vi "CAEN_HVChannel.ProcCases.vi"(0 "i ref in":refnum<vi>, 1 "selector":string, 2 "Data":T1, 3 "call cluster":T2={"Object"="", "Selector"="", "CallType"=enum."synchronous", "Async Object"="", "Async Selector"="", "Data Descriptor"="", "Data"=[], "Error #"=0, "Expire"=0}, 5 "error in (no error)":errorcluster) -> (14 "i ref out":refnum<vi>, 17 "answer cluster":T2={"Object"="", "Selector"="", "CallType"=enum."synchronous", "Async Object"="", "Async Selector"="", "Data Descriptor"="", "Data"=[], "Error #"=0, "Expire"=0}, 19 "error out":errorcluster)   [LabVIEW 2014, in "CAEN_HVChannel.lvlib"]
doc: "This method is called by a process from within the default case in the event loop. The methods of a class that are linked to events will be called from THIS method. Add your code here."
uses:
  CAEN_HVChannel.lvlib
  CS_Core/CSSystem/CoreDefs/CoreDefs.call_type.ctl
  CS_Core/BaseProcess/BaseProcess.descriptor string definition.ctl
  CS_Core/CSSystem/CoreDefs/CoreDefs.rawDataType.ctl
  CS_Core/CSApplicationBaseClasses/PSChannelBase/PSChannelBase.directionType.ctl
  CS_Core/CSApplicationBaseClasses/PSChannelBase/PSChannelBase.serviceType.ctl
  CS_Core/CSSystem/CoreDefs/CoreDefs.error_type.ctl
  CS_Core/CSSystem/CoreDefs/CoreDefs.error_severity.ctl
  CSlibraries/UtilityLib/UtilityLib.valueStatus.ctl
  CS_Core/CSSystem/CoreLib/CoreLib.byte array 2 double.vi
  CS_Core/CSSystem/CoreLib/CoreLib.string 2 byte array.vi
  CS_Core/CSSystem/CoreLib/CoreLib.double 2 byte array.vi
  CS_Core/CSSystem/CoreLib/CoreLib.short 2 byte array.vi
  CS_Core/CSSystem/CoreLib/CoreLib.byte array 2 short.vi
  CS_Core/CSSystem/CoreLib/CoreLib.byte array 2 int.vi
  CS_Core/CSSystem/CoreLib/CoreLib.byte array 2 string.vi
  CS_Core/CSSystem/CoreLib/CoreLib.lvlib
  CS_Core/BaseProcess/BaseProcess.lvlib
  CS_Core/CSApplicationBaseClasses/PSChannelBase/PSChannelBase.lvlib
  CS_Core/CAEObj/CAEObj.lvlib
  CS_Core/CSApplicationBaseClasses/DeviceBase/DeviceBase.lvlib
  CAEN_HVSystem/CAEN_HVSystem.lvlib
  CSlibraries/UtilityLib/UtilityLib.lvlib
  CSlibraries-extern/DimLVEvent/LVDimInterface/LVDimInterface.lvlib
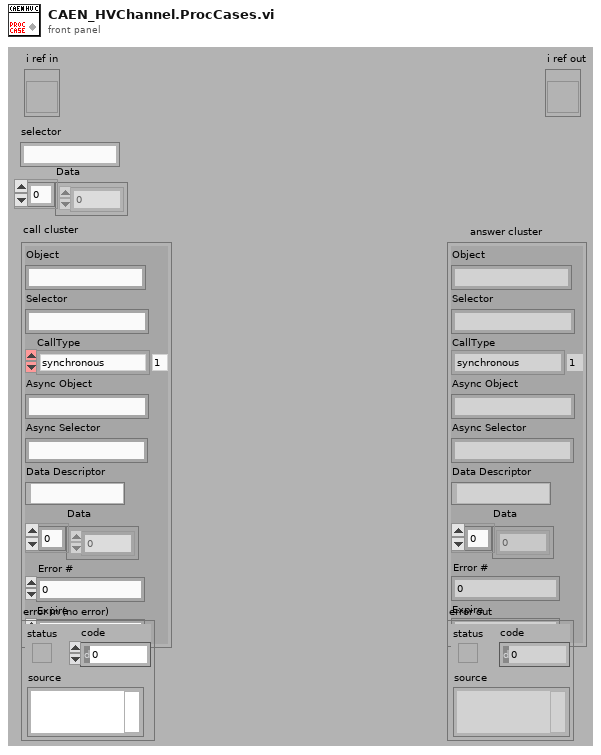
[diagram p1: front panel]
types:
  T1 = typedef "CoreDefs.rawDataType.ctl" = i8[]
  T2 = typedef "CoreDefs.call_type.ctl" = cluster{"Object":string, "Selector":string, "CallType":enum16{"simple", "synchronous", "asynchronous"}, "Async Object":string, "Async Selector":string, "Data Descriptor":T3, "Data":T1, "Error #":i32, "Expire":u32}
  T3 = typedef "BaseProcess.lvlib/BaseProcess.descriptor string definition.ctl" = string
  T4 = typedef "PSChannelBase.lvlib/PSChannelBase.serviceType.ctl" = enum16{"onOff", "voltage", "current", "tripCurrent", "rampUpSpeed", "rampDownSpeed", "status"}
  T5 = typedef "PSChannelBase.lvlib/PSChannelBase.directionType.ctl" = enum16{"unknown", "update actual value", "update nominal value", "update both"}
  T6 = typedef "CoreDefs.error_severity.ctl" = enum16{"undefined", "information", "warning", "error", "fatal"}
  T7 = typedef "CoreDefs.error_type.ctl" = enum16{"no error", "can't load process", "can't unload process", "process does not exist", "can't install process", "can't remove process", "unknown function", "time out", "can't execute function", "duplicate queue name", "super not found", "caller queue invalid", "can't ping process", "unknown error", "VISA Error", "VISA timeout", "GPIB timeout", "GPIB error", "communication error", "data type mismatch", "can't read data from OPC server", "can't write data to OPC server", "OET error", "function not implemented", "process already exists", "invalid Shared Variable name", "error writing Shared Variable", "error reading Shared Variable", "invalid client name", "corrupt database", "unknown class", "call not authorized", "parameter out of range", "OET timeout: can't get data to modify", "invalid queue name", "requested operation incompatible with current state", "event undefined", "event disabled", "state undefined", "caller is not a friend", "EventBuilder: bad eventID", "EventBuilder: no DAQ devices", "a thread must not stop itself", "UNUSED ELEMENT4", "DiscArchiver: eventData incomplete", "DiscArchiver: eventData does not belong to run", "DiscArchiver: can't open file", "DiscArchiver: can't write to file", "DiscArchiver: available disc space low", "can't acquire semaphore", "error reading data from database", "notifier object is not existing", "can't register process", "can't unregister process", "illegal event type", "object disabled", "object already exists", "can't change state", "Instrument not found", "no connection to remote node", "invalid reference", "N/A", "UNUSED ELEMENT 1", "element not found", "illegal TCP/IP connection detected", "object does not exist", "invalid access ID", "unknown CS system", "invalid privilige", "unsupported data type", "unsupported server type", "IO server already exists", "Shared Variable already exists"}
  T8 = typedef "UtilityLib.lvlib/UtilityLib.valueStatus.ctl" = enum16{"no info available", "stand by/off", "on", "warning", "alarm/malfunction", "not implemented", "user action required", "important information", "system default", "control default", "indicator default", "button default"}
  T9 = typedef "CAEN_HVChannel.lvlib/CAEN_HVChannel.i attribute.ctl" = cluster{"Channel Array":cluster{"Logical Name":string, "Address":string, "error in (no error)":errorcluster, "Name":cluster{"Name":string, "DIM Status":cluster{"no link":bool, "quality":i32, "Time Stamp":timestamp}}, "Status":cluster{"Status":i16, "DIM Status":cluster{"no link":bool, "quality":i32, "Time Stamp":timestamp}}, "V0Set":cluster{"V0Set#EU":cluster{"V0Set#EU":string, "DIM Status":cluster{"no link":bool, "quality":i32, "Time Stamp":timestamp}}, "V0Set":cluster{"V0Set":dbl, "DIM Status":cluster{"no link":bool, "quality":i32, "Time Stamp":timestamp}}, "V0Set#HighEU":cluster{"V0Set#HighEU":dbl, "DIM Status":cluster{"no link":bool, "quality":i32, "Time Stamp":timestamp}}, "V0Set#LowEU":cluster{"V0Set#LowEU":dbl, "DIM Status":cluster{"no link":bool, "quality":i32, "Time Stamp":timestamp}}, "V0Set#Multiplier":dbl}, "I0Set":cluster{"I0Set#EU":cluster{"I0Set#EU":string, "DIM Status":cluster{"no link":bool, "quality":i32, "Time Stamp":timestamp}}, "I0Set":cluster{"I0Set":dbl, "DIM Status":cluster{"no link":bool, "quality":i32, "Time Stamp":timestamp}}, "I0Set#HighEU":cluster{"I0Set#HighEU":dbl, "DIM Status":cluster{"no link":bool, "quality":i32, "Time Stamp":timestamp}}, "I0Set#LowEU":cluster{"I0Set#LowEU":dbl, "DIM Status":cluster{"no link":bool, "quality":i32, "Time Stamp":timestamp}}, "I0Set#Multiplier":dbl}, "V1Set":cluster{"V1Set#EU":cluster{"V1Set#EU":string, "DIM Status":cluster{"no link":bool, "quality":i32, "Time Stamp":timestamp}}, "V1Set":cluster{"V1Set":dbl, "DIM Status":cluster{"no link":bool, "quality":i32, "Time Stamp":timestamp}}, "V1Set#HighEU":cluster{"V1Set#HighEU":dbl, "DIM Status":cluster{"no link":bool, "quality":i32, "Time Stamp":timestamp}}, "V1Set#LowEU":cluster{"V1Set#LowEU":dbl, "DIM Status":cluster{"no link":bool, "quality":i32, "Time Stamp":timestamp}}, "V1Set#Multiplier":dbl}, "I1Set":cluster{"I1Set#EU":cluster{"I1Set#EU":string, "DIM Status":cluster{"no link":bool, "quality":i32, "Time Stamp":timestamp}}, "I1Set":cluster{"I1Set":dbl, "DIM Status":cluster{"no link":bool, "quality":i32, "Time Stamp":timestamp}}, "I1Set#HighEU":cluster{"I1Set#HighEU":dbl, "DIM Status":cluster{"no link":bool, "quality":i32, "Time Stamp":timestamp}}, "I1Set#LowEU":cluster{"I1Set#LowEU":dbl, "DIM Status":cluster{"no link":bool, "quality":i32, "Time Stamp":timestamp}}, "I1Set#Multiplier":dbl}, "RUp":cluster{"RUp#EU":cluster{"RUp#EU":string, "DIM Status":cluster{"no link":bool, "quality":i32, "Time Stamp":timestamp}}, "RUp":cluster{"RUp":dbl, "DIM Status":cluster{"no link":bool, "quality":i32, "Time Stamp":timestamp}}, "RUp#HighEU":cluster{"RUp#HighEU":dbl, "DIM Status":cluster{"no link":bool, "quality":i32, "Time Stamp":timestamp}}, "RUp#LowEU":cluster{"RUp#LowEU":dbl, "DIM Status":cluster{"no link":bool, "quality":i32, "Time Stamp":timestamp}}, "RUp#Multiplier":dbl}, "RDWn":cluster{"RDWn#EU":cluster{"RDWn#EU":string, "DIM Status":cluster{"no link":bool, "quality":i32, "Time Stamp":timestamp}}, "RDWn":cluster{"RDWn":dbl, "DIM Status":cluster{"no link":bool, "quality":i32, "Time Stamp":timestamp}}, "RDWn#HighEU":cluster{"RDWn#HighEU":dbl, "DIM Status":cluster{"no link":bool, "quality":i32, "Time Stamp":timestamp}}, "RDWn#LowEU":cluster{"RDWn#LowEU":dbl, "DIM Status":cluster{"no link":bool, "quality":i32, "Time Stamp":timestamp}}, "RDWn#Multiplier":dbl}, "Trip":cluster{"Trip#EU":cluster{"Trip#EU":string, "DIM Status":cluster{"no link":bool, "quality":i32, "Time Stamp":timestamp}}, "Trip":cluster{"Trip":dbl, "DIM Status":cluster{"no link":bool, "quality":i32, "Time Stamp":timestamp}}, "Trip#HighEU":cluster{"Trip#HighEU":dbl, "DIM Status":cluster{"no link":bool, "quality":i32, "Time Stamp":timestamp}}, "Trip#LowEU":cluster{"Trip#LowEU":dbl, "DIM Status":cluster{"no link":bool, "quality":i32, "Time Stamp":timestamp}}, "Trip#Multiplier":dbl}, "SVMax":cluster{"SVMax#EU":cluster{"SVMax#EU":string, "DIM Status":cluster{"no link":bool, "quality":i32, "Time Stamp":timestamp}}, "SVMax":cluster{"SVMax":dbl, "DIM Status":cluster{"no link":bool, "quality":i32, "Time Stamp":timestamp}}, "SVMax#HighEU":cluster{"SVMax#HighEU":dbl, "DIM Status":cluster{"no link":bool, "quality":i32, "Time Stamp":timestamp}}, "SVMax#LowEU":cluster{"SVMax#LowEU":dbl, "DIM Status":cluster{"no link":bool, "quality":i32, "Time Stamp":timestamp}}, "SVMax#Multiplier":dbl}, "VMon":cluster{"VMon#EU":cluster{"VMon#EU":string, "DIM Status":cluster{"no link":bool, "quality":i32, "Time Stamp":timestamp}}, "VMon":cluster{"VMon":dbl, "DIM Status":cluster{"no link":bool, "quality":i32, "Time Stamp":timestamp}}, "VMon#HighEU":cluster{"VMon#HighEU":dbl, "DIM Status":cluster{"no link":bool, "quality":i32, "Time Stamp":timestamp}}, "VMon#LowEU":cluster{"VMon#LowEU":dbl, "DIM Status":cluster{"no link":bool, "quality":i32, "Time Stamp":timestamp}}, "VMon#Multiplier":dbl}, "IMon":cluster{"IMon#EU":cluster{"IMon#EU":string, "DIM Status":cluster{"no link":bool, "quality":i32, "Time Stamp":timestamp}}, "IMon":cluster{"IMon":dbl, "DIM Status":cluster{"no link":bool, "quality":i32, "Time Stamp":timestamp}}, "IMon#HighEU":cluster{"IMon#HighEU":dbl, "DIM Status":cluster{"no link":bool, "quality":i32, "Time Stamp":timestamp}}, "IMon#LowEU":cluster{"IMon#LowEU":dbl, "DIM Status":cluster{"no link":bool, "quality":i32, "Time Stamp":timestamp}}, "IMon#Multiplier":dbl}, "TripInt":cluster{"TripInt#EU":cluster{"TripInt#EU":string, "DIM Status":cluster{"no link":bool, "quality":i32, "Time Stamp":timestamp}}, "TripInt":cluster{"TripInt":dbl, "DIM Status":cluster{"no link":bool, "quality":i32, "Time Stamp":timestamp}}, "TripInt#HighEU":cluster{"TripInt#HighEU":dbl, "DIM Status":cluster{"no link":bool, "quality":i32, "Time Stamp":timestamp}}, "TripInt#LowEU":cluster{"TripInt#LowEU":dbl, "DIM Status":cluster{"no link":bool, "quality":i32, "Time Stamp":timestamp}}, "TripInt#Multiplier":dbl}, "TripExt":cluster{"TripExt#EU":cluster{"TripExt#EU":string, "DIM Status":cluster{"no link":bool, "quality":i32, "Time Stamp":timestamp}}, "TripExt":cluster{"TripExt":dbl, "DIM Status":cluster{"no link":bool, "quality":i32, "Time Stamp":timestamp}}, "TripExt#HighEU":cluster{"TripExt#HighEU":dbl, "DIM Status":cluster{"no link":bool, "quality":i32, "Time Stamp":timestamp}}, "TripExt#LowEU":cluster{"TripExt#LowEU":dbl, "DIM Status":cluster{"no link":bool, "quality":i32, "Time Stamp":timestamp}}, "TripExt#Multiplier":dbl}, "Pw":cluster{"Pw":cluster{"Pw":bool, "DIM Status":cluster{"no link":bool, "quality":i32, "Time Stamp":timestamp}}, "Pw#CoClose":cluster{"Pw#CoClose":string, "DIM Status":cluster{"no link":bool, "quality":i32, "Time Stamp":timestamp}}, "Pw#CoOpen":cluster{"Pw#CoOpen":string, "DIM Status":cluster{"no link":bool, "quality":i32, "Time Stamp":timestamp}}}, "POn":cluster{"POn":cluster{"POn":bool, "DIM Status":cluster{"no link":bool, "quality":i32, "Time Stamp":timestamp}}, "POn#CoClose":cluster{"POn#CoClose":string, "DIM Status":cluster{"no link":bool, "quality":i32, "Time Stamp":timestamp}}, "POn#CoOpen":cluster{"POn#CoOpen":string, "DIM Status":cluster{"no link":bool, "quality":i32, "Time Stamp":timestamp}}}, "PDwn":cluster{"PDwn":cluster{"PDwn":bool, "DIM Status":cluster{"no link":bool, "quality":i32, "Time Stamp":timestamp}}, "PDwn#CoClose":cluster{"PDwn#CoClose":string, "DIM Status":cluster{"no link":bool, "quality":i32, "Time Stamp":timestamp}}, "PDwn#CoOpen":cluster{"PDwn#CoOpen":string, "DIM Status":cluster{"no link":bool, "quality":i32, "Time Stamp":timestamp}}}, "DIM Service IDs":cluster{"nomV1Set":i32, "nomI1Set":i32, "nomTrip":i32, "nomSVMax":i32, "nomPOn":i32, "nomPDwn":i32, "nomTripInt":i32, "nomTripExt":i32}}[], "VoltageInRangeBand":dbl}
  T10 = cluster{"Logical Name":string, "Address":string, "error in (no error)":errorcluster, "Name":cluster{"Name":string, "DIM Status":cluster{"no link":bool, "quality":i32, "Time Stamp":timestamp}}, "Status":cluster{"Status":i16, "DIM Status":cluster{"no link":bool, "quality":i32, "Time Stamp":timestamp}}, "V0Set":cluster{"V0Set#EU":cluster{"V0Set#EU":string, "DIM Status":cluster{"no link":bool, "quality":i32, "Time Stamp":timestamp}}, "V0Set":cluster{"V0Set":dbl, "DIM Status":cluster{"no link":bool, "quality":i32, "Time Stamp":timestamp}}, "V0Set#HighEU":cluster{"V0Set#HighEU":dbl, "DIM Status":cluster{"no link":bool, "quality":i32, "Time Stamp":timestamp}}, "V0Set#LowEU":cluster{"V0Set#LowEU":dbl, "DIM Status":cluster{"no link":bool, "quality":i32, "Time Stamp":timestamp}}, "V0Set#Multiplier":dbl}, "I0Set":cluster{"I0Set#EU":cluster{"I0Set#EU":string, "DIM Status":cluster{"no link":bool, "quality":i32, "Time Stamp":timestamp}}, "I0Set":cluster{"I0Set":dbl, "DIM Status":cluster{"no link":bool, "quality":i32, "Time Stamp":timestamp}}, "I0Set#HighEU":cluster{"I0Set#HighEU":dbl, "DIM Status":cluster{"no link":bool, "quality":i32, "Time Stamp":timestamp}}, "I0Set#LowEU":cluster{"I0Set#LowEU":dbl, "DIM Status":cluster{"no link":bool, "quality":i32, "Time Stamp":timestamp}}, "I0Set#Multiplier":dbl}, "V1Set":cluster{"V1Set#EU":cluster{"V1Set#EU":string, "DIM Status":cluster{"no link":bool, "quality":i32, "Time Stamp":timestamp}}, "V1Set":cluster{"V1Set":dbl, "DIM Status":cluster{"no link":bool, "quality":i32, "Time Stamp":timestamp}}, "V1Set#HighEU":cluster{"V1Set#HighEU":dbl, "DIM Status":cluster{"no link":bool, "quality":i32, "Time Stamp":timestamp}}, "V1Set#LowEU":cluster{"V1Set#LowEU":dbl, "DIM Status":cluster{"no link":bool, "quality":i32, "Time Stamp":timestamp}}, "V1Set#Multiplier":dbl}, "I1Set":cluster{"I1Set#EU":cluster{"I1Set#EU":string, "DIM Status":cluster{"no link":bool, "quality":i32, "Time Stamp":timestamp}}, "I1Set":cluster{"I1Set":dbl, "DIM Status":cluster{"no link":bool, "quality":i32, "Time Stamp":timestamp}}, "I1Set#HighEU":cluster{"I1Set#HighEU":dbl, "DIM Status":cluster{"no link":bool, "quality":i32, "Time Stamp":timestamp}}, "I1Set#LowEU":cluster{"I1Set#LowEU":dbl, "DIM Status":cluster{"no link":bool, "quality":i32, "Time Stamp":timestamp}}, "I1Set#Multiplier":dbl}, "RUp":cluster{"RUp#EU":cluster{"RUp#EU":string, "DIM Status":cluster{"no link":bool, "quality":i32, "Time Stamp":timestamp}}, "RUp":cluster{"RUp":dbl, "DIM Status":cluster{"no link":bool, "quality":i32, "Time Stamp":timestamp}}, "RUp#HighEU":cluster{"RUp#HighEU":dbl, "DIM Status":cluster{"no link":bool, "quality":i32, "Time Stamp":timestamp}}, "RUp#LowEU":cluster{"RUp#LowEU":dbl, "DIM Status":cluster{"no link":bool, "quality":i32, "Time Stamp":timestamp}}, "RUp#Multiplier":dbl}, "RDWn":cluster{"RDWn#EU":cluster{"RDWn#EU":string, "DIM Status":cluster{"no link":bool, "quality":i32, "Time Stamp":timestamp}}, "RDWn":cluster{"RDWn":dbl, "DIM Status":cluster{"no link":bool, "quality":i32, "Time Stamp":timestamp}}, "RDWn#HighEU":cluster{"RDWn#HighEU":dbl, "DIM Status":cluster{"no link":bool, "quality":i32, "Time Stamp":timestamp}}, "RDWn#LowEU":cluster{"RDWn#LowEU":dbl, "DIM Status":cluster{"no link":bool, "quality":i32, "Time Stamp":timestamp}}, "RDWn#Multiplier":dbl}, "Trip":cluster{"Trip#EU":cluster{"Trip#EU":string, "DIM Status":cluster{"no link":bool, "quality":i32, "Time Stamp":timestamp}}, "Trip":cluster{"Trip":dbl, "DIM Status":cluster{"no link":bool, "quality":i32, "Time Stamp":timestamp}}, "Trip#HighEU":cluster{"Trip#HighEU":dbl, "DIM Status":cluster{"no link":bool, "quality":i32, "Time Stamp":timestamp}}, "Trip#LowEU":cluster{"Trip#LowEU":dbl, "DIM Status":cluster{"no link":bool, "quality":i32, "Time Stamp":timestamp}}, "Trip#Multiplier":dbl}, "SVMax":cluster{"SVMax#EU":cluster{"SVMax#EU":string, "DIM Status":cluster{"no link":bool, "quality":i32, "Time Stamp":timestamp}}, "SVMax":cluster{"SVMax":dbl, "DIM Status":cluster{"no link":bool, "quality":i32, "Time Stamp":timestamp}}, "SVMax#HighEU":cluster{"SVMax#HighEU":dbl, "DIM Status":cluster{"no link":bool, "quality":i32, "Time Stamp":timestamp}}, "SVMax#LowEU":cluster{"SVMax#LowEU":dbl, "DIM Status":cluster{"no link":bool, "quality":i32, "Time Stamp":timestamp}}, "SVMax#Multiplier":dbl}, "VMon":cluster{"VMon#EU":cluster{"VMon#EU":string, "DIM Status":cluster{"no link":bool, "quality":i32, "Time Stamp":timestamp}}, "VMon":cluster{"VMon":dbl, "DIM Status":cluster{"no link":bool, "quality":i32, "Time Stamp":timestamp}}, "VMon#HighEU":cluster{"VMon#HighEU":dbl, "DIM Status":cluster{"no link":bool, "quality":i32, "Time Stamp":timestamp}}, "VMon#LowEU":cluster{"VMon#LowEU":dbl, "DIM Status":cluster{"no link":bool, "quality":i32, "Time Stamp":timestamp}}, "VMon#Multiplier":dbl}, "IMon":cluster{"IMon#EU":cluster{"IMon#EU":string, "DIM Status":cluster{"no link":bool, "quality":i32, "Time Stamp":timestamp}}, "IMon":cluster{"IMon":dbl, "DIM Status":cluster{"no link":bool, "quality":i32, "Time Stamp":timestamp}}, "IMon#HighEU":cluster{"IMon#HighEU":dbl, "DIM Status":cluster{"no link":bool, "quality":i32, "Time Stamp":timestamp}}, "IMon#LowEU":cluster{"IMon#LowEU":dbl, "DIM Status":cluster{"no link":bool, "quality":i32, "Time Stamp":timestamp}}, "IMon#Multiplier":dbl}, "TripInt":cluster{"TripInt#EU":cluster{"TripInt#EU":string, "DIM Status":cluster{"no link":bool, "quality":i32, "Time Stamp":timestamp}}, "TripInt":cluster{"TripInt":dbl, "DIM Status":cluster{"no link":bool, "quality":i32, "Time Stamp":timestamp}}, "TripInt#HighEU":cluster{"TripInt#HighEU":dbl, "DIM Status":cluster{"no link":bool, "quality":i32, "Time Stamp":timestamp}}, "TripInt#LowEU":cluster{"TripInt#LowEU":dbl, "DIM Status":cluster{"no link":bool, "quality":i32, "Time Stamp":timestamp}}, "TripInt#Multiplier":dbl}, "TripExt":cluster{"TripExt#EU":cluster{"TripExt#EU":string, "DIM Status":cluster{"no link":bool, "quality":i32, "Time Stamp":timestamp}}, "TripExt":cluster{"TripExt":dbl, "DIM Status":cluster{"no link":bool, "quality":i32, "Time Stamp":timestamp}}, "TripExt#HighEU":cluster{"TripExt#HighEU":dbl, "DIM Status":cluster{"no link":bool, "quality":i32, "Time Stamp":timestamp}}, "TripExt#LowEU":cluster{"TripExt#LowEU":dbl, "DIM Status":cluster{"no link":bool, "quality":i32, "Time Stamp":timestamp}}, "TripExt#Multiplier":dbl}, "Pw":cluster{"Pw":cluster{"Pw":bool, "DIM Status":cluster{"no link":bool, "quality":i32, "Time Stamp":timestamp}}, "Pw#CoClose":cluster{"Pw#CoClose":string, "DIM Status":cluster{"no link":bool, "quality":i32, "Time Stamp":timestamp}}, "Pw#CoOpen":cluster{"Pw#CoOpen":string, "DIM Status":cluster{"no link":bool, "quality":i32, "Time Stamp":timestamp}}}, "POn":cluster{"POn":cluster{"POn":bool, "DIM Status":cluster{"no link":bool, "quality":i32, "Time Stamp":timestamp}}, "POn#CoClose":cluster{"POn#CoClose":string, "DIM Status":cluster{"no link":bool, "quality":i32, "Time Stamp":timestamp}}, "POn#CoOpen":cluster{"POn#CoOpen":string, "DIM Status":cluster{"no link":bool, "quality":i32, "Time Stamp":timestamp}}}, "PDwn":cluster{"PDwn":cluster{"PDwn":bool, "DIM Status":cluster{"no link":bool, "quality":i32, "Time Stamp":timestamp}}, "PDwn#CoClose":cluster{"PDwn#CoClose":string, "DIM Status":cluster{"no link":bool, "quality":i32, "Time Stamp":timestamp}}, "PDwn#CoOpen":cluster{"PDwn#CoOpen":string, "DIM Status":cluster{"no link":bool, "quality":i32, "Time Stamp":timestamp}}}, "DIM Service IDs":cluster{"nomV1Set":i32, "nomI1Set":i32, "nomTrip":i32, "nomSVMax":i32, "nomPOn":i32, "nomPDwn":i32, "nomTripInt":i32, "nomTripExt":i32}}[]
  T11 = cluster{"Logical Name":string, "Address":string, "error in (no error)":errorcluster, "Name":cluster{"Name":string, "DIM Status":cluster{"no link":bool, "quality":i32, "Time Stamp":timestamp}}, "Status":cluster{"Status":i16, "DIM Status":cluster{"no link":bool, "quality":i32, "Time Stamp":timestamp}}, "V0Set":cluster{"V0Set#EU":cluster{"V0Set#EU":string, "DIM Status":cluster{"no link":bool, "quality":i32, "Time Stamp":timestamp}}, "V0Set":cluster{"V0Set":dbl, "DIM Status":cluster{"no link":bool, "quality":i32, "Time Stamp":timestamp}}, "V0Set#HighEU":cluster{"V0Set#HighEU":dbl, "DIM Status":cluster{"no link":bool, "quality":i32, "Time Stamp":timestamp}}, "V0Set#LowEU":cluster{"V0Set#LowEU":dbl, "DIM Status":cluster{"no link":bool, "quality":i32, "Time Stamp":timestamp}}, "V0Set#Multiplier":dbl}, "I0Set":cluster{"I0Set#EU":cluster{"I0Set#EU":string, "DIM Status":cluster{"no link":bool, "quality":i32, "Time Stamp":timestamp}}, "I0Set":cluster{"I0Set":dbl, "DIM Status":cluster{"no link":bool, "quality":i32, "Time Stamp":timestamp}}, "I0Set#HighEU":cluster{"I0Set#HighEU":dbl, "DIM Status":cluster{"no link":bool, "quality":i32, "Time Stamp":timestamp}}, "I0Set#LowEU":cluster{"I0Set#LowEU":dbl, "DIM Status":cluster{"no link":bool, "quality":i32, "Time Stamp":timestamp}}, "I0Set#Multiplier":dbl}, "V1Set":cluster{"V1Set#EU":cluster{"V1Set#EU":string, "DIM Status":cluster{"no link":bool, "quality":i32, "Time Stamp":timestamp}}, "V1Set":cluster{"V1Set":dbl, "DIM Status":cluster{"no link":bool, "quality":i32, "Time Stamp":timestamp}}, "V1Set#HighEU":cluster{"V1Set#HighEU":dbl, "DIM Status":cluster{"no link":bool, "quality":i32, "Time Stamp":timestamp}}, "V1Set#LowEU":cluster{"V1Set#LowEU":dbl, "DIM Status":cluster{"no link":bool, "quality":i32, "Time Stamp":timestamp}}, "V1Set#Multiplier":dbl}, "I1Set":cluster{"I1Set#EU":cluster{"I1Set#EU":string, "DIM Status":cluster{"no link":bool, "quality":i32, "Time Stamp":timestamp}}, "I1Set":cluster{"I1Set":dbl, "DIM Status":cluster{"no link":bool, "quality":i32, "Time Stamp":timestamp}}, "I1Set#HighEU":cluster{"I1Set#HighEU":dbl, "DIM Status":cluster{"no link":bool, "quality":i32, "Time Stamp":timestamp}}, "I1Set#LowEU":cluster{"I1Set#LowEU":dbl, "DIM Status":cluster{"no link":bool, "quality":i32, "Time Stamp":timestamp}}, "I1Set#Multiplier":dbl}, "RUp":cluster{"RUp#EU":cluster{"RUp#EU":string, "DIM Status":cluster{"no link":bool, "quality":i32, "Time Stamp":timestamp}}, "RUp":cluster{"RUp":dbl, "DIM Status":cluster{"no link":bool, "quality":i32, "Time Stamp":timestamp}}, "RUp#HighEU":cluster{"RUp#HighEU":dbl, "DIM Status":cluster{"no link":bool, "quality":i32, "Time Stamp":timestamp}}, "RUp#LowEU":cluster{"RUp#LowEU":dbl, "DIM Status":cluster{"no link":bool, "quality":i32, "Time Stamp":timestamp}}, "RUp#Multiplier":dbl}, "RDWn":cluster{"RDWn#EU":cluster{"RDWn#EU":string, "DIM Status":cluster{"no link":bool, "quality":i32, "Time Stamp":timestamp}}, "RDWn":cluster{"RDWn":dbl, "DIM Status":cluster{"no link":bool, "quality":i32, "Time Stamp":timestamp}}, "RDWn#HighEU":cluster{"RDWn#HighEU":dbl, "DIM Status":cluster{"no link":bool, "quality":i32, "Time Stamp":timestamp}}, "RDWn#LowEU":cluster{"RDWn#LowEU":dbl, "DIM Status":cluster{"no link":bool, "quality":i32, "Time Stamp":timestamp}}, "RDWn#Multiplier":dbl}, "Trip":cluster{"Trip#EU":cluster{"Trip#EU":string, "DIM Status":cluster{"no link":bool, "quality":i32, "Time Stamp":timestamp}}, "Trip":cluster{"Trip":dbl, "DIM Status":cluster{"no link":bool, "quality":i32, "Time Stamp":timestamp}}, "Trip#HighEU":cluster{"Trip#HighEU":dbl, "DIM Status":cluster{"no link":bool, "quality":i32, "Time Stamp":timestamp}}, "Trip#LowEU":cluster{"Trip#LowEU":dbl, "DIM Status":cluster{"no link":bool, "quality":i32, "Time Stamp":timestamp}}, "Trip#Multiplier":dbl}, "SVMax":cluster{"SVMax#EU":cluster{"SVMax#EU":string, "DIM Status":cluster{"no link":bool, "quality":i32, "Time Stamp":timestamp}}, "SVMax":cluster{"SVMax":dbl, "DIM Status":cluster{"no link":bool, "quality":i32, "Time Stamp":timestamp}}, "SVMax#HighEU":cluster{"SVMax#HighEU":dbl, "DIM Status":cluster{"no link":bool, "quality":i32, "Time Stamp":timestamp}}, "SVMax#LowEU":cluster{"SVMax#LowEU":dbl, "DIM Status":cluster{"no link":bool, "quality":i32, "Time Stamp":timestamp}}, "SVMax#Multiplier":dbl}, "VMon":cluster{"VMon#EU":cluster{"VMon#EU":string, "DIM Status":cluster{"no link":bool, "quality":i32, "Time Stamp":timestamp}}, "VMon":cluster{"VMon":dbl, "DIM Status":cluster{"no link":bool, "quality":i32, "Time Stamp":timestamp}}, "VMon#HighEU":cluster{"VMon#HighEU":dbl, "DIM Status":cluster{"no link":bool, "quality":i32, "Time Stamp":timestamp}}, "VMon#LowEU":cluster{"VMon#LowEU":dbl, "DIM Status":cluster{"no link":bool, "quality":i32, "Time Stamp":timestamp}}, "VMon#Multiplier":dbl}, "IMon":cluster{"IMon#EU":cluster{"IMon#EU":string, "DIM Status":cluster{"no link":bool, "quality":i32, "Time Stamp":timestamp}}, "IMon":cluster{"IMon":dbl, "DIM Status":cluster{"no link":bool, "quality":i32, "Time Stamp":timestamp}}, "IMon#HighEU":cluster{"IMon#HighEU":dbl, "DIM Status":cluster{"no link":bool, "quality":i32, "Time Stamp":timestamp}}, "IMon#LowEU":cluster{"IMon#LowEU":dbl, "DIM Status":cluster{"no link":bool, "quality":i32, "Time Stamp":timestamp}}, "IMon#Multiplier":dbl}, "TripInt":cluster{"TripInt#EU":cluster{"TripInt#EU":string, "DIM Status":cluster{"no link":bool, "quality":i32, "Time Stamp":timestamp}}, "TripInt":cluster{"TripInt":dbl, "DIM Status":cluster{"no link":bool, "quality":i32, "Time Stamp":timestamp}}, "TripInt#HighEU":cluster{"TripInt#HighEU":dbl, "DIM Status":cluster{"no link":bool, "quality":i32, "Time Stamp":timestamp}}, "TripInt#LowEU":cluster{"TripInt#LowEU":dbl, "DIM Status":cluster{"no link":bool, "quality":i32, "Time Stamp":timestamp}}, "TripInt#Multiplier":dbl}, "TripExt":cluster{"TripExt#EU":cluster{"TripExt#EU":string, "DIM Status":cluster{"no link":bool, "quality":i32, "Time Stamp":timestamp}}, "TripExt":cluster{"TripExt":dbl, "DIM Status":cluster{"no link":bool, "quality":i32, "Time Stamp":timestamp}}, "TripExt#HighEU":cluster{"TripExt#HighEU":dbl, "DIM Status":cluster{"no link":bool, "quality":i32, "Time Stamp":timestamp}}, "TripExt#LowEU":cluster{"TripExt#LowEU":dbl, "DIM Status":cluster{"no link":bool, "quality":i32, "Time Stamp":timestamp}}, "TripExt#Multiplier":dbl}, "Pw":cluster{"Pw":cluster{"Pw":bool, "DIM Status":cluster{"no link":bool, "quality":i32, "Time Stamp":timestamp}}, "Pw#CoClose":cluster{"Pw#CoClose":string, "DIM Status":cluster{"no link":bool, "quality":i32, "Time Stamp":timestamp}}, "Pw#CoOpen":cluster{"Pw#CoOpen":string, "DIM Status":cluster{"no link":bool, "quality":i32, "Time Stamp":timestamp}}}, "POn":cluster{"POn":cluster{"POn":bool, "DIM Status":cluster{"no link":bool, "quality":i32, "Time Stamp":timestamp}}, "POn#CoClose":cluster{"POn#CoClose":string, "DIM Status":cluster{"no link":bool, "quality":i32, "Time Stamp":timestamp}}, "POn#CoOpen":cluster{"POn#CoOpen":string, "DIM Status":cluster{"no link":bool, "quality":i32, "Time Stamp":timestamp}}}, "PDwn":cluster{"PDwn":cluster{"PDwn":bool, "DIM Status":cluster{"no link":bool, "quality":i32, "Time Stamp":timestamp}}, "PDwn#CoClose":cluster{"PDwn#CoClose":string, "DIM Status":cluster{"no link":bool, "quality":i32, "Time Stamp":timestamp}}, "PDwn#CoOpen":cluster{"PDwn#CoOpen":string, "DIM Status":cluster{"no link":bool, "quality":i32, "Time Stamp":timestamp}}}, "DIM Service IDs":cluster{"nomV1Set":i32, "nomI1Set":i32, "nomTrip":i32, "nomSVMax":i32, "nomPOn":i32, "nomPDwn":i32, "nomTripInt":i32, "nomTripExt":i32}}
  T12 = typedef "BaseProcess.lvlib/BaseProcess.i attribute.ctl" = cluster{"EventStatus":string, "EventError":i32, "PresetEvtWatchD":i32, "PresetPdcWatchD":i32, "EventTimeout":i32, "PeriodicInterval":i32, "Interface":string[], "Address":string[], "Special":string[], "PeriodicError":i32, "PeriodicStatus":string, "SuperProc":string, "Descriptors":T13[], "CaseRef":refnum<vi>, "PdcRef":refnum<vi>, "Thread Ref":refnum<vi>, "eventErrorID":i32, "eventStatusID":i32, "periodicErrorID":i32, "periodicStatusID":i32, "pdcCtrID":i32}
  T13 = typedef "BaseProcess.lvlib/BaseProcess.descriptor definition.ctl" = cluster{"selector":string, "descriptor":T3}
  T14 = typedef "PSChannelBase.lvlib/PSChannelBase.i attribute.ctl" = cluster{"defaultChannelIndex":i32, "nofChannels":i32, "defaultChannelIndexID":i32, "nofChannelsID":i32, "actValues":T15, "nomValues":T15, "logicalName":string[], "physicalName":string[], "logicalNameID":i32, "physicalNameID":i32}
  T15 = typedef "PSChannelBase.lvlib/PSChannelBase.parameters.ctl" = cluster{"onOff":bool[], "voltage":dbl[], "current":dbl[], "tripCurrent":dbl[], "rampUpSpeed":dbl[], "rampDownSpeed":dbl[], "status":i32[], "serviceIDs":cluster{"onOfflID":i32, "voltageID":i32, "currentID":i32, "tripCurrentID":i32, "rampUpSpeedID":i32, "rampDownSpeedID":i32, "statusID":i32}}
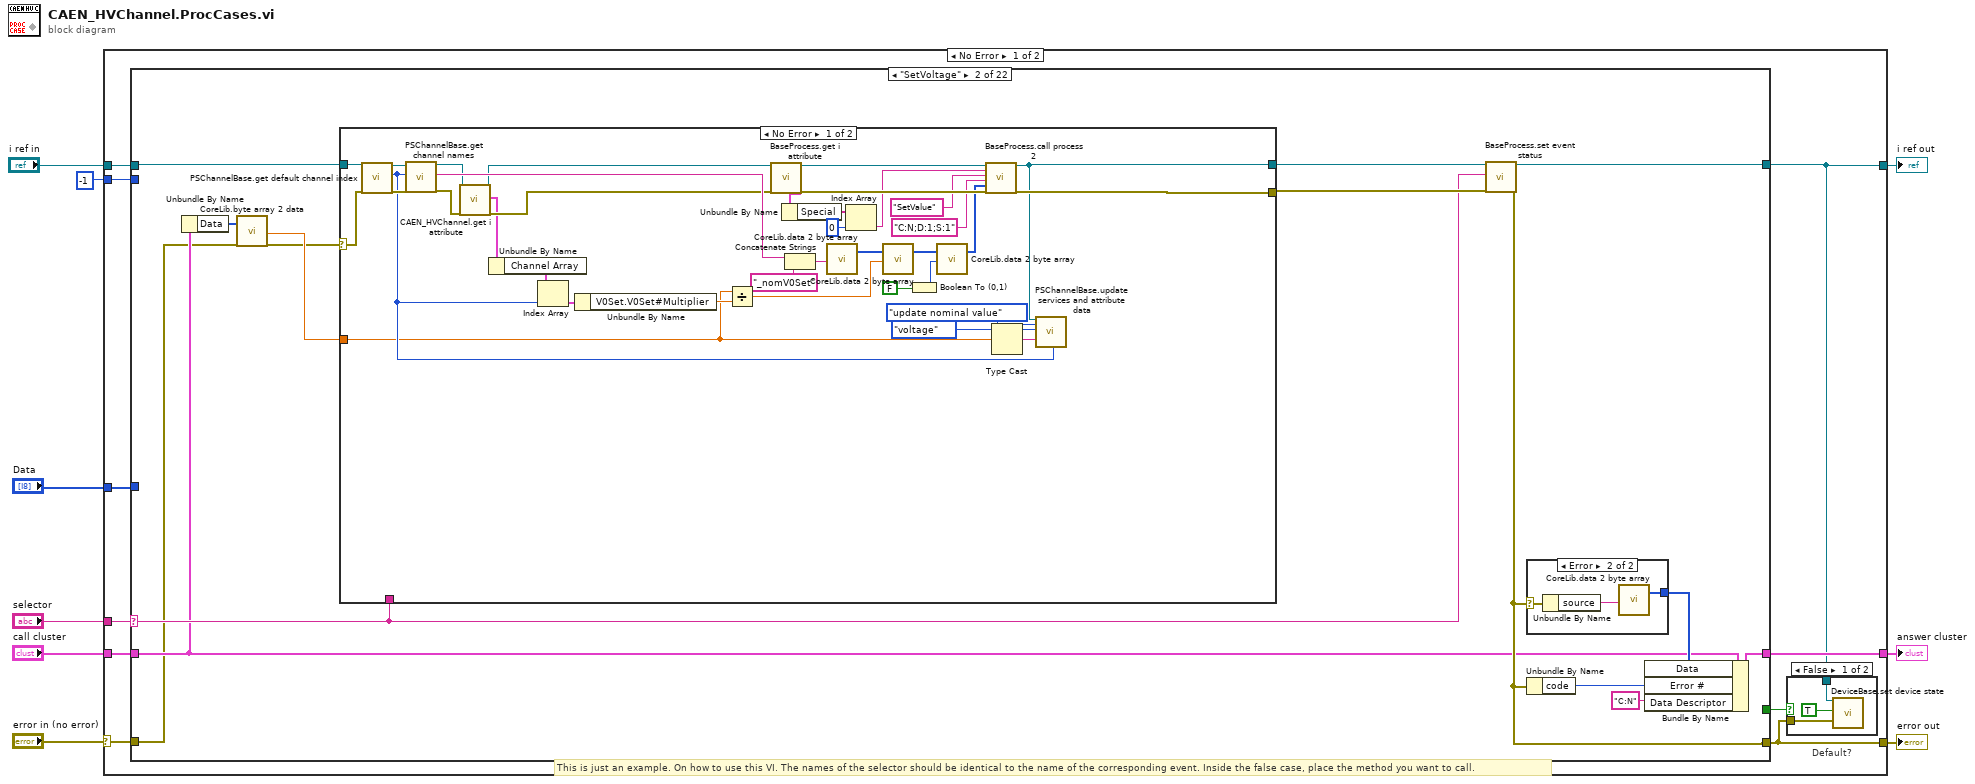
[diagram p0: block diagram]
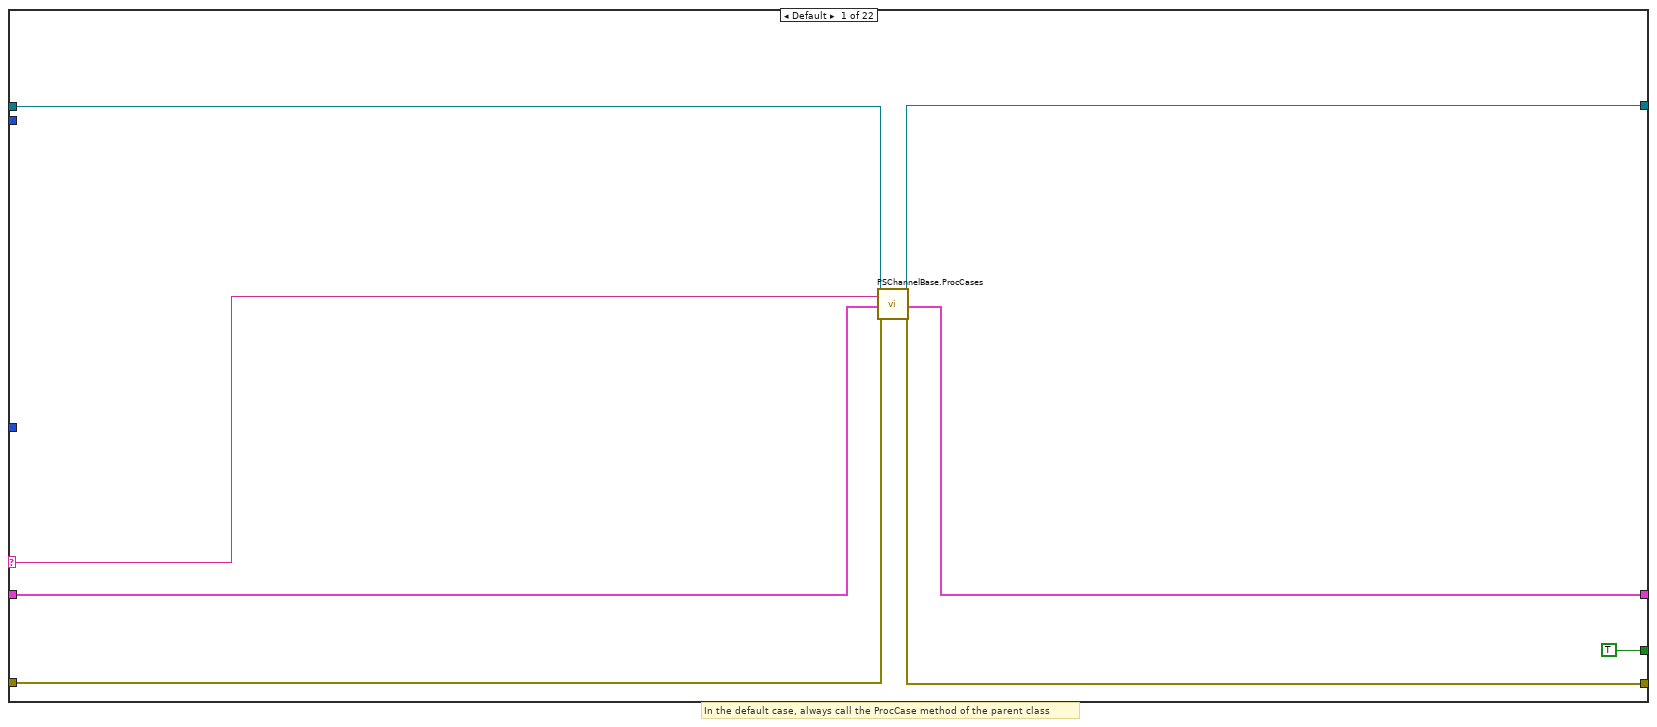
[diagram p3: hidden frame]
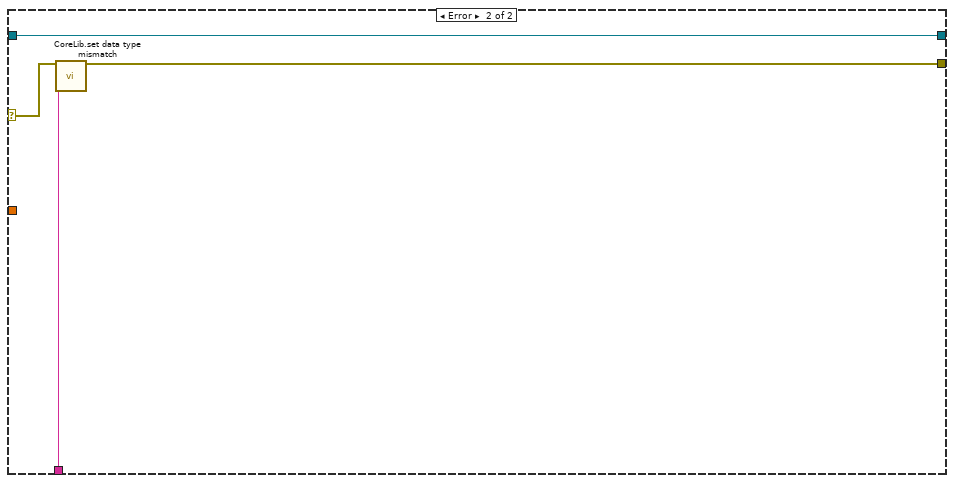
[diagram p5: hidden frame]
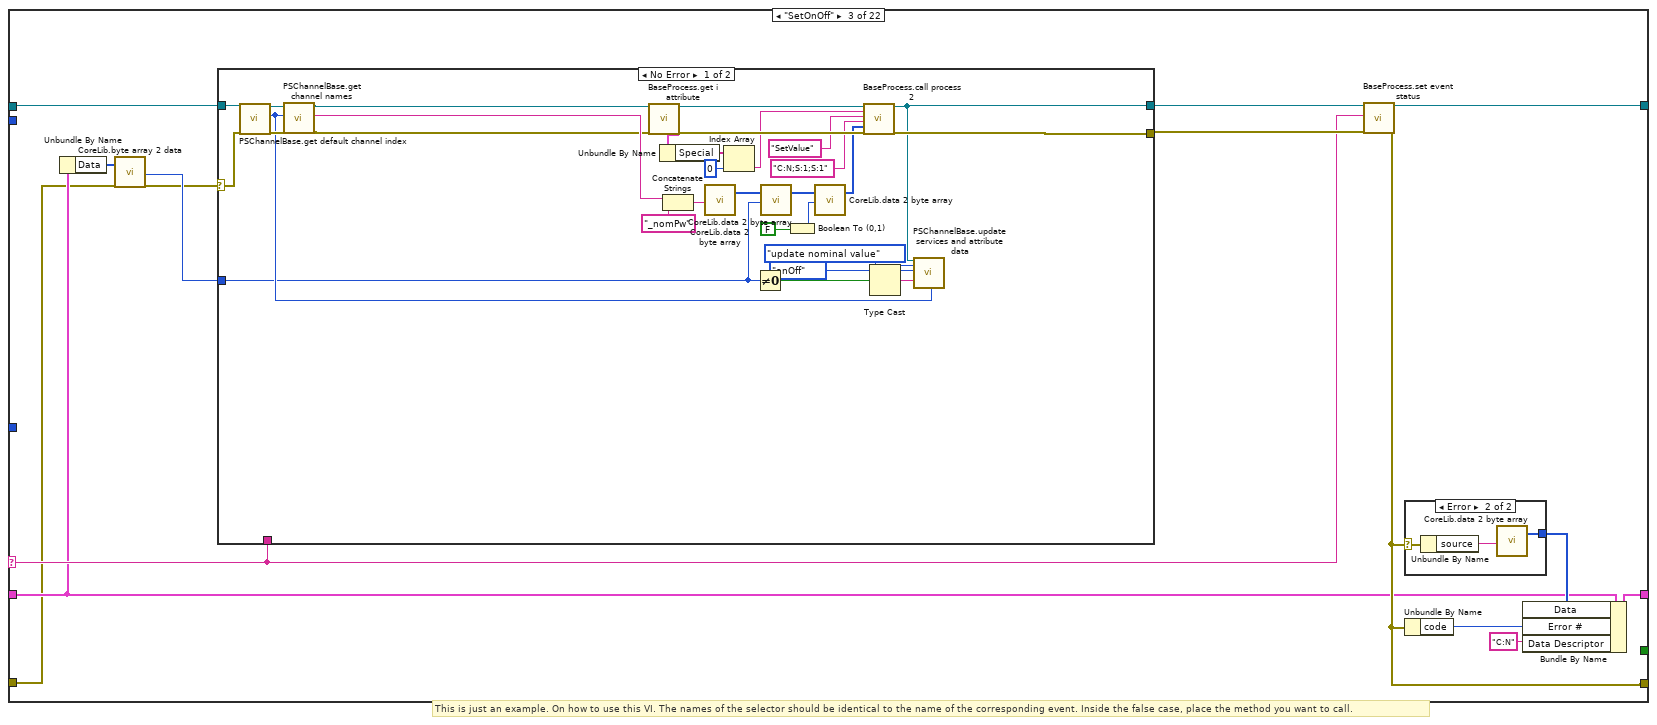
[diagram p6: hidden frame]
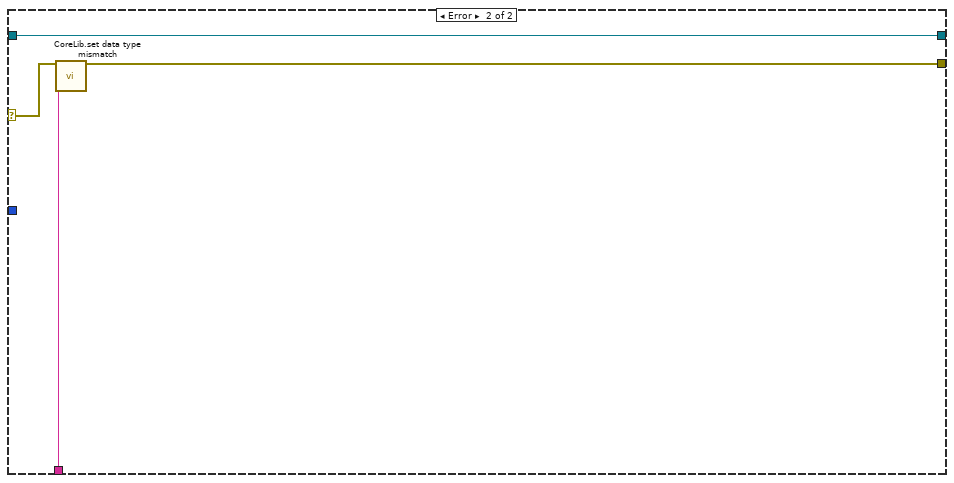
[diagram p8: hidden frame]
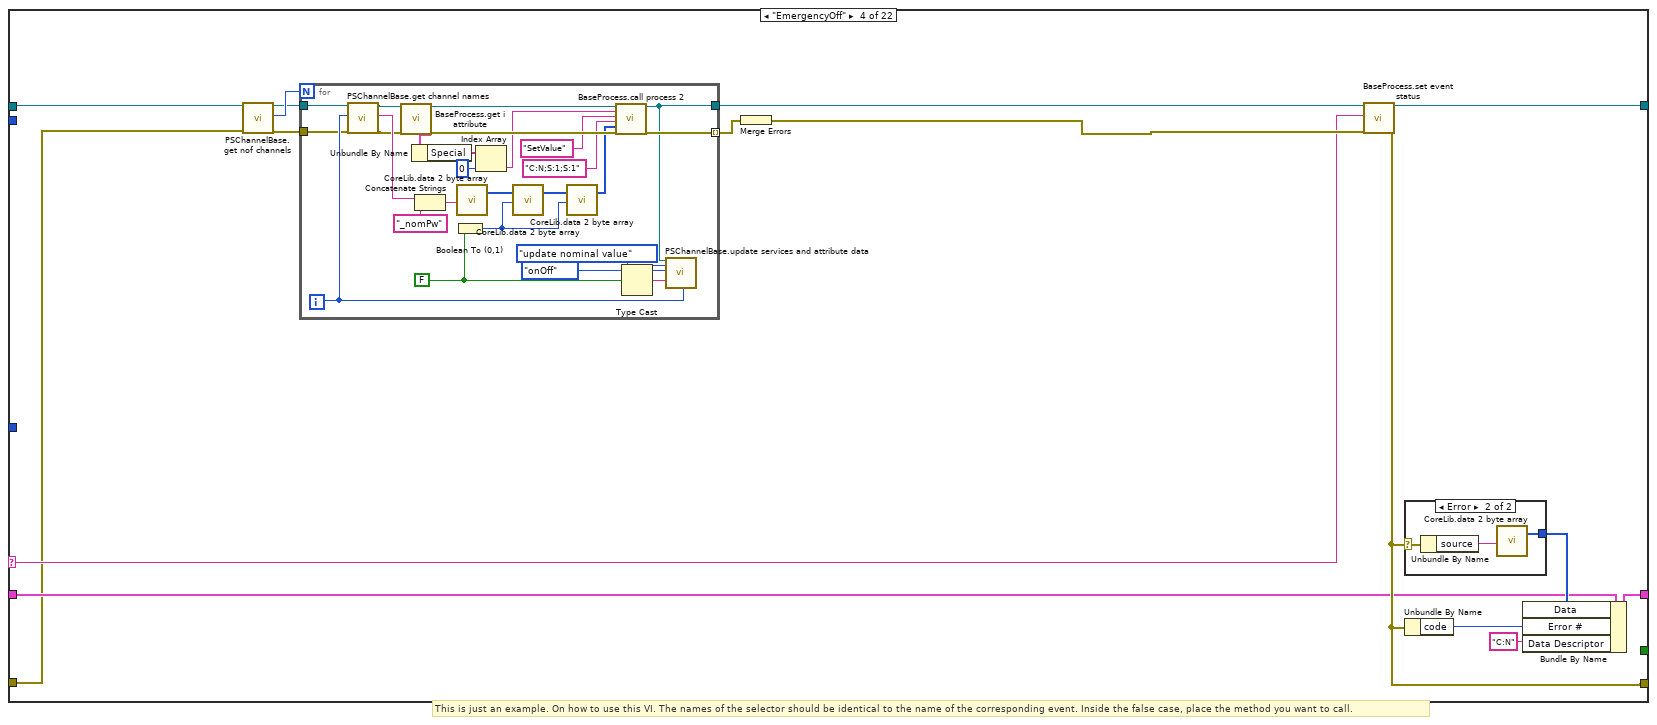
[diagram p9: hidden frame]
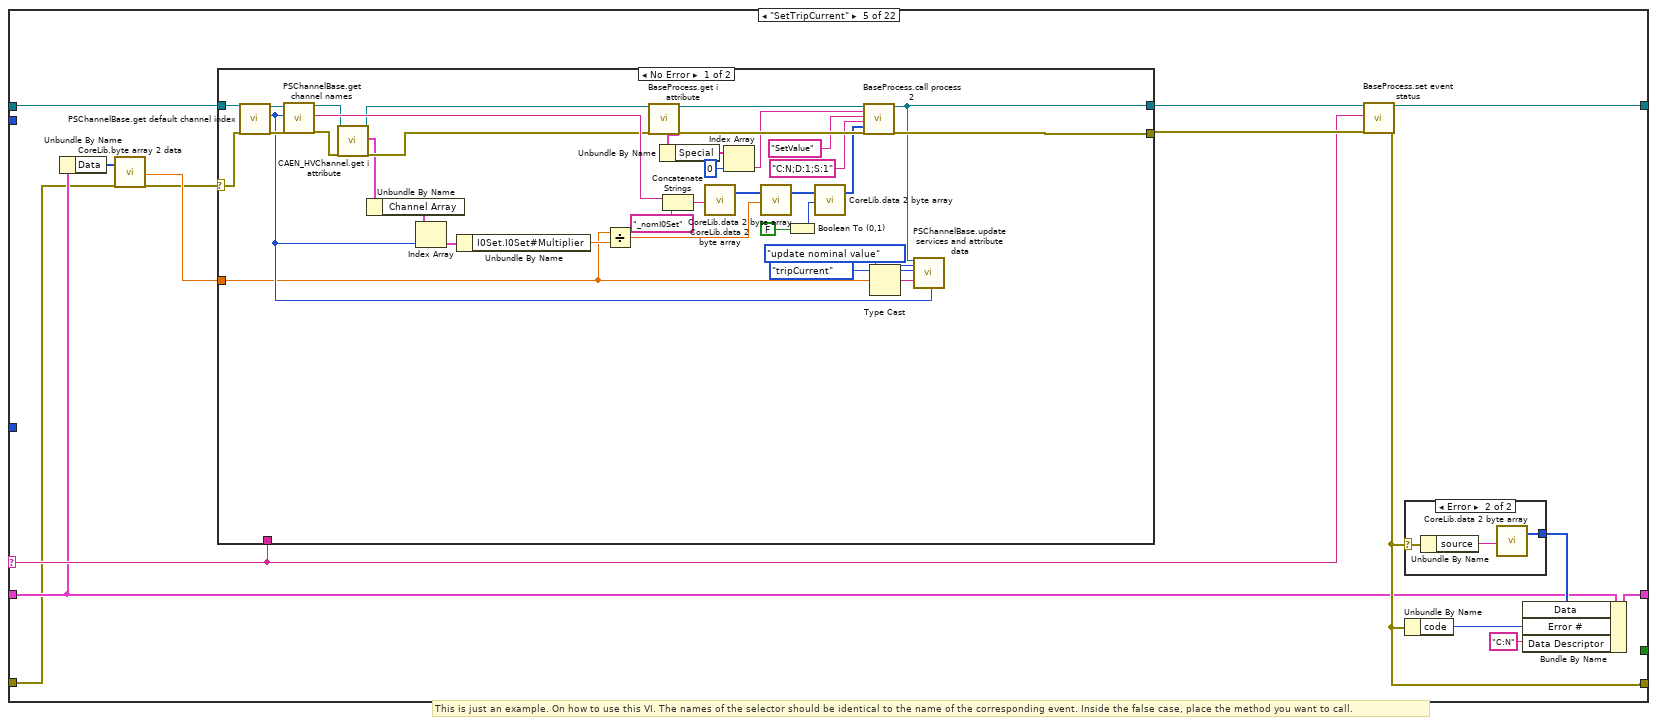
[diagram p11: hidden frame]
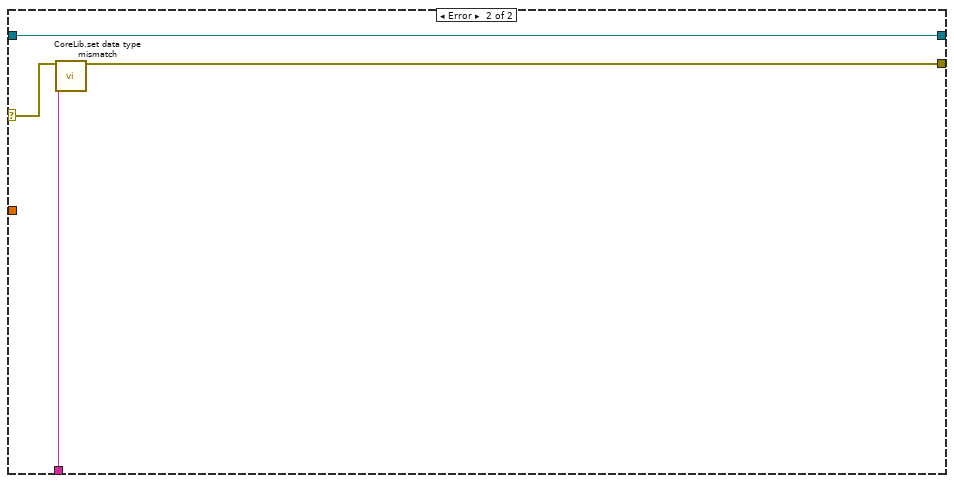
[diagram p13: hidden frame]
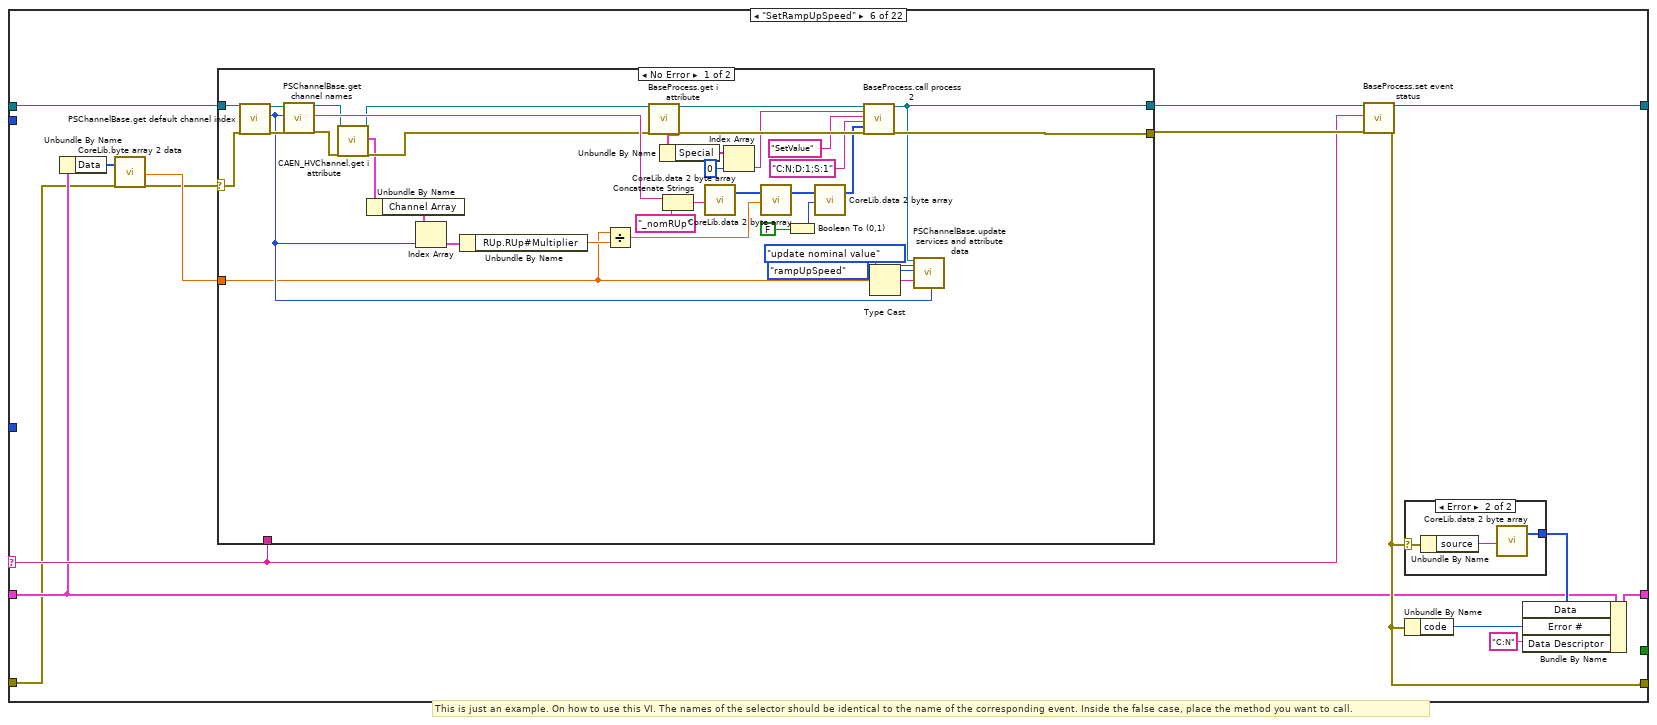
[diagram p14: hidden frame]
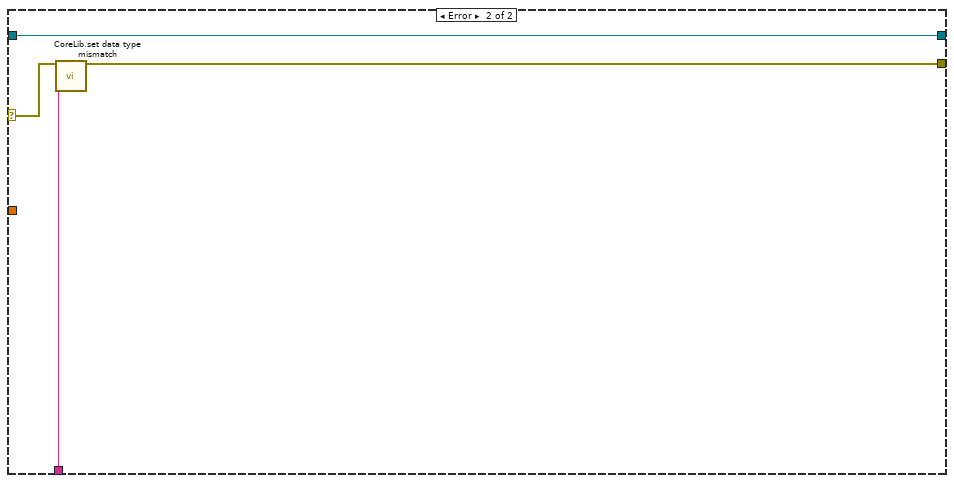
[diagram p16: hidden frame]
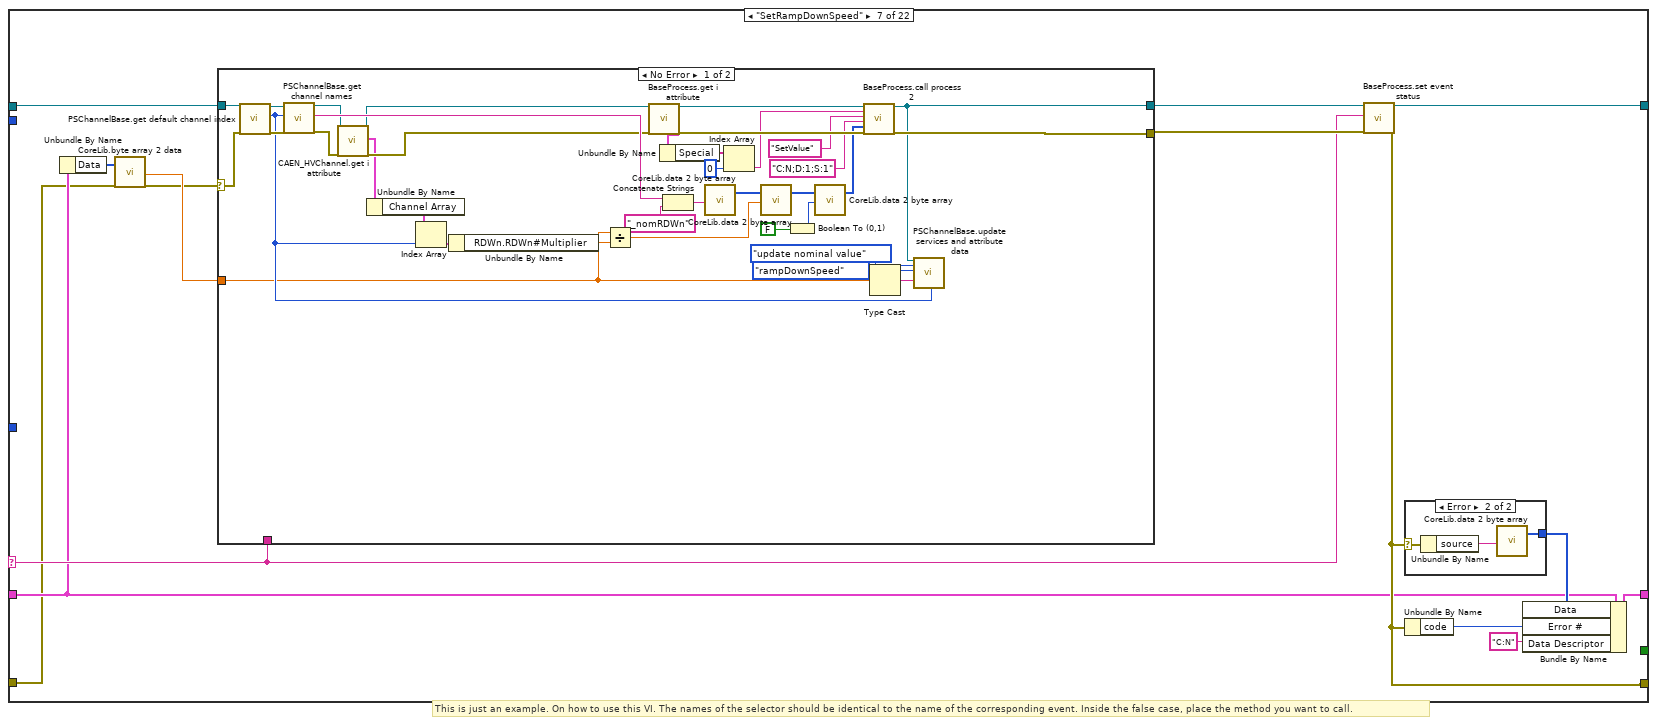
[diagram p17: hidden frame]
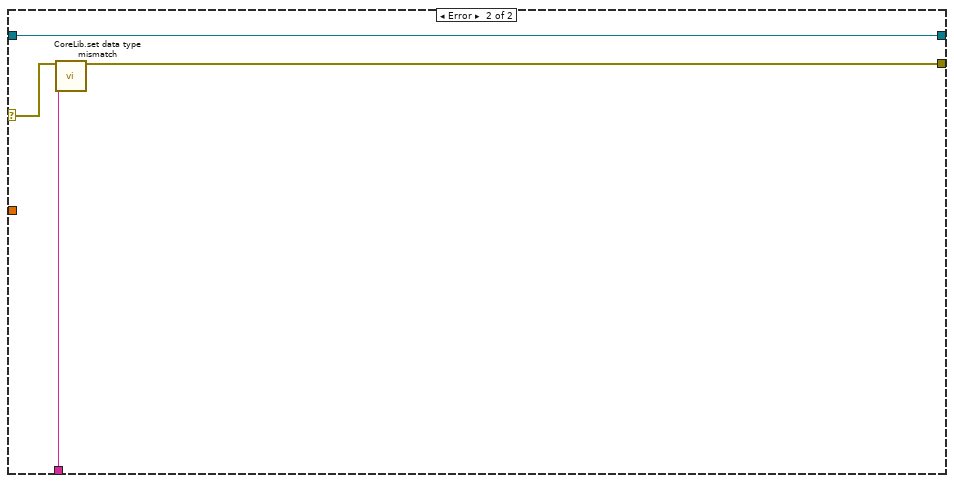
[diagram p19: hidden frame]
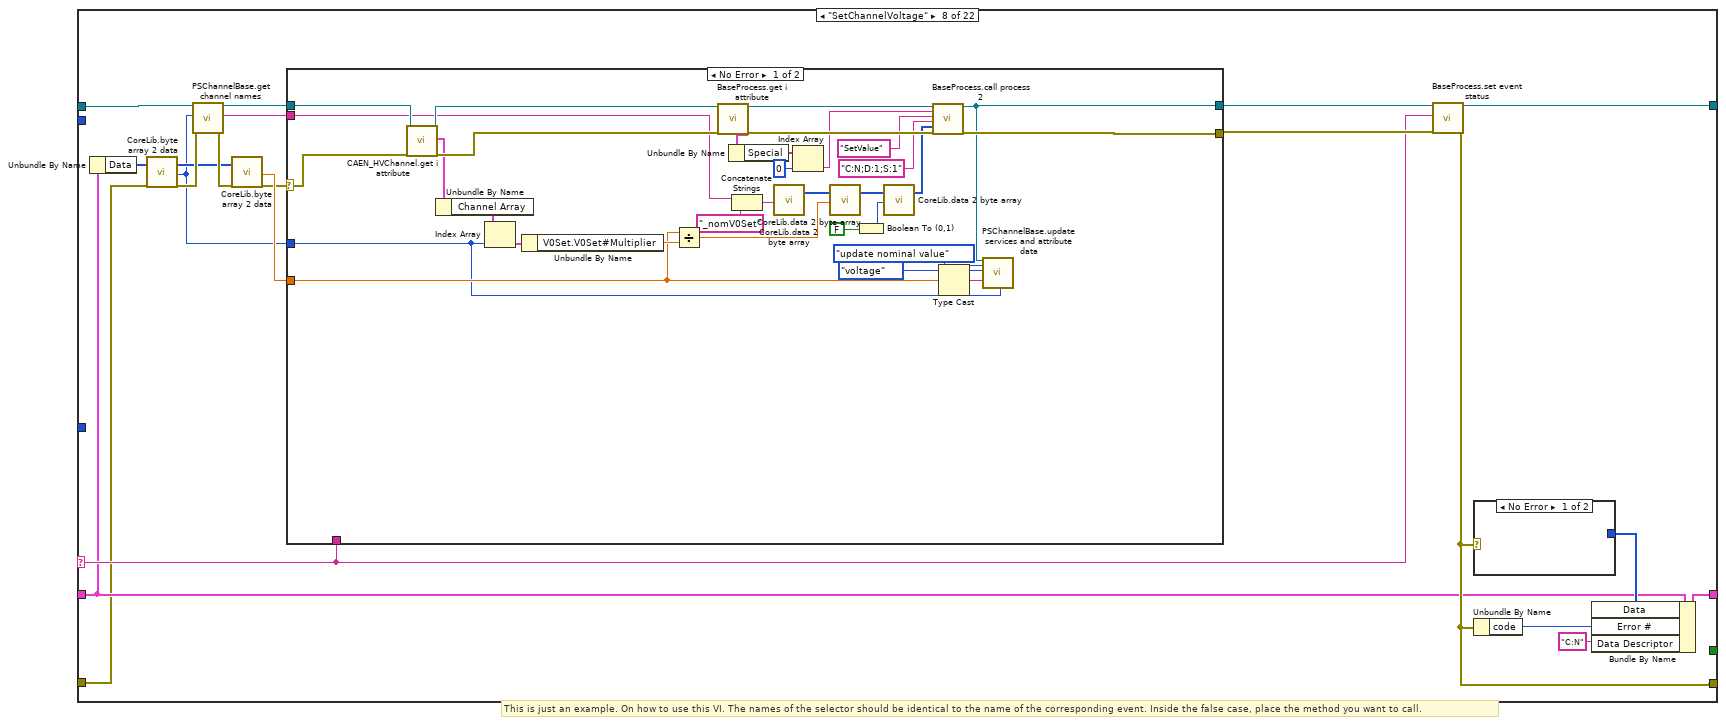
[diagram p20: hidden frame]
diagram:
  n1 = case shown="No Error" "error in (no error)" {
    selector: "error in (no error)" -> [w14 w2795]
    tunnel: "selector" -> [w19 _]
    tunnel: [w18 w2796] -> w8
    tunnel: "Data" -> [w17 _]
    tunnel: "call cluster" -> [w16 w2796]
    tunnel: "i ref in" -> [w15 w2797]
    tunnel: [w11 w2797] -> w4
    tunnel: [w12 w2795] -> w3
    tunnel: -1 ("ms timeout (10000)") -> [w10 _]
    frame No Error {
      n2 = case shown="\"SetVoltage\"" w19 {
        selector: w19 -> [w25 w39 w97 w150 w194 w252 w310 w374 w434 w493 w552 w611 w670 w729 w788 w845 w902 w956 w1016 w1076 w1129 w1161]
        tunnel: w17 -> [_ _ _ _ _ _ _ _ _ _ _ _ _ _ _ _ _ _ _ _ _ w1158]
        tunnel: w15 -> [w24 w32 w90 w146 w187 w245 w303 w363 w423 w482 w541 w600 w659 w718 w777 w834 w891 w945 w1005 w1065 w1138 w1149]
        tunnel: [w30 w38 w96 w149 w193 w251 w309 w373 w433 w492 w551 w610 w669 w728 w787 w844 w901 w955 w1015 w1075 w1128 w1160] -> w11
        tunnel: w16 -> [w26 w35 w93 w147 w190 w248 w306 w371 w431 w490 w549 w608 w667 w726 w785 w842 w899 w953 w1013 w1073 w1135 w1167]
        tunnel: [w27 w44 w102 w155 w199 w257 w315 w379 w439 w498 w557 w616 w675 w734 w793 w850 w907 w961 w1021 w1081 w1134 w1166] -> w18
        tunnel: w14 -> [w29 w31 w89 w145 w186 w244 w302 w367 w427 w486 w545 w604 w663 w722 w781 w838 w895 w949 w1009 w1069 w1137 w1151]
        tunnel: [w28 w40 w98 w151 w195 w253 w311 w375 w435 w494 w553 w612 w671 w730 w789 w846 w903 w957 w1017 w1077 w1130 w1162] -> w12
        tunnel: [TRUE _ _ _ _ _ _ _ _ _ _ _ _ _ _ _ _ _ _ _ _ _] -> w13
        tunnel: w10 -> [_ _ _ _ _ _ _ _ _ _ _ _ _ _ _ _ _ _ _ _ _ w1156]
        frame Default {
          # "In the default case, always call the ProcCase method of the parent class"
          n3 = call "PSChannelBase.ProcCases.vi"("i ref in"=w24, "selector"=w25, "call cluster"=w26, "error in (no error)"=w29) -> ("i ref out"=w30:refnum<vi>, "answer cluster"=w27:T2, "error out"=w28:errorcluster)  [unwired: 13 in]
        }
        frame "SetVoltage" {
          # "This is just an example. On how to use this VI. The names of the selector should be identical to the name of the corresponding event. Inside the false case, place the method you want to call."
          n4 = Unbundle By Name(w35) -> ("Data"=w36:T1)
          n5 = call-poly "CoreLib.byte array 2 data.vi"("byteArray"=w36, "error in (no error)"=w31) -> ("d64"=w34:dbl, "error out"=w33:errorcluster)  [unwired: 15 in, 1 out]
          n6 = case shown="No Error" w33 {
            selector: w33 -> [w61 w85]
            tunnel: [w65 w88] -> w42
            tunnel: w32 -> [w63 w88]
            tunnel: [w66 w87] -> w41
            tunnel: w39 -> [_ w86]
            tunnel: w34 -> [w50 _]
            frame No Error {
              n7 = call "PSChannelBase.get default channel index.vi"("i ref in"=w63, "error in (no error)"=w61) -> ("i ref out"=w64:refnum<vi>, "defaultChannelIndex"=w53:i32, "error out"=w62:errorcluster)  [unwired: 15 in]
              n8 = call "PSChannelBase.get channel names.vi"("i ref in"=w64, "channelIndex"=w53, "error in (no error)"=w62) -> ("i ref out"=w56:refnum<vi>, "physcialName"=w60:string, "error out"=w59:errorcluster)  [unwired: 13 in, 1 out]
              n9 = call "CAEN_HVChannel.get i attribute.vi"("i ref in"=w56, "error in (no error)"=w59) -> ("i ref out"=w55:refnum<vi>, "i attribute"=w57:T9, "error out"=w58:errorcluster)  [unwired: 15 in]
              n10 = Unbundle By Name(w57) -> ("Channel Array"=w54:T10)
              n11 = Index Array(array=w54, index=w53) -> (element=w52:T11)
              n12 = Unbundle By Name(w52) -> ("V0Set.V0Set#Multiplier"=w51:dbl)
              n13 = Divide(x=w50, y=w51) -> (x/y=w49:dbl)
              n14 = call "BaseProcess.get i attribute.vi"("i ref in"=w55, "error in (no error)"=w58) -> ("i ref out"=w77:refnum<vi>, "i attribute"=w80:T12, "error out"=w81:errorcluster)  [unwired: 15 in]
              n15 = Unbundle By Name(w80) -> ("Special"=w79:string[])
              n16 = Concatenate Strings(w60, "_nomV0Set" ("string")) -> (w68:string)
              n17 = call-poly "CoreLib.data 2 byte array.vi"("string"=w68) -> ("byteArray out"=w73:T1)  [unwired: 18 in]
              n18 = Index Array(array=w79, index=0) -> (element=w76:string)
              n19 = call-poly "CoreLib.data 2 byte array.vi"("byteArray"=w73, "f64"=w49) -> ("byteArray out"=w72:T1)  [unwired: 17 in]
              n20 = Boolean To (0,1)(Boolean=FALSE) -> (0, 1=w70:i16)
              n21 = call-poly "CoreLib.data 2 byte array.vi"("byteArray"=w72, "i16"=w70) -> ("byteArray out"=w69:T1)  [unwired: 17 in]
              n22 = call "BaseProcess.call process 2.vi"("i ref in"=w77, "Object"=w76, "Selector"="SetValue", "Data Descriptor"="C:N;D:1;S:1", "Data"=w69, "error in (no error)"=w81) -> ("i ref out"=w65:refnum<vi>, "error out"=w66:errorcluster)  [unwired: 12 in]
              n23 = Type Cast(x=w50) -> (*(type *) &x=w84:string)  [unwired: 1 in]
              n24 = call "PSChannelBase.update services and attribute data.vi"("i ref in"=w65, "direction"=PSChannelBase.directionType."update nominal value", "service"=PSChannelBase.serviceType."voltage", "value"=w84, "channelNumber"=w53) -> ()  [unwired: 12 in, 3 out]
            }
            frame Error {
              n25 = call "CoreLib.set data type mismatch.vi"("error in (no error)"=w85, "error source"=w86) -> ("error out"=w87:errorcluster)  [unwired: 17 in]
            }
          }
          n26 = call "BaseProcess.set event status.vi"("i ref in"=w42, "EventStatus"=w39, "error in (no error)"=w41) -> ("i ref out"=w38:refnum<vi>, "error out"=w40:errorcluster)  [unwired: 14 in, 1 out]
          n27 = case shown="Error" w40 {
            selector: w40 -> [_ w48]
            tunnel: [_ w47] -> w43
            frame No Error {
            }
            frame Error {
              n28 = Unbundle By Name(w48) -> ("source"=w46:string)
              n29 = call-poly "CoreLib.data 2 byte array.vi"("string"=w46) -> ("byteArray out"=w47:T1)  [unwired: 18 in]
            }
          }
          n30 = Unbundle By Name(w40) -> ("code"=w45:i32)
          n31 = Bundle By Name(cluster=w35, "Data"=w43, "Error #"=w45, "Data Descriptor"="C:N") -> (w44:T2)
        }
        frame "SetOnOff" {
          # "This is just an example. On how to use this VI. The names of the selector should be identical to the name of the corresponding event. Inside the false case, place the method you want to call."
          n32 = Unbundle By Name(w93) -> ("Data"=w94:T1)
          n33 = call-poly "CoreLib.byte array 2 data.vi"("byteArray"=w94, "error in (no error)"=w89) -> ("i16"=w92:i16, "error out"=w91:errorcluster)  [unwired: 15 in, 1 out]
          n34 = case shown="No Error" w91 {
            selector: w91 -> [w113 w137]
            tunnel: [w117 w140] -> w100
            tunnel: w90 -> [w115 w140]
            tunnel: [w118 w139] -> w99
            tunnel: w97 -> [_ w138]
            tunnel: w92 -> [w108 _]
            frame No Error {
              n35 = call "PSChannelBase.get default channel index.vi"("i ref in"=w115, "error in (no error)"=w113) -> ("i ref out"=w116:refnum<vi>, "defaultChannelIndex"=w111:i32, "error out"=w114:errorcluster)  [unwired: 15 in]
              n36 = call "PSChannelBase.get channel names.vi"("i ref in"=w116, "channelIndex"=w111, "error in (no error)"=w114) -> ("i ref out"=w110:refnum<vi>, "physcialName"=w112:string, "error out"=w109:errorcluster)  [unwired: 13 in, 1 out]
              n37 = call "BaseProcess.get i attribute.vi"("i ref in"=w110, "error in (no error)"=w109) -> ("i ref out"=w129:refnum<vi>, "i attribute"=w132:T12, "error out"=w133:errorcluster)  [unwired: 15 in]
              n38 = Unbundle By Name(w132) -> ("Special"=w131:string[])
              n39 = Concatenate Strings(w112, "_nomPw" ("string")) -> (w120:string)
              n40 = call-poly "CoreLib.data 2 byte array.vi"("string"=w120) -> ("byteArray out"=w125:T1)  [unwired: 18 in]
              n41 = Index Array(array=w131, index=0) -> (element=w128:string)
              n42 = Not Equal To 0?(x=w108) -> (x != 0?=w107:bool)
              n43 = call-poly "CoreLib.data 2 byte array.vi"("byteArray"=w125, "i16"=w108) -> ("byteArray out"=w124:T1)  [unwired: 17 in]
              n44 = Boolean To (0,1)(Boolean=FALSE) -> (0, 1=w122:i16)
              n45 = call-poly "CoreLib.data 2 byte array.vi"("byteArray"=w124, "i16"=w122) -> ("byteArray out"=w121:T1)  [unwired: 17 in]
              n46 = call "BaseProcess.call process 2.vi"("i ref in"=w129, "Object"=w128, "Selector"="SetValue", "Data Descriptor"="C:N;S:1;S:1", "Data"=w121, "error in (no error)"=w133) -> ("i ref out"=w117:refnum<vi>, "error out"=w118:errorcluster)  [unwired: 12 in]
              n47 = Type Cast(x=w107) -> (*(type *) &x=w136:string)  [unwired: 1 in]
              n48 = call "PSChannelBase.update services and attribute data.vi"("i ref in"=w117, "direction"=PSChannelBase.directionType."update nominal value", "service"=PSChannelBase.serviceType."onOff", "value"=w136, "channelNumber"=w111) -> ()  [unwired: 12 in, 3 out]
            }
            frame Error {
              n49 = call "CoreLib.set data type mismatch.vi"("error in (no error)"=w137, "error source"=w138) -> ("error out"=w139:errorcluster)  [unwired: 17 in]
            }
          }
          n50 = call "BaseProcess.set event status.vi"("i ref in"=w100, "EventStatus"=w97, "error in (no error)"=w99) -> ("i ref out"=w96:refnum<vi>, "error out"=w98:errorcluster)  [unwired: 14 in, 1 out]
          n51 = case shown="Error" w98 {
            selector: w98 -> [_ w106]
            tunnel: [_ w105] -> w101
            frame No Error {
            }
            frame Error {
              n52 = Unbundle By Name(w106) -> ("source"=w104:string)
              n53 = call-poly "CoreLib.data 2 byte array.vi"("string"=w104) -> ("byteArray out"=w105:T1)  [unwired: 18 in]
            }
          }
          n54 = Unbundle By Name(w98) -> ("code"=w103:i32)
          n55 = Bundle By Name(cluster=w93, "Data"=w101, "Error #"=w103, "Data Descriptor"="C:N") -> (w102:T2)
        }
        frame "EmergencyOff" {
          # "This is just an example. On how to use this VI. The names of the selector should be identical to the name of the corresponding event. Inside the false case, place the method you want to call."
          n56 = call "PSChannelBase.get nof channels.vi"("i ref in"=w146, "error in (no error)"=w145) -> ("i ref out"=w143:refnum<vi>, "NofChannels"=w144:i32, "error out"=w142:errorcluster)  [unwired: 15 in]
          n57 = for {
            N: w144 -> [_]
            tunnel: [w166] -> w141 mode=indexing
            tunnel: [w165] -> w153
            tunnel: w143 -> [w160]
            tunnel: w142 -> [w159]
            i -> [w161]
            w158 = FALSE
            n58 = call "PSChannelBase.get channel names.vi"("i ref in"=w160, "channelIndex"=w161, "error in (no error)"=w159) -> ("i ref out"=w163:refnum<vi>, "physcialName"=w164:string, "error out"=w162:errorcluster)  [unwired: 13 in, 1 out]
            n59 = call "BaseProcess.get i attribute.vi"("i ref in"=w163, "error in (no error)"=w162) -> ("i ref out"=w175:refnum<vi>, "i attribute"=w178:T12, "error out"=w179:errorcluster)  [unwired: 15 in]
            n60 = Unbundle By Name(w178) -> ("Special"=w177:string[])
            n61 = Concatenate Strings(w164, "_nomPw" ("string")) -> (w168:string)
            n62 = Boolean To (0,1)(Boolean=w158) -> (0, 1=w157:i16)
            n63 = call-poly "CoreLib.data 2 byte array.vi"("string"=w168) -> ("byteArray out"=w171:T1)  [unwired: 18 in]
            n64 = Index Array(array=w177, index=0) -> (element=w174:string)
            n65 = call-poly "CoreLib.data 2 byte array.vi"("byteArray"=w171, "i16"=w157) -> ("byteArray out"=w170:T1)  [unwired: 17 in]
            n66 = call-poly "CoreLib.data 2 byte array.vi"("byteArray"=w170, "i16"=w157) -> ("byteArray out"=w169:T1)  [unwired: 17 in]
            n67 = call "BaseProcess.call process 2.vi"("i ref in"=w175, "Object"=w174, "Selector"="SetValue", "Data Descriptor"="C:N;S:1;S:1", "Data"=w169, "error in (no error)"=w179) -> ("i ref out"=w165:refnum<vi>, "error out"=w166:errorcluster)  [unwired: 12 in]
            n68 = Type Cast(x=w158) -> (*(type *) &x=w182:string)  [unwired: 1 in]
            n69 = call "PSChannelBase.update services and attribute data.vi"("i ref in"=w165, "direction"=PSChannelBase.directionType."update nominal value", "service"=PSChannelBase.serviceType."onOff", "value"=w182, "channelNumber"=w161) -> ()  [unwired: 12 in, 3 out]
          }
          n70 = Merge Errors(w141) -> (w152:errorcluster)
          n71 = call "BaseProcess.set event status.vi"("i ref in"=w153, "EventStatus"=w150, "error in (no error)"=w152) -> ("i ref out"=w149:refnum<vi>, "error out"=w151:errorcluster)  [unwired: 14 in, 1 out]
          n72 = case shown="Error" w151 {
            selector: w151 -> [_ w185]
            tunnel: [_ w184] -> w154
            frame No Error {
            }
            frame Error {
              n73 = Unbundle By Name(w185) -> ("source"=w183:string)
              n74 = call-poly "CoreLib.data 2 byte array.vi"("string"=w183) -> ("byteArray out"=w184:T1)  [unwired: 18 in]
            }
          }
          n75 = Unbundle By Name(w151) -> ("code"=w156:i32)
          n76 = Bundle By Name(cluster=w147, "Data"=w154, "Error #"=w156, "Data Descriptor"="C:N") -> (w155:T2)
        }
        frame "SetTripCurrent" {
          # "This is just an example. On how to use this VI. The names of the selector should be identical to the name of the corresponding event. Inside the false case, place the method you want to call."
          n77 = Unbundle By Name(w190) -> ("Data"=w191:T1)
          n78 = call-poly "CoreLib.byte array 2 data.vi"("byteArray"=w191, "error in (no error)"=w186) -> ("d64"=w189:dbl, "error out"=w188:errorcluster)  [unwired: 15 in, 1 out]
          n79 = case shown="No Error" w188 {
            selector: w188 -> [w216 w240]
            tunnel: [w220 w243] -> w197
            tunnel: w187 -> [w218 w243]
            tunnel: [w221 w242] -> w196
            tunnel: w194 -> [_ w241]
            tunnel: w189 -> [w205 _]
            frame No Error {
              n80 = call "PSChannelBase.get default channel index.vi"("i ref in"=w218, "error in (no error)"=w216) -> ("i ref out"=w219:refnum<vi>, "defaultChannelIndex"=w208:i32, "error out"=w217:errorcluster)  [unwired: 15 in]
              n81 = call "PSChannelBase.get channel names.vi"("i ref in"=w219, "channelIndex"=w208, "error in (no error)"=w217) -> ("i ref out"=w211:refnum<vi>, "physcialName"=w215:string, "error out"=w214:errorcluster)  [unwired: 13 in, 1 out]
              n82 = call "CAEN_HVChannel.get i attribute.vi"("i ref in"=w211, "error in (no error)"=w214) -> ("i ref out"=w210:refnum<vi>, "i attribute"=w212:T9, "error out"=w213:errorcluster)  [unwired: 15 in]
              n83 = Unbundle By Name(w212) -> ("Channel Array"=w209:T10)
              n84 = Index Array(array=w209, index=w208) -> (element=w207:T11)
              n85 = Unbundle By Name(w207) -> ("I0Set.I0Set#Multiplier"=w206:dbl)
              n86 = Divide(x=w205, y=w206) -> (x/y=w204:dbl)
              n87 = call "BaseProcess.get i attribute.vi"("i ref in"=w210, "error in (no error)"=w213) -> ("i ref out"=w232:refnum<vi>, "i attribute"=w235:T12, "error out"=w236:errorcluster)  [unwired: 15 in]
              n88 = Unbundle By Name(w235) -> ("Special"=w234:string[])
              n89 = Concatenate Strings(w215, "_nomI0Set" ("string")) -> (w223:string)
              n90 = call-poly "CoreLib.data 2 byte array.vi"("string"=w223) -> ("byteArray out"=w228:T1)  [unwired: 18 in]
              n91 = Index Array(array=w234, index=0) -> (element=w231:string)
              n92 = call-poly "CoreLib.data 2 byte array.vi"("byteArray"=w228, "f64"=w204) -> ("byteArray out"=w227:T1)  [unwired: 17 in]
              n93 = Boolean To (0,1)(Boolean=FALSE) -> (0, 1=w225:i16)
              n94 = call-poly "CoreLib.data 2 byte array.vi"("byteArray"=w227, "i16"=w225) -> ("byteArray out"=w224:T1)  [unwired: 17 in]
              n95 = call "BaseProcess.call process 2.vi"("i ref in"=w232, "Object"=w231, "Selector"="SetValue", "Data Descriptor"="C:N;D:1;S:1", "Data"=w224, "error in (no error)"=w236) -> ("i ref out"=w220:refnum<vi>, "error out"=w221:errorcluster)  [unwired: 12 in]
              n96 = Type Cast(x=w205) -> (*(type *) &x=w239:string)  [unwired: 1 in]
              n97 = call "PSChannelBase.update services and attribute data.vi"("i ref in"=w220, "direction"=PSChannelBase.directionType."update nominal value", "service"=PSChannelBase.serviceType."tripCurrent", "value"=w239, "channelNumber"=w208) -> ()  [unwired: 12 in, 3 out]
            }
            frame Error {
              n98 = call "CoreLib.set data type mismatch.vi"("error in (no error)"=w240, "error source"=w241) -> ("error out"=w242:errorcluster)  [unwired: 17 in]
            }
          }
          n99 = call "BaseProcess.set event status.vi"("i ref in"=w197, "EventStatus"=w194, "error in (no error)"=w196) -> ("i ref out"=w193:refnum<vi>, "error out"=w195:errorcluster)  [unwired: 14 in, 1 out]
          n100 = case shown="Error" w195 {
            selector: w195 -> [_ w203]
            tunnel: [_ w202] -> w198
            frame No Error {
            }
            frame Error {
              n101 = Unbundle By Name(w203) -> ("source"=w201:string)
              n102 = call-poly "CoreLib.data 2 byte array.vi"("string"=w201) -> ("byteArray out"=w202:T1)  [unwired: 18 in]
            }
          }
          n103 = Unbundle By Name(w195) -> ("code"=w200:i32)
          n104 = Bundle By Name(cluster=w190, "Data"=w198, "Error #"=w200, "Data Descriptor"="C:N") -> (w199:T2)
        }
        frame "SetRampUpSpeed" {
          # "This is just an example. On how to use this VI. The names of the selector should be identical to the name of the corresponding event. Inside the false case, place the method you want to call."
          n105 = Unbundle By Name(w248) -> ("Data"=w249:T1)
          n106 = call-poly "CoreLib.byte array 2 data.vi"("byteArray"=w249, "error in (no error)"=w244) -> ("d64"=w247:dbl, "error out"=w246:errorcluster)  [unwired: 15 in, 1 out]
          n107 = case shown="No Error" w246 {
            selector: w246 -> [w274 w298]
            tunnel: [w278 w301] -> w255
            tunnel: w245 -> [w276 w301]
            tunnel: [w279 w300] -> w254
            tunnel: w252 -> [_ w299]
            tunnel: w247 -> [w263 _]
            frame No Error {
              n108 = call "PSChannelBase.get default channel index.vi"("i ref in"=w276, "error in (no error)"=w274) -> ("i ref out"=w277:refnum<vi>, "defaultChannelIndex"=w266:i32, "error out"=w275:errorcluster)  [unwired: 15 in]
              n109 = call "PSChannelBase.get channel names.vi"("i ref in"=w277, "channelIndex"=w266, "error in (no error)"=w275) -> ("i ref out"=w269:refnum<vi>, "physcialName"=w273:string, "error out"=w272:errorcluster)  [unwired: 13 in, 1 out]
              n110 = call "CAEN_HVChannel.get i attribute.vi"("i ref in"=w269, "error in (no error)"=w272) -> ("i ref out"=w268:refnum<vi>, "i attribute"=w270:T9, "error out"=w271:errorcluster)  [unwired: 15 in]
              n111 = Unbundle By Name(w270) -> ("Channel Array"=w267:T10)
              n112 = Index Array(array=w267, index=w266) -> (element=w265:T11)
              n113 = Unbundle By Name(w265) -> ("RUp.RUp#Multiplier"=w264:dbl)
              n114 = Divide(x=w263, y=w264) -> (x/y=w262:dbl)
              n115 = call "BaseProcess.get i attribute.vi"("i ref in"=w268, "error in (no error)"=w271) -> ("i ref out"=w290:refnum<vi>, "i attribute"=w293:T12, "error out"=w294:errorcluster)  [unwired: 15 in]
              n116 = Unbundle By Name(w293) -> ("Special"=w292:string[])
              n117 = Concatenate Strings(w273, "_nomRUp" ("string")) -> (w281:string)
              n118 = call-poly "CoreLib.data 2 byte array.vi"("string"=w281) -> ("byteArray out"=w286:T1)  [unwired: 18 in]
              n119 = Index Array(array=w292, index=0) -> (element=w289:string)
              n120 = call-poly "CoreLib.data 2 byte array.vi"("byteArray"=w286, "f64"=w262) -> ("byteArray out"=w285:T1)  [unwired: 17 in]
              n121 = Boolean To (0,1)(Boolean=FALSE) -> (0, 1=w283:i16)
              n122 = call-poly "CoreLib.data 2 byte array.vi"("byteArray"=w285, "i16"=w283) -> ("byteArray out"=w282:T1)  [unwired: 17 in]
              n123 = call "BaseProcess.call process 2.vi"("i ref in"=w290, "Object"=w289, "Selector"="SetValue", "Data Descriptor"="C:N;D:1;S:1", "Data"=w282, "error in (no error)"=w294) -> ("i ref out"=w278:refnum<vi>, "error out"=w279:errorcluster)  [unwired: 12 in]
              n124 = Type Cast(x=w263) -> (*(type *) &x=w297:string)  [unwired: 1 in]
              n125 = call "PSChannelBase.update services and attribute data.vi"("i ref in"=w278, "direction"=PSChannelBase.directionType."update nominal value", "service"=PSChannelBase.serviceType."rampUpSpeed", "value"=w297, "channelNumber"=w266) -> ()  [unwired: 12 in, 3 out]
            }
            frame Error {
              n126 = call "CoreLib.set data type mismatch.vi"("error in (no error)"=w298, "error source"=w299) -> ("error out"=w300:errorcluster)  [unwired: 17 in]
            }
          }
          n127 = call "BaseProcess.set event status.vi"("i ref in"=w255, "EventStatus"=w252, "error in (no error)"=w254) -> ("i ref out"=w251:refnum<vi>, "error out"=w253:errorcluster)  [unwired: 14 in, 1 out]
          n128 = case shown="Error" w253 {
            selector: w253 -> [_ w261]
            tunnel: [_ w260] -> w256
            frame No Error {
            }
            frame Error {
              n129 = Unbundle By Name(w261) -> ("source"=w259:string)
              n130 = call-poly "CoreLib.data 2 byte array.vi"("string"=w259) -> ("byteArray out"=w260:T1)  [unwired: 18 in]
            }
          }
          n131 = Unbundle By Name(w253) -> ("code"=w258:i32)
          n132 = Bundle By Name(cluster=w248, "Data"=w256, "Error #"=w258, "Data Descriptor"="C:N") -> (w257:T2)
        }
        frame "SetRampDownSpeed" {
          # "This is just an example. On how to use this VI. The names of the selector should be identical to the name of the corresponding event. Inside the false case, place the method you want to call."
          n133 = Unbundle By Name(w306) -> ("Data"=w307:T1)
          n134 = call-poly "CoreLib.byte array 2 data.vi"("byteArray"=w307, "error in (no error)"=w302) -> ("d64"=w305:dbl, "error out"=w304:errorcluster)  [unwired: 15 in, 1 out]
          n135 = case shown="No Error" w304 {
            selector: w304 -> [w332 w356]
            tunnel: [w336 w359] -> w313
            tunnel: w303 -> [w334 w359]
            tunnel: [w337 w358] -> w312
            tunnel: w310 -> [_ w357]
            tunnel: w305 -> [w321 _]
            frame No Error {
              n136 = call "PSChannelBase.get default channel index.vi"("i ref in"=w334, "error in (no error)"=w332) -> ("i ref out"=w335:refnum<vi>, "defaultChannelIndex"=w324:i32, "error out"=w333:errorcluster)  [unwired: 15 in]
              n137 = call "PSChannelBase.get channel names.vi"("i ref in"=w335, "channelIndex"=w324, "error in (no error)"=w333) -> ("i ref out"=w327:refnum<vi>, "physcialName"=w331:string, "error out"=w330:errorcluster)  [unwired: 13 in, 1 out]
              n138 = call "CAEN_HVChannel.get i attribute.vi"("i ref in"=w327, "error in (no error)"=w330) -> ("i ref out"=w326:refnum<vi>, "i attribute"=w328:T9, "error out"=w329:errorcluster)  [unwired: 15 in]
              n139 = Unbundle By Name(w328) -> ("Channel Array"=w325:T10)
              n140 = Index Array(array=w325, index=w324) -> (element=w323:T11)
              n141 = Unbundle By Name(w323) -> ("RDWn.RDWn#Multiplier"=w322:dbl)
              n142 = Divide(x=w321, y=w322) -> (x/y=w320:dbl)
              n143 = call "BaseProcess.get i attribute.vi"("i ref in"=w326, "error in (no error)"=w329) -> ("i ref out"=w348:refnum<vi>, "i attribute"=w351:T12, "error out"=w352:errorcluster)  [unwired: 15 in]
              n144 = Unbundle By Name(w351) -> ("Special"=w350:string[])
              n145 = Concatenate Strings(w331, "_nomRDWn" ("string")) -> (w339:string)
              n146 = call-poly "CoreLib.data 2 byte array.vi"("string"=w339) -> ("byteArray out"=w344:T1)  [unwired: 18 in]
              n147 = Index Array(array=w350, index=0) -> (element=w347:string)
              n148 = call-poly "CoreLib.data 2 byte array.vi"("byteArray"=w344, "f64"=w320) -> ("byteArray out"=w343:T1)  [unwired: 17 in]
              n149 = Boolean To (0,1)(Boolean=FALSE) -> (0, 1=w341:i16)
              n150 = call-poly "CoreLib.data 2 byte array.vi"("byteArray"=w343, "i16"=w341) -> ("byteArray out"=w340:T1)  [unwired: 17 in]
              n151 = call "BaseProcess.call process 2.vi"("i ref in"=w348, "Object"=w347, "Selector"="SetValue", "Data Descriptor"="C:N;D:1;S:1", "Data"=w340, "error in (no error)"=w352) -> ("i ref out"=w336:refnum<vi>, "error out"=w337:errorcluster)  [unwired: 12 in]
              n152 = Type Cast(x=w321) -> (*(type *) &x=w355:string)  [unwired: 1 in]
              n153 = call "PSChannelBase.update services and attribute data.vi"("i ref in"=w336, "direction"=PSChannelBase.directionType."update nominal value", "service"=PSChannelBase.serviceType."rampDownSpeed", "value"=w355, "channelNumber"=w324) -> ()  [unwired: 12 in, 3 out]
            }
            frame Error {
              n154 = call "CoreLib.set data type mismatch.vi"("error in (no error)"=w356, "error source"=w357) -> ("error out"=w358:errorcluster)  [unwired: 17 in]
            }
          }
          n155 = call "BaseProcess.set event status.vi"("i ref in"=w313, "EventStatus"=w310, "error in (no error)"=w312) -> ("i ref out"=w309:refnum<vi>, "error out"=w311:errorcluster)  [unwired: 14 in, 1 out]
          n156 = case shown="Error" w311 {
            selector: w311 -> [_ w319]
            tunnel: [_ w318] -> w314
            frame No Error {
            }
            frame Error {
              n157 = Unbundle By Name(w319) -> ("source"=w317:string)
              n158 = call-poly "CoreLib.data 2 byte array.vi"("string"=w317) -> ("byteArray out"=w318:T1)  [unwired: 18 in]
            }
          }
          n159 = Unbundle By Name(w311) -> ("code"=w316:i32)
          n160 = Bundle By Name(cluster=w306, "Data"=w314, "Error #"=w316, "Data Descriptor"="C:N") -> (w315:T2)
        }
        frame "SetChannelVoltage" {
          # "This is just an example. On how to use this VI. The names of the selector should be identical to the name of the corresponding event. Inside the false case, place the method you want to call."
          n161 = Unbundle By Name(w371) -> ("Data"=w366:T1)
          n162 = call-poly "CoreLib.byte array 2 data.vi"("byteArray"=w366, "error in (no error)"=w367) -> ("byteArray out"=w364:T1, "i32"=w360:i32, "error out"=w368:errorcluster)  [unwired: 15 in]
          n163 = call "PSChannelBase.get channel names.vi"("i ref in"=w363, "channelIndex"=w360, "error in (no error)"=w368) -> ("i ref out"=w362:refnum<vi>, "physcialName"=w361:string, "error out"=w365:errorcluster)  [unwired: 13 in, 1 out]
          n164 = call-poly "CoreLib.byte array 2 data.vi"("byteArray"=w364, "error in (no error)"=w365) -> ("d64"=w370:dbl, "error out"=w369:errorcluster)  [unwired: 15 in, 1 out]
          n165 = case shown="No Error" w369 {
            selector: w369 -> [w385 w416]
            tunnel: [w396 w419] -> w377
            tunnel: w362 -> [w387 w419]
            tunnel: [w397 w418] -> w376
            tunnel: w374 -> [_ w417]
            tunnel: w370 -> [w390 _]
            tunnel: w361 -> [w386 _]
            tunnel: w360 -> [w384 _]
            frame No Error {
              n166 = call "CAEN_HVChannel.get i attribute.vi"("i ref in"=w387, "error in (no error)"=w385) -> ("i ref out"=w388:refnum<vi>, "i attribute"=w394:T9, "error out"=w395:errorcluster)  [unwired: 15 in]
              n167 = Unbundle By Name(w394) -> ("Channel Array"=w393:T10)
              n168 = Index Array(array=w393, index=w384) -> (element=w392:T11)
              n169 = Unbundle By Name(w392) -> ("V0Set.V0Set#Multiplier"=w391:dbl)
              n170 = Divide(x=w390, y=w391) -> (x/y=w389:dbl)
              n171 = call "BaseProcess.get i attribute.vi"("i ref in"=w388, "error in (no error)"=w395) -> ("i ref out"=w408:refnum<vi>, "i attribute"=w411:T12, "error out"=w412:errorcluster)  [unwired: 15 in]
              n172 = Unbundle By Name(w411) -> ("Special"=w410:string[])
              n173 = Concatenate Strings(w386, "_nomV0Set" ("string")) -> (w399:string)
              n174 = call-poly "CoreLib.data 2 byte array.vi"("string"=w399) -> ("byteArray out"=w404:T1)  [unwired: 18 in]
              n175 = Index Array(array=w410, index=0) -> (element=w407:string)
              n176 = call-poly "CoreLib.data 2 byte array.vi"("byteArray"=w404, "f64"=w389) -> ("byteArray out"=w403:T1)  [unwired: 17 in]
              n177 = Boolean To (0,1)(Boolean=FALSE) -> (0, 1=w401:i16)
              n178 = call-poly "CoreLib.data 2 byte array.vi"("byteArray"=w403, "i16"=w401) -> ("byteArray out"=w400:T1)  [unwired: 17 in]
              n179 = call "BaseProcess.call process 2.vi"("i ref in"=w408, "Object"=w407, "Selector"="SetValue", "Data Descriptor"="C:N;D:1;S:1", "Data"=w400, "error in (no error)"=w412) -> ("i ref out"=w396:refnum<vi>, "error out"=w397:errorcluster)  [unwired: 12 in]
              n180 = Type Cast(x=w390) -> (*(type *) &x=w415:string)  [unwired: 1 in]
              n181 = call "PSChannelBase.update services and attribute data.vi"("i ref in"=w396, "direction"=PSChannelBase.directionType."update nominal value", "service"=PSChannelBase.serviceType."voltage", "value"=w415, "channelNumber"=w384) -> ()  [unwired: 12 in, 3 out]
            }
            frame Error {
              n182 = call "CoreLib.set data type mismatch.vi"("error in (no error)"=w416, "error source"=w417) -> ("error out"=w418:errorcluster)  [unwired: 17 in]
            }
          }
          n183 = call "BaseProcess.set event status.vi"("i ref in"=w377, "EventStatus"=w374, "error in (no error)"=w376) -> ("i ref out"=w373:refnum<vi>, "error out"=w375:errorcluster)  [unwired: 14 in, 1 out]
          n184 = case shown="No Error" w375 {
            selector: w375 -> [_ w383]
            tunnel: [_ w382] -> w378
            frame No Error {
            }
            frame Error {
              n185 = Unbundle By Name(w383) -> ("source"=w381:string)
              n186 = call-poly "CoreLib.data 2 byte array.vi"("string"=w381) -> ("byteArray out"=w382:T1)  [unwired: 18 in]
            }
          }
          n187 = Unbundle By Name(w375) -> ("code"=w380:i32)
          n188 = Bundle By Name(cluster=w371, "Data"=w378, "Error #"=w380, "Data Descriptor"="C:N") -> (w379:T2)
        }
        frame "SetChannelV1Set" {
          # "This is just an example. On how to use this VI. The names of the selector should be identical to the name of the corresponding event. Inside the false case, place the method you want to call."
          n189 = Unbundle By Name(w431) -> ("Data"=w426:T1)
          n190 = call-poly "CoreLib.byte array 2 data.vi"("byteArray"=w426, "error in (no error)"=w427) -> ("byteArray out"=w424:T1, "i32"=w420:i32, "error out"=w428:errorcluster)  [unwired: 15 in]
          n191 = call "PSChannelBase.get channel names.vi"("i ref in"=w423, "channelIndex"=w420, "error in (no error)"=w428) -> ("i ref out"=w422:refnum<vi>, "physcialName"=w421:string, "error out"=w425:errorcluster)  [unwired: 13 in, 1 out]
          n192 = call-poly "CoreLib.byte array 2 data.vi"("byteArray"=w424, "error in (no error)"=w425) -> ("d64"=w430:dbl, "error out"=w429:errorcluster)  [unwired: 15 in, 1 out]
          n193 = case shown="No Error" w429 {
            selector: w429 -> [w448 w475]
            tunnel: [w458 w478] -> w437
            tunnel: w422 -> [w450 w478]
            tunnel: [w459 w477] -> w436
            tunnel: w434 -> [_ w476]
            tunnel: w430 -> [w444 _]
            tunnel: w421 -> [w449 _]
            tunnel: w420 -> [w447 _]
            frame No Error {
              n194 = call "CAEN_HVChannel.get i attribute.vi"("i ref in"=w450, "error in (no error)"=w448) -> ("i ref out"=w451:refnum<vi>, "i attribute"=w456:T9, "error out"=w457:errorcluster)  [unwired: 15 in]
              n195 = Unbundle By Name(w456) -> ("Channel Array"=w455:T10)
              n196 = Index Array(array=w455, index=w447) -> (element=w454:T11)
              n197 = Unbundle By Name(w454) -> ("V1Set.V1Set#Multiplier"=w453:dbl, "DIM Service IDs.nomV1Set"=w446:i32)
              n198 = Divide(x=w444, y=w453) -> (x/y=w452:dbl)
              n199 = call "BaseProcess.get i attribute.vi"("i ref in"=w451, "error in (no error)"=w457) -> ("i ref out"=w470:refnum<vi>, "i attribute"=w473:T12, "error out"=w474:errorcluster)  [unwired: 15 in]
              n200 = Unbundle By Name(w473) -> ("Special"=w472:string[])
              n201 = Concatenate Strings(w449, "_nomV1Set" ("string")) -> (w461:string)
              n202 = call-poly "CoreLib.data 2 byte array.vi"("string"=w461) -> ("byteArray out"=w466:T1)  [unwired: 18 in]
              n203 = Index Array(array=w472, index=0) -> (element=w469:string)
              n204 = call-poly "CoreLib.data 2 byte array.vi"("byteArray"=w466, "f64"=w452) -> ("byteArray out"=w465:T1)  [unwired: 17 in]
              n205 = Boolean To (0,1)(Boolean=FALSE) -> (0, 1=w463:i16)
              n206 = Type Cast(x=w444) -> (*(type *) &x=w445:string)  [unwired: 1 in]
              n207 = call-poly "CoreLib.data 2 byte array.vi"("byteArray"=w465, "i16"=w463) -> ("byteArray out"=w462:T1)  [unwired: 17 in]
              n208 = call "LVDimInterface.dis_update_service.vi"("my_serviceID"=w446, "data"=w445) -> ()  [unwired: 15 in, 3 out]
              n209 = call "BaseProcess.call process 2.vi"("i ref in"=w470, "Object"=w469, "Selector"="SetValue", "Data Descriptor"="C:N;D:1;S:1", "Data"=w462, "error in (no error)"=w474) -> ("i ref out"=w458:refnum<vi>, "error out"=w459:errorcluster)  [unwired: 12 in]
            }
            frame Error {
              n210 = call "CoreLib.set data type mismatch.vi"("error in (no error)"=w475, "error source"=w476) -> ("error out"=w477:errorcluster)  [unwired: 17 in]
            }
          }
          n211 = call "BaseProcess.set event status.vi"("i ref in"=w437, "EventStatus"=w434, "error in (no error)"=w436) -> ("i ref out"=w433:refnum<vi>, "error out"=w435:errorcluster)  [unwired: 14 in, 1 out]
          n212 = case shown="Error" w435 {
            selector: w435 -> [_ w443]
            tunnel: [_ w442] -> w438
            frame No Error {
            }
            frame Error {
              n213 = Unbundle By Name(w443) -> ("source"=w441:string)
              n214 = call-poly "CoreLib.data 2 byte array.vi"("string"=w441) -> ("byteArray out"=w442:T1)  [unwired: 18 in]
            }
          }
          n215 = Unbundle By Name(w435) -> ("code"=w440:i32)
          n216 = Bundle By Name(cluster=w431, "Data"=w438, "Error #"=w440, "Data Descriptor"="C:N") -> (w439:T2)
        }
        frame "SetChannelI1Set" {
          # "This is just an example. On how to use this VI. The names of the selector should be identical to the name of the corresponding event. Inside the false case, place the method you want to call."
          n217 = Unbundle By Name(w490) -> ("Data"=w485:T1)
          n218 = call-poly "CoreLib.byte array 2 data.vi"("byteArray"=w485, "error in (no error)"=w486) -> ("byteArray out"=w483:T1, "i32"=w479:i32, "error out"=w487:errorcluster)  [unwired: 15 in]
          n219 = call "PSChannelBase.get channel names.vi"("i ref in"=w482, "channelIndex"=w479, "error in (no error)"=w487) -> ("i ref out"=w481:refnum<vi>, "physcialName"=w480:string, "error out"=w484:errorcluster)  [unwired: 13 in, 1 out]
          n220 = call-poly "CoreLib.byte array 2 data.vi"("byteArray"=w483, "error in (no error)"=w484) -> ("d64"=w489:dbl, "error out"=w488:errorcluster)  [unwired: 15 in, 1 out]
          n221 = case shown="No Error" w488 {
            selector: w488 -> [w507 w534]
            tunnel: [w517 w537] -> w496
            tunnel: w481 -> [w509 w537]
            tunnel: [w518 w536] -> w495
            tunnel: w493 -> [_ w535]
            tunnel: w489 -> [w503 _]
            tunnel: w480 -> [w508 _]
            tunnel: w479 -> [w506 _]
            frame No Error {
              n222 = call "CAEN_HVChannel.get i attribute.vi"("i ref in"=w509, "error in (no error)"=w507) -> ("i ref out"=w510:refnum<vi>, "i attribute"=w515:T9, "error out"=w516:errorcluster)  [unwired: 15 in]
              n223 = Unbundle By Name(w515) -> ("Channel Array"=w514:T10)
              n224 = Index Array(array=w514, index=w506) -> (element=w513:T11)
              n225 = Unbundle By Name(w513) -> ("I1Set.I1Set#Multiplier"=w512:dbl, "DIM Service IDs.nomI1Set"=w505:i32)
              n226 = Divide(x=w503, y=w512) -> (x/y=w511:dbl)
              n227 = call "BaseProcess.get i attribute.vi"("i ref in"=w510, "error in (no error)"=w516) -> ("i ref out"=w529:refnum<vi>, "i attribute"=w532:T12, "error out"=w533:errorcluster)  [unwired: 15 in]
              n228 = Unbundle By Name(w532) -> ("Special"=w531:string[])
              n229 = Concatenate Strings(w508, "_nomI1Set" ("string")) -> (w520:string)
              n230 = call-poly "CoreLib.data 2 byte array.vi"("string"=w520) -> ("byteArray out"=w525:T1)  [unwired: 18 in]
              n231 = Index Array(array=w531, index=0) -> (element=w528:string)
              n232 = call-poly "CoreLib.data 2 byte array.vi"("byteArray"=w525, "f64"=w511) -> ("byteArray out"=w524:T1)  [unwired: 17 in]
              n233 = Boolean To (0,1)(Boolean=FALSE) -> (0, 1=w522:i16)
              n234 = Type Cast(x=w503) -> (*(type *) &x=w504:string)  [unwired: 1 in]
              n235 = call-poly "CoreLib.data 2 byte array.vi"("byteArray"=w524, "i16"=w522) -> ("byteArray out"=w521:T1)  [unwired: 17 in]
              n236 = call "LVDimInterface.dis_update_service.vi"("my_serviceID"=w505, "data"=w504) -> ()  [unwired: 15 in, 3 out]
              n237 = call "BaseProcess.call process 2.vi"("i ref in"=w529, "Object"=w528, "Selector"="SetValue", "Data Descriptor"="C:N;D:1;S:1", "Data"=w521, "error in (no error)"=w533) -> ("i ref out"=w517:refnum<vi>, "error out"=w518:errorcluster)  [unwired: 12 in]
            }
            frame Error {
              n238 = call "CoreLib.set data type mismatch.vi"("error in (no error)"=w534, "error source"=w535) -> ("error out"=w536:errorcluster)  [unwired: 17 in]
            }
          }
          n239 = call "BaseProcess.set event status.vi"("i ref in"=w496, "EventStatus"=w493, "error in (no error)"=w495) -> ("i ref out"=w492:refnum<vi>, "error out"=w494:errorcluster)  [unwired: 14 in, 1 out]
          n240 = case shown="Error" w494 {
            selector: w494 -> [_ w502]
            tunnel: [_ w501] -> w497
            frame No Error {
            }
            frame Error {
              n241 = Unbundle By Name(w502) -> ("source"=w500:string)
              n242 = call-poly "CoreLib.data 2 byte array.vi"("string"=w500) -> ("byteArray out"=w501:T1)  [unwired: 18 in]
            }
          }
          n243 = Unbundle By Name(w494) -> ("code"=w499:i32)
          n244 = Bundle By Name(cluster=w490, "Data"=w497, "Error #"=w499, "Data Descriptor"="C:N") -> (w498:T2)
        }
        frame "SetChannelTripTime" {
          # "This is just an example. On how to use this VI. The names of the selector should be identical to the name of the corresponding event. Inside the false case, place the method you want to call."
          n245 = Unbundle By Name(w549) -> ("Data"=w544:T1)
          n246 = call-poly "CoreLib.byte array 2 data.vi"("byteArray"=w544, "error in (no error)"=w545) -> ("byteArray out"=w542:T1, "i32"=w538:i32, "error out"=w546:errorcluster)  [unwired: 15 in]
          n247 = call "PSChannelBase.get channel names.vi"("i ref in"=w541, "channelIndex"=w538, "error in (no error)"=w546) -> ("i ref out"=w540:refnum<vi>, "physcialName"=w539:string, "error out"=w543:errorcluster)  [unwired: 13 in, 1 out]
          n248 = call-poly "CoreLib.byte array 2 data.vi"("byteArray"=w542, "error in (no error)"=w543) -> ("d64"=w548:dbl, "error out"=w547:errorcluster)  [unwired: 15 in, 1 out]
          n249 = case shown="No Error" w547 {
            selector: w547 -> [w566 w593]
            tunnel: [w576 w596] -> w555
            tunnel: w540 -> [w568 w596]
            tunnel: [w577 w595] -> w554
            tunnel: w552 -> [_ w594]
            tunnel: w548 -> [w562 _]
            tunnel: w539 -> [w567 _]
            tunnel: w538 -> [w565 _]
            frame No Error {
              n250 = call "CAEN_HVChannel.get i attribute.vi"("i ref in"=w568, "error in (no error)"=w566) -> ("i ref out"=w569:refnum<vi>, "i attribute"=w574:T9, "error out"=w575:errorcluster)  [unwired: 15 in]
              n251 = Unbundle By Name(w574) -> ("Channel Array"=w573:T10)
              n252 = Index Array(array=w573, index=w565) -> (element=w572:T11)
              n253 = Unbundle By Name(w572) -> ("Trip.Trip#Multiplier"=w571:dbl, "DIM Service IDs.nomTrip"=w564:i32)
              n254 = Divide(x=w562, y=w571) -> (x/y=w570:dbl)
              n255 = call "BaseProcess.get i attribute.vi"("i ref in"=w569, "error in (no error)"=w575) -> ("i ref out"=w588:refnum<vi>, "i attribute"=w591:T12, "error out"=w592:errorcluster)  [unwired: 15 in]
              n256 = Unbundle By Name(w591) -> ("Special"=w590:string[])
              n257 = Concatenate Strings(w567, "_nomTrip" ("string")) -> (w579:string)
              n258 = call-poly "CoreLib.data 2 byte array.vi"("string"=w579) -> ("byteArray out"=w584:T1)  [unwired: 18 in]
              n259 = Index Array(array=w590, index=0) -> (element=w587:string)
              n260 = call-poly "CoreLib.data 2 byte array.vi"("byteArray"=w584, "f64"=w570) -> ("byteArray out"=w583:T1)  [unwired: 17 in]
              n261 = Boolean To (0,1)(Boolean=FALSE) -> (0, 1=w581:i16)
              n262 = Type Cast(x=w562) -> (*(type *) &x=w563:string)  [unwired: 1 in]
              n263 = call-poly "CoreLib.data 2 byte array.vi"("byteArray"=w583, "i16"=w581) -> ("byteArray out"=w580:T1)  [unwired: 17 in]
              n264 = call "LVDimInterface.dis_update_service.vi"("my_serviceID"=w564, "data"=w563) -> ()  [unwired: 15 in, 3 out]
              n265 = call "BaseProcess.call process 2.vi"("i ref in"=w588, "Object"=w587, "Selector"="SetValue", "Data Descriptor"="C:N;D:1;S:1", "Data"=w580, "error in (no error)"=w592) -> ("i ref out"=w576:refnum<vi>, "error out"=w577:errorcluster)  [unwired: 12 in]
            }
            frame Error {
              n266 = call "CoreLib.set data type mismatch.vi"("error in (no error)"=w593, "error source"=w594) -> ("error out"=w595:errorcluster)  [unwired: 17 in]
            }
          }
          n267 = call "BaseProcess.set event status.vi"("i ref in"=w555, "EventStatus"=w552, "error in (no error)"=w554) -> ("i ref out"=w551:refnum<vi>, "error out"=w553:errorcluster)  [unwired: 14 in, 1 out]
          n268 = case shown="Error" w553 {
            selector: w553 -> [_ w561]
            tunnel: [_ w560] -> w556
            frame No Error {
            }
            frame Error {
              n269 = Unbundle By Name(w561) -> ("source"=w559:string)
              n270 = call-poly "CoreLib.data 2 byte array.vi"("string"=w559) -> ("byteArray out"=w560:T1)  [unwired: 18 in]
            }
          }
          n271 = Unbundle By Name(w553) -> ("code"=w558:i32)
          n272 = Bundle By Name(cluster=w549, "Data"=w556, "Error #"=w558, "Data Descriptor"="C:N") -> (w557:T2)
        }
        frame "SetChannelTripInt" {
          # "This is just an example. On how to use this VI. The names of the selector should be identical to the name of the corresponding event. Inside the false case, place the method you want to call."
          n273 = Unbundle By Name(w608) -> ("Data"=w603:T1)
          n274 = call-poly "CoreLib.byte array 2 data.vi"("byteArray"=w603, "error in (no error)"=w604) -> ("byteArray out"=w601:T1, "i32"=w597:i32, "error out"=w605:errorcluster)  [unwired: 15 in]
          n275 = call "PSChannelBase.get channel names.vi"("i ref in"=w600, "channelIndex"=w597, "error in (no error)"=w605) -> ("i ref out"=w599:refnum<vi>, "physcialName"=w598:string, "error out"=w602:errorcluster)  [unwired: 13 in, 1 out]
          n276 = call-poly "CoreLib.byte array 2 data.vi"("byteArray"=w601, "error in (no error)"=w602) -> ("d64"=w607:dbl, "error out"=w606:errorcluster)  [unwired: 15 in, 1 out]
          n277 = case shown="No Error" w606 {
            selector: w606 -> [w625 w652]
            tunnel: [w635 w655] -> w614
            tunnel: w599 -> [w627 w655]
            tunnel: [w636 w654] -> w613
            tunnel: w611 -> [_ w653]
            tunnel: w607 -> [w621 _]
            tunnel: w598 -> [w626 _]
            tunnel: w597 -> [w624 _]
            frame No Error {
              n278 = call "CAEN_HVChannel.get i attribute.vi"("i ref in"=w627, "error in (no error)"=w625) -> ("i ref out"=w628:refnum<vi>, "i attribute"=w633:T9, "error out"=w634:errorcluster)  [unwired: 15 in]
              n279 = Unbundle By Name(w633) -> ("Channel Array"=w632:T10)
              n280 = Index Array(array=w632, index=w624) -> (element=w631:T11)
              n281 = Unbundle By Name(w631) -> ("TripInt.TripInt#Multiplier"=w630:dbl, "DIM Service IDs.nomTripInt"=w623:i32)
              n282 = Divide(x=w621, y=w630) -> (x/y=w629:dbl)
              n283 = call "BaseProcess.get i attribute.vi"("i ref in"=w628, "error in (no error)"=w634) -> ("i ref out"=w647:refnum<vi>, "i attribute"=w650:T12, "error out"=w651:errorcluster)  [unwired: 15 in]
              n284 = Unbundle By Name(w650) -> ("Special"=w649:string[])
              n285 = Concatenate Strings(w626, "_nomTripInt" ("string")) -> (w638:string)
              n286 = call-poly "CoreLib.data 2 byte array.vi"("string"=w638) -> ("byteArray out"=w643:T1)  [unwired: 18 in]
              n287 = Index Array(array=w649, index=0) -> (element=w646:string)
              n288 = call-poly "CoreLib.data 2 byte array.vi"("byteArray"=w643, "f64"=w629) -> ("byteArray out"=w642:T1)  [unwired: 17 in]
              n289 = Boolean To (0,1)(Boolean=FALSE) -> (0, 1=w640:i16)
              n290 = Type Cast(x=w621) -> (*(type *) &x=w622:string)  [unwired: 1 in]
              n291 = call-poly "CoreLib.data 2 byte array.vi"("byteArray"=w642, "i16"=w640) -> ("byteArray out"=w639:T1)  [unwired: 17 in]
              n292 = call "LVDimInterface.dis_update_service.vi"("my_serviceID"=w623, "data"=w622) -> ()  [unwired: 15 in, 3 out]
              n293 = call "BaseProcess.call process 2.vi"("i ref in"=w647, "Object"=w646, "Selector"="SetValue", "Data Descriptor"="C:N;D:1;S:1", "Data"=w639, "error in (no error)"=w651) -> ("i ref out"=w635:refnum<vi>, "error out"=w636:errorcluster)  [unwired: 12 in]
            }
            frame Error {
              n294 = call "CoreLib.set data type mismatch.vi"("error in (no error)"=w652, "error source"=w653) -> ("error out"=w654:errorcluster)  [unwired: 17 in]
            }
          }
          n295 = call "BaseProcess.set event status.vi"("i ref in"=w614, "EventStatus"=w611, "error in (no error)"=w613) -> ("i ref out"=w610:refnum<vi>, "error out"=w612:errorcluster)  [unwired: 14 in, 1 out]
          n296 = case shown="Error" w612 {
            selector: w612 -> [_ w620]
            tunnel: [_ w619] -> w615
            frame No Error {
            }
            frame Error {
              n297 = Unbundle By Name(w620) -> ("source"=w618:string)
              n298 = call-poly "CoreLib.data 2 byte array.vi"("string"=w618) -> ("byteArray out"=w619:T1)  [unwired: 18 in]
            }
          }
          n299 = Unbundle By Name(w612) -> ("code"=w617:i32)
          n300 = Bundle By Name(cluster=w608, "Data"=w615, "Error #"=w617, "Data Descriptor"="C:N") -> (w616:T2)
        }
        frame "SetChannelTripExt" {
          # "This is just an example. On how to use this VI. The names of the selector should be identical to the name of the corresponding event. Inside the false case, place the method you want to call."
          n301 = Unbundle By Name(w667) -> ("Data"=w662:T1)
          n302 = call-poly "CoreLib.byte array 2 data.vi"("byteArray"=w662, "error in (no error)"=w663) -> ("byteArray out"=w660:T1, "i32"=w656:i32, "error out"=w664:errorcluster)  [unwired: 15 in]
          n303 = call "PSChannelBase.get channel names.vi"("i ref in"=w659, "channelIndex"=w656, "error in (no error)"=w664) -> ("i ref out"=w658:refnum<vi>, "physcialName"=w657:string, "error out"=w661:errorcluster)  [unwired: 13 in, 1 out]
          n304 = call-poly "CoreLib.byte array 2 data.vi"("byteArray"=w660, "error in (no error)"=w661) -> ("d64"=w666:dbl, "error out"=w665:errorcluster)  [unwired: 15 in, 1 out]
          n305 = case shown="No Error" w665 {
            selector: w665 -> [w684 w711]
            tunnel: [w694 w714] -> w673
            tunnel: w658 -> [w686 w714]
            tunnel: [w695 w713] -> w672
            tunnel: w670 -> [_ w712]
            tunnel: w666 -> [w680 _]
            tunnel: w657 -> [w685 _]
            tunnel: w656 -> [w683 _]
            frame No Error {
              n306 = call "CAEN_HVChannel.get i attribute.vi"("i ref in"=w686, "error in (no error)"=w684) -> ("i ref out"=w687:refnum<vi>, "i attribute"=w692:T9, "error out"=w693:errorcluster)  [unwired: 15 in]
              n307 = Unbundle By Name(w692) -> ("Channel Array"=w691:T10)
              n308 = Index Array(array=w691, index=w683) -> (element=w690:T11)
              n309 = Unbundle By Name(w690) -> ("TripExt.TripExt#Multiplier"=w689:dbl, "DIM Service IDs.nomTripExt"=w682:i32)
              n310 = Divide(x=w680, y=w689) -> (x/y=w688:dbl)
              n311 = call "BaseProcess.get i attribute.vi"("i ref in"=w687, "error in (no error)"=w693) -> ("i ref out"=w706:refnum<vi>, "i attribute"=w709:T12, "error out"=w710:errorcluster)  [unwired: 15 in]
              n312 = Unbundle By Name(w709) -> ("Special"=w708:string[])
              n313 = Concatenate Strings(w685, "_nomTripExt" ("string")) -> (w697:string)
              n314 = call-poly "CoreLib.data 2 byte array.vi"("string"=w697) -> ("byteArray out"=w702:T1)  [unwired: 18 in]
              n315 = Index Array(array=w708, index=0) -> (element=w705:string)
              n316 = call-poly "CoreLib.data 2 byte array.vi"("byteArray"=w702, "f64"=w688) -> ("byteArray out"=w701:T1)  [unwired: 17 in]
              n317 = Boolean To (0,1)(Boolean=FALSE) -> (0, 1=w699:i16)
              n318 = Type Cast(x=w680) -> (*(type *) &x=w681:string)  [unwired: 1 in]
              n319 = call-poly "CoreLib.data 2 byte array.vi"("byteArray"=w701, "i16"=w699) -> ("byteArray out"=w698:T1)  [unwired: 17 in]
              n320 = call "LVDimInterface.dis_update_service.vi"("my_serviceID"=w682, "data"=w681) -> ()  [unwired: 15 in, 3 out]
              n321 = call "BaseProcess.call process 2.vi"("i ref in"=w706, "Object"=w705, "Selector"="SetValue", "Data Descriptor"="C:N;D:1;S:1", "Data"=w698, "error in (no error)"=w710) -> ("i ref out"=w694:refnum<vi>, "error out"=w695:errorcluster)  [unwired: 12 in]
            }
            frame Error {
              n322 = call "CoreLib.set data type mismatch.vi"("error in (no error)"=w711, "error source"=w712) -> ("error out"=w713:errorcluster)  [unwired: 17 in]
            }
          }
          n323 = call "BaseProcess.set event status.vi"("i ref in"=w673, "EventStatus"=w670, "error in (no error)"=w672) -> ("i ref out"=w669:refnum<vi>, "error out"=w671:errorcluster)  [unwired: 14 in, 1 out]
          n324 = case shown="Error" w671 {
            selector: w671 -> [_ w679]
            tunnel: [_ w678] -> w674
            frame No Error {
            }
            frame Error {
              n325 = Unbundle By Name(w679) -> ("source"=w677:string)
              n326 = call-poly "CoreLib.data 2 byte array.vi"("string"=w677) -> ("byteArray out"=w678:T1)  [unwired: 18 in]
            }
          }
          n327 = Unbundle By Name(w671) -> ("code"=w676:i32)
          n328 = Bundle By Name(cluster=w667, "Data"=w674, "Error #"=w676, "Data Descriptor"="C:N") -> (w675:T2)
        }
        frame "SetChannelSVMax" {
          # "This is just an example. On how to use this VI. The names of the selector should be identical to the name of the corresponding event. Inside the false case, place the method you want to call."
          n329 = Unbundle By Name(w726) -> ("Data"=w721:T1)
          n330 = call-poly "CoreLib.byte array 2 data.vi"("byteArray"=w721, "error in (no error)"=w722) -> ("byteArray out"=w719:T1, "i32"=w715:i32, "error out"=w723:errorcluster)  [unwired: 15 in]
          n331 = call "PSChannelBase.get channel names.vi"("i ref in"=w718, "channelIndex"=w715, "error in (no error)"=w723) -> ("i ref out"=w717:refnum<vi>, "physcialName"=w716:string, "error out"=w720:errorcluster)  [unwired: 13 in, 1 out]
          n332 = call-poly "CoreLib.byte array 2 data.vi"("byteArray"=w719, "error in (no error)"=w720) -> ("d64"=w725:dbl, "error out"=w724:errorcluster)  [unwired: 15 in, 1 out]
          n333 = case shown="No Error" w724 {
            selector: w724 -> [w743 w770]
            tunnel: [w753 w773] -> w732
            tunnel: w717 -> [w745 w773]
            tunnel: [w754 w772] -> w731
            tunnel: w729 -> [_ w771]
            tunnel: w725 -> [w739 _]
            tunnel: w716 -> [w744 _]
            tunnel: w715 -> [w742 _]
            frame No Error {
              n334 = call "CAEN_HVChannel.get i attribute.vi"("i ref in"=w745, "error in (no error)"=w743) -> ("i ref out"=w746:refnum<vi>, "i attribute"=w751:T9, "error out"=w752:errorcluster)  [unwired: 15 in]
              n335 = Unbundle By Name(w751) -> ("Channel Array"=w750:T10)
              n336 = Index Array(array=w750, index=w742) -> (element=w749:T11)
              n337 = Unbundle By Name(w749) -> ("SVMax.SVMax#Multiplier"=w748:dbl, "DIM Service IDs.nomSVMax"=w741:i32)
              n338 = Divide(x=w739, y=w748) -> (x/y=w747:dbl)
              n339 = call "BaseProcess.get i attribute.vi"("i ref in"=w746, "error in (no error)"=w752) -> ("i ref out"=w765:refnum<vi>, "i attribute"=w768:T12, "error out"=w769:errorcluster)  [unwired: 15 in]
              n340 = Unbundle By Name(w768) -> ("Special"=w767:string[])
              n341 = Concatenate Strings(w744, "_nomSVMax" ("string")) -> (w756:string)
              n342 = call-poly "CoreLib.data 2 byte array.vi"("string"=w756) -> ("byteArray out"=w761:T1)  [unwired: 18 in]
              n343 = Index Array(array=w767, index=0) -> (element=w764:string)
              n344 = call-poly "CoreLib.data 2 byte array.vi"("byteArray"=w761, "f64"=w747) -> ("byteArray out"=w760:T1)  [unwired: 17 in]
              n345 = Boolean To (0,1)(Boolean=FALSE) -> (0, 1=w758:i16)
              n346 = Type Cast(x=w739) -> (*(type *) &x=w740:string)  [unwired: 1 in]
              n347 = call-poly "CoreLib.data 2 byte array.vi"("byteArray"=w760, "i16"=w758) -> ("byteArray out"=w757:T1)  [unwired: 17 in]
              n348 = call "LVDimInterface.dis_update_service.vi"("my_serviceID"=w741, "data"=w740) -> ()  [unwired: 15 in, 3 out]
              n349 = call "BaseProcess.call process 2.vi"("i ref in"=w765, "Object"=w764, "Selector"="SetValue", "Data Descriptor"="C:N;D:1;S:1", "Data"=w757, "error in (no error)"=w769) -> ("i ref out"=w753:refnum<vi>, "error out"=w754:errorcluster)  [unwired: 12 in]
            }
            frame Error {
              n350 = call "CoreLib.set data type mismatch.vi"("error in (no error)"=w770, "error source"=w771) -> ("error out"=w772:errorcluster)  [unwired: 17 in]
            }
          }
          n351 = call "BaseProcess.set event status.vi"("i ref in"=w732, "EventStatus"=w729, "error in (no error)"=w731) -> ("i ref out"=w728:refnum<vi>, "error out"=w730:errorcluster)  [unwired: 14 in, 1 out]
          n352 = case shown="Error" w730 {
            selector: w730 -> [_ w738]
            tunnel: [_ w737] -> w733
            frame No Error {
            }
            frame Error {
              n353 = Unbundle By Name(w738) -> ("source"=w736:string)
              n354 = call-poly "CoreLib.data 2 byte array.vi"("string"=w736) -> ("byteArray out"=w737:T1)  [unwired: 18 in]
            }
          }
          n355 = Unbundle By Name(w730) -> ("code"=w735:i32)
          n356 = Bundle By Name(cluster=w726, "Data"=w733, "Error #"=w735, "Data Descriptor"="C:N") -> (w734:T2)
        }
        frame "SetChannelPwrOnOption" {
          # "This is just an example. On how to use this VI. The names of the selector should be identical to the name of the corresponding event. Inside the false case, place the method you want to call."
          n357 = Unbundle By Name(w785) -> ("Data"=w780:T1)
          n358 = call-poly "CoreLib.byte array 2 data.vi"("byteArray"=w780, "error in (no error)"=w781) -> ("byteArray out"=w778:T1, "i32"=w774:i32, "error out"=w782:errorcluster)  [unwired: 15 in]
          n359 = call "PSChannelBase.get channel names.vi"("i ref in"=w777, "channelIndex"=w774, "error in (no error)"=w782) -> ("i ref out"=w776:refnum<vi>, "physcialName"=w775:string, "error out"=w779:errorcluster)  [unwired: 13 in, 1 out]
          n360 = call-poly "CoreLib.byte array 2 data.vi"("byteArray"=w778, "error in (no error)"=w779) -> ("i16"=w784:i16, "error out"=w783:errorcluster)  [unwired: 15 in, 1 out]
          n361 = case shown="No Error" w783 {
            selector: w783 -> [w802 w827]
            tunnel: [w810 w830] -> w791
            tunnel: w776 -> [w804 w830]
            tunnel: [w811 w829] -> w790
            tunnel: w788 -> [_ w828]
            tunnel: w784 -> [w798 _]
            tunnel: w775 -> [w803 _]
            tunnel: w774 -> [w801 _]
            frame No Error {
              n362 = call "CAEN_HVChannel.get i attribute.vi"("i ref in"=w804, "error in (no error)"=w802) -> ("i ref out"=w805:refnum<vi>, "i attribute"=w808:T9, "error out"=w809:errorcluster)  [unwired: 15 in]
              n363 = Unbundle By Name(w808) -> ("Channel Array"=w807:T10)
              n364 = Index Array(array=w807, index=w801) -> (element=w806:T11)
              n365 = Unbundle By Name(w806) -> ("DIM Service IDs.nomPDwn"=w800:i32)
              n366 = call "BaseProcess.get i attribute.vi"("i ref in"=w805, "error in (no error)"=w809) -> ("i ref out"=w822:refnum<vi>, "i attribute"=w825:T12, "error out"=w826:errorcluster)  [unwired: 15 in]
              n367 = Unbundle By Name(w825) -> ("Special"=w824:string[])
              n368 = Concatenate Strings(w803, "_nomPOn" ("string")) -> (w813:string)
              n369 = call-poly "CoreLib.data 2 byte array.vi"("string"=w813) -> ("byteArray out"=w818:T1)  [unwired: 18 in]
              n370 = Index Array(array=w824, index=0) -> (element=w821:string)
              n371 = call-poly "CoreLib.data 2 byte array.vi"("byteArray"=w818, "f64"=w798) -> ("byteArray out"=w817:T1)  [unwired: 17 in]
              n372 = Boolean To (0,1)(Boolean=FALSE) -> (0, 1=w815:i16)
              n373 = Type Cast(x=w798) -> (*(type *) &x=w799:string)  [unwired: 1 in]
              n374 = call-poly "CoreLib.data 2 byte array.vi"("byteArray"=w817, "i16"=w815) -> ("byteArray out"=w814:T1)  [unwired: 17 in]
              n375 = call "LVDimInterface.dis_update_service.vi"("my_serviceID"=w800, "data"=w799) -> ()  [unwired: 15 in, 3 out]
              n376 = call "BaseProcess.call process 2.vi"("i ref in"=w822, "Object"=w821, "Selector"="SetValue", "Data Descriptor"="C:N;S:1;S:1", "Data"=w814, "error in (no error)"=w826) -> ("i ref out"=w810:refnum<vi>, "error out"=w811:errorcluster)  [unwired: 12 in]
            }
            frame Error {
              n377 = call "CoreLib.set data type mismatch.vi"("error in (no error)"=w827, "error source"=w828) -> ("error out"=w829:errorcluster)  [unwired: 17 in]
            }
          }
          n378 = call "BaseProcess.set event status.vi"("i ref in"=w791, "EventStatus"=w788, "error in (no error)"=w790) -> ("i ref out"=w787:refnum<vi>, "error out"=w789:errorcluster)  [unwired: 14 in, 1 out]
          n379 = case shown="Error" w789 {
            selector: w789 -> [_ w797]
            tunnel: [_ w796] -> w792
            frame No Error {
            }
            frame Error {
              n380 = Unbundle By Name(w797) -> ("source"=w795:string)
              n381 = call-poly "CoreLib.data 2 byte array.vi"("string"=w795) -> ("byteArray out"=w796:T1)  [unwired: 18 in]
            }
          }
          n382 = Unbundle By Name(w789) -> ("code"=w794:i32)
          n383 = Bundle By Name(cluster=w785, "Data"=w792, "Error #"=w794, "Data Descriptor"="C:N") -> (w793:T2)
        }
        frame "SetChannelPwrDwnOption" {
          # "This is just an example. On how to use this VI. The names of the selector should be identical to the name of the corresponding event. Inside the false case, place the method you want to call."
          n384 = Unbundle By Name(w842) -> ("Data"=w837:T1)
          n385 = call-poly "CoreLib.byte array 2 data.vi"("byteArray"=w837, "error in (no error)"=w838) -> ("byteArray out"=w835:T1, "i32"=w831:i32, "error out"=w839:errorcluster)  [unwired: 15 in]
          n386 = call "PSChannelBase.get channel names.vi"("i ref in"=w834, "channelIndex"=w831, "error in (no error)"=w839) -> ("i ref out"=w833:refnum<vi>, "physcialName"=w832:string, "error out"=w836:errorcluster)  [unwired: 13 in, 1 out]
          n387 = call-poly "CoreLib.byte array 2 data.vi"("byteArray"=w835, "error in (no error)"=w836) -> ("i16"=w841:i16, "error out"=w840:errorcluster)  [unwired: 15 in, 1 out]
          n388 = case shown="No Error" w840 {
            selector: w840 -> [w859 w884]
            tunnel: [w867 w887] -> w848
            tunnel: w833 -> [w861 w887]
            tunnel: [w868 w886] -> w847
            tunnel: w845 -> [_ w885]
            tunnel: w841 -> [w855 _]
            tunnel: w832 -> [w860 _]
            tunnel: w831 -> [w858 _]
            frame No Error {
              n389 = call "CAEN_HVChannel.get i attribute.vi"("i ref in"=w861, "error in (no error)"=w859) -> ("i ref out"=w862:refnum<vi>, "i attribute"=w865:T9, "error out"=w866:errorcluster)  [unwired: 15 in]
              n390 = Unbundle By Name(w865) -> ("Channel Array"=w864:T10)
              n391 = Index Array(array=w864, index=w858) -> (element=w863:T11)
              n392 = Unbundle By Name(w863) -> ("DIM Service IDs.nomPDwn"=w857:i32)
              n393 = call "BaseProcess.get i attribute.vi"("i ref in"=w862, "error in (no error)"=w866) -> ("i ref out"=w879:refnum<vi>, "i attribute"=w882:T12, "error out"=w883:errorcluster)  [unwired: 15 in]
              n394 = Unbundle By Name(w882) -> ("Special"=w881:string[])
              n395 = Concatenate Strings(w860, "_nomPDwn" ("string")) -> (w870:string)
              n396 = call-poly "CoreLib.data 2 byte array.vi"("string"=w870) -> ("byteArray out"=w875:T1)  [unwired: 18 in]
              n397 = Index Array(array=w881, index=0) -> (element=w878:string)
              n398 = call-poly "CoreLib.data 2 byte array.vi"("byteArray"=w875, "f64"=w855) -> ("byteArray out"=w874:T1)  [unwired: 17 in]
              n399 = Boolean To (0,1)(Boolean=FALSE) -> (0, 1=w872:i16)
              n400 = Type Cast(x=w855) -> (*(type *) &x=w856:string)  [unwired: 1 in]
              n401 = call-poly "CoreLib.data 2 byte array.vi"("byteArray"=w874, "i16"=w872) -> ("byteArray out"=w871:T1)  [unwired: 17 in]
              n402 = call "LVDimInterface.dis_update_service.vi"("my_serviceID"=w857, "data"=w856) -> ()  [unwired: 15 in, 3 out]
              n403 = call "BaseProcess.call process 2.vi"("i ref in"=w879, "Object"=w878, "Selector"="SetValue", "Data Descriptor"="C:N;S:1;S:1", "Data"=w871, "error in (no error)"=w883) -> ("i ref out"=w867:refnum<vi>, "error out"=w868:errorcluster)  [unwired: 12 in]
            }
            frame Error {
              n404 = call "CoreLib.set data type mismatch.vi"("error in (no error)"=w884, "error source"=w885) -> ("error out"=w886:errorcluster)  [unwired: 17 in]
            }
          }
          n405 = call "BaseProcess.set event status.vi"("i ref in"=w848, "EventStatus"=w845, "error in (no error)"=w847) -> ("i ref out"=w844:refnum<vi>, "error out"=w846:errorcluster)  [unwired: 14 in, 1 out]
          n406 = case shown="Error" w846 {
            selector: w846 -> [_ w854]
            tunnel: [_ w853] -> w849
            frame No Error {
            }
            frame Error {
              n407 = Unbundle By Name(w854) -> ("source"=w852:string)
              n408 = call-poly "CoreLib.data 2 byte array.vi"("string"=w852) -> ("byteArray out"=w853:T1)  [unwired: 18 in]
            }
          }
          n409 = Unbundle By Name(w846) -> ("code"=w851:i32)
          n410 = Bundle By Name(cluster=w842, "Data"=w849, "Error #"=w851, "Data Descriptor"="C:N") -> (w850:T2)
        }
        frame "SetChannelOnOff" {
          # "This is just an example. On how to use this VI. The names of the selector should be identical to the name of the corresponding event. Inside the false case, place the method you want to call."
          n411 = Unbundle By Name(w899) -> ("Data"=w894:T1)
          n412 = call-poly "CoreLib.byte array 2 data.vi"("byteArray"=w894, "error in (no error)"=w895) -> ("byteArray out"=w892:T1, "i32"=w888:i32, "error out"=w896:errorcluster)  [unwired: 15 in]
          n413 = call "PSChannelBase.get channel names.vi"("i ref in"=w891, "channelIndex"=w888, "error in (no error)"=w896) -> ("i ref out"=w890:refnum<vi>, "physcialName"=w889:string, "error out"=w893:errorcluster)  [unwired: 13 in, 1 out]
          n414 = call-poly "CoreLib.byte array 2 data.vi"("byteArray"=w892, "error in (no error)"=w893) -> ("i16"=w898:i16, "error out"=w897:errorcluster)  [unwired: 15 in, 1 out]
          n415 = case shown="No Error" w897 {
            selector: w897 -> [w914 w938]
            tunnel: [w918 w941] -> w905
            tunnel: w890 -> [w915 w941]
            tunnel: [w919 w940] -> w904
            tunnel: w902 -> [_ w939]
            tunnel: w898 -> [w913 _]
            tunnel: w889 -> [w917 _]
            tunnel: w888 -> [w916 _]
            frame No Error {
              n416 = call "BaseProcess.get i attribute.vi"("i ref in"=w915, "error in (no error)"=w914) -> ("i ref out"=w930:refnum<vi>, "i attribute"=w933:T12, "error out"=w934:errorcluster)  [unwired: 15 in]
              n417 = Unbundle By Name(w933) -> ("Special"=w932:string[])
              n418 = Concatenate Strings(w917, "_nomPw" ("string")) -> (w921:string)
              n419 = call-poly "CoreLib.data 2 byte array.vi"("string"=w921) -> ("byteArray out"=w926:T1)  [unwired: 18 in]
              n420 = Index Array(array=w932, index=0) -> (element=w929:string)
              n421 = Not Equal To 0?(x=w913) -> (x != 0?=w912:bool)
              n422 = call-poly "CoreLib.data 2 byte array.vi"("byteArray"=w926, "i16"=w913) -> ("byteArray out"=w925:T1)  [unwired: 17 in]
              n423 = Boolean To (0,1)(Boolean=FALSE) -> (0, 1=w923:i16)
              n424 = call-poly "CoreLib.data 2 byte array.vi"("byteArray"=w925, "i16"=w923) -> ("byteArray out"=w922:T1)  [unwired: 17 in]
              n425 = call "BaseProcess.call process 2.vi"("i ref in"=w930, "Object"=w929, "Selector"="SetValue", "Data Descriptor"="C:N;S:1;S:1", "Data"=w922, "error in (no error)"=w934) -> ("i ref out"=w918:refnum<vi>, "error out"=w919:errorcluster)  [unwired: 12 in]
              n426 = Type Cast(x=w912) -> (*(type *) &x=w937:string)  [unwired: 1 in]
              n427 = call "PSChannelBase.update services and attribute data.vi"("i ref in"=w918, "direction"=PSChannelBase.directionType."update nominal value", "service"=PSChannelBase.serviceType."onOff", "value"=w937, "channelNumber"=w916) -> ()  [unwired: 12 in, 3 out]
            }
            frame Error {
              n428 = call "CoreLib.set data type mismatch.vi"("error in (no error)"=w938, "error source"=w939) -> ("error out"=w940:errorcluster)  [unwired: 17 in]
            }
          }
          n429 = call "BaseProcess.set event status.vi"("i ref in"=w905, "EventStatus"=w902, "error in (no error)"=w904) -> ("i ref out"=w901:refnum<vi>, "error out"=w903:errorcluster)  [unwired: 14 in, 1 out]
          n430 = case shown="No Error" w903 {
            selector: w903 -> [_ w911]
            tunnel: [_ w910] -> w906
            frame No Error {
            }
            frame Error {
              n431 = Unbundle By Name(w911) -> ("source"=w909:string)
              n432 = call-poly "CoreLib.data 2 byte array.vi"("string"=w909) -> ("byteArray out"=w910:T1)  [unwired: 18 in]
            }
          }
          n433 = Unbundle By Name(w903) -> ("code"=w908:i32)
          n434 = Bundle By Name(cluster=w899, "Data"=w906, "Error #"=w908, "Data Descriptor"="C:N") -> (w907:T2)
        }
        frame "SetChannelTripCurrent" {
          # "This is just an example. On how to use this VI. The names of the selector should be identical to the name of the corresponding event. Inside the false case, place the method you want to call."
          n435 = Unbundle By Name(w953) -> ("Data"=w948:T1)
          n436 = call-poly "CoreLib.byte array 2 data.vi"("byteArray"=w948, "error in (no error)"=w949) -> ("byteArray out"=w946:T1, "i32"=w942:i32, "error out"=w950:errorcluster)  [unwired: 15 in]
          n437 = call "PSChannelBase.get channel names.vi"("i ref in"=w945, "channelIndex"=w942, "error in (no error)"=w950) -> ("i ref out"=w944:refnum<vi>, "physcialName"=w943:string, "error out"=w947:errorcluster)  [unwired: 13 in, 1 out]
          n438 = call-poly "CoreLib.byte array 2 data.vi"("byteArray"=w946, "error in (no error)"=w947) -> ("d64"=w952:dbl, "error out"=w951:errorcluster)  [unwired: 15 in, 1 out]
          n439 = case shown="No Error" w951 {
            selector: w951 -> [w967 w998]
            tunnel: [w978 w1001] -> w959
            tunnel: w944 -> [w969 w1001]
            tunnel: [w979 w1000] -> w958
            tunnel: w956 -> [_ w999]
            tunnel: w952 -> [w972 _]
            tunnel: w943 -> [w968 _]
            tunnel: w942 -> [w966 _]
            frame No Error {
              n440 = call "CAEN_HVChannel.get i attribute.vi"("i ref in"=w969, "error in (no error)"=w967) -> ("i ref out"=w970:refnum<vi>, "i attribute"=w976:T9, "error out"=w977:errorcluster)  [unwired: 15 in]
              n441 = Unbundle By Name(w976) -> ("Channel Array"=w975:T10)
              n442 = Index Array(array=w975, index=w966) -> (element=w974:T11)
              n443 = Unbundle By Name(w974) -> ("I0Set.I0Set#Multiplier"=w973:dbl)
              n444 = Divide(x=w972, y=w973) -> (x/y=w971:dbl)
              n445 = call "BaseProcess.get i attribute.vi"("i ref in"=w970, "error in (no error)"=w977) -> ("i ref out"=w990:refnum<vi>, "i attribute"=w993:T12, "error out"=w994:errorcluster)  [unwired: 15 in]
              n446 = Unbundle By Name(w993) -> ("Special"=w992:string[])
              n447 = Concatenate Strings(w968, "_nomI0Set" ("string")) -> (w981:string)
              n448 = call-poly "CoreLib.data 2 byte array.vi"("string"=w981) -> ("byteArray out"=w986:T1)  [unwired: 18 in]
              n449 = Index Array(array=w992, index=0) -> (element=w989:string)
              n450 = call-poly "CoreLib.data 2 byte array.vi"("byteArray"=w986, "f64"=w971) -> ("byteArray out"=w985:T1)  [unwired: 17 in]
              n451 = Boolean To (0,1)(Boolean=FALSE) -> (0, 1=w983:i16)
              n452 = call-poly "CoreLib.data 2 byte array.vi"("byteArray"=w985, "i16"=w983) -> ("byteArray out"=w982:T1)  [unwired: 17 in]
              n453 = call "BaseProcess.call process 2.vi"("i ref in"=w990, "Object"=w989, "Selector"="SetValue", "Data Descriptor"="C:N;D:1;S:1", "Data"=w982, "error in (no error)"=w994) -> ("i ref out"=w978:refnum<vi>, "error out"=w979:errorcluster)  [unwired: 12 in]
              n454 = Type Cast(x=w972) -> (*(type *) &x=w997:string)  [unwired: 1 in]
              n455 = call "PSChannelBase.update services and attribute data.vi"("i ref in"=w978, "direction"=PSChannelBase.directionType."update nominal value", "service"=PSChannelBase.serviceType."tripCurrent", "value"=w997, "channelNumber"=w966) -> ()  [unwired: 12 in, 3 out]
            }
            frame Error {
              n456 = call "CoreLib.set data type mismatch.vi"("error in (no error)"=w998, "error source"=w999) -> ("error out"=w1000:errorcluster)  [unwired: 17 in]
            }
          }
          n457 = call "BaseProcess.set event status.vi"("i ref in"=w959, "EventStatus"=w956, "error in (no error)"=w958) -> ("i ref out"=w955:refnum<vi>, "error out"=w957:errorcluster)  [unwired: 14 in, 1 out]
          n458 = case shown="Error" w957 {
            selector: w957 -> [_ w965]
            tunnel: [_ w964] -> w960
            frame No Error {
            }
            frame Error {
              n459 = Unbundle By Name(w965) -> ("source"=w963:string)
              n460 = call-poly "CoreLib.data 2 byte array.vi"("string"=w963) -> ("byteArray out"=w964:T1)  [unwired: 18 in]
            }
          }
          n461 = Unbundle By Name(w957) -> ("code"=w962:i32)
          n462 = Bundle By Name(cluster=w953, "Data"=w960, "Error #"=w962, "Data Descriptor"="C:N") -> (w961:T2)
        }
        frame "SetChannelRampUpSpeed" {
          # "This is just an example. On how to use this VI. The names of the selector should be identical to the name of the corresponding event. Inside the false case, place the method you want to call."
          n463 = Unbundle By Name(w1013) -> ("Data"=w1008:T1)
          n464 = call-poly "CoreLib.byte array 2 data.vi"("byteArray"=w1008, "error in (no error)"=w1009) -> ("byteArray out"=w1006:T1, "i32"=w1002:i32, "error out"=w1010:errorcluster)  [unwired: 15 in]
          n465 = call "PSChannelBase.get channel names.vi"("i ref in"=w1005, "channelIndex"=w1002, "error in (no error)"=w1010) -> ("i ref out"=w1004:refnum<vi>, "physcialName"=w1003:string, "error out"=w1007:errorcluster)  [unwired: 13 in, 1 out]
          n466 = call-poly "CoreLib.byte array 2 data.vi"("byteArray"=w1006, "error in (no error)"=w1007) -> ("d64"=w1012:dbl, "error out"=w1011:errorcluster)  [unwired: 15 in, 1 out]
          n467 = case shown="No Error" w1011 {
            selector: w1011 -> [w1027 w1058]
            tunnel: [w1038 w1061] -> w1019
            tunnel: w1004 -> [w1029 w1061]
            tunnel: [w1039 w1060] -> w1018
            tunnel: w1016 -> [_ w1059]
            tunnel: w1012 -> [w1032 _]
            tunnel: w1003 -> [w1028 _]
            tunnel: w1002 -> [w1026 _]
            frame No Error {
              n468 = call "CAEN_HVChannel.get i attribute.vi"("i ref in"=w1029, "error in (no error)"=w1027) -> ("i ref out"=w1030:refnum<vi>, "i attribute"=w1036:T9, "error out"=w1037:errorcluster)  [unwired: 15 in]
              n469 = Unbundle By Name(w1036) -> ("Channel Array"=w1035:T10)
              n470 = Index Array(array=w1035, index=w1026) -> (element=w1034:T11)
              n471 = Unbundle By Name(w1034) -> ("RUp.RUp#Multiplier"=w1033:dbl)
              n472 = Divide(x=w1032, y=w1033) -> (x/y=w1031:dbl)
              n473 = call "BaseProcess.get i attribute.vi"("i ref in"=w1030, "error in (no error)"=w1037) -> ("i ref out"=w1050:refnum<vi>, "i attribute"=w1053:T12, "error out"=w1054:errorcluster)  [unwired: 15 in]
              n474 = Unbundle By Name(w1053) -> ("Special"=w1052:string[])
              n475 = Concatenate Strings(w1028, "_nomRUp" ("string")) -> (w1041:string)
              n476 = call-poly "CoreLib.data 2 byte array.vi"("string"=w1041) -> ("byteArray out"=w1046:T1)  [unwired: 18 in]
              n477 = Index Array(array=w1052, index=0) -> (element=w1049:string)
              n478 = call-poly "CoreLib.data 2 byte array.vi"("byteArray"=w1046, "f64"=w1031) -> ("byteArray out"=w1045:T1)  [unwired: 17 in]
              n479 = Boolean To (0,1)(Boolean=FALSE) -> (0, 1=w1043:i16)
              n480 = call-poly "CoreLib.data 2 byte array.vi"("byteArray"=w1045, "i16"=w1043) -> ("byteArray out"=w1042:T1)  [unwired: 17 in]
              n481 = call "BaseProcess.call process 2.vi"("i ref in"=w1050, "Object"=w1049, "Selector"="SetValue", "Data Descriptor"="C:N;D:1;S:1", "Data"=w1042, "error in (no error)"=w1054) -> ("i ref out"=w1038:refnum<vi>, "error out"=w1039:errorcluster)  [unwired: 12 in]
              n482 = Type Cast(x=w1032) -> (*(type *) &x=w1057:string)  [unwired: 1 in]
              n483 = call "PSChannelBase.update services and attribute data.vi"("i ref in"=w1038, "direction"=PSChannelBase.directionType."update nominal value", "service"=PSChannelBase.serviceType."rampUpSpeed", "value"=w1057, "channelNumber"=w1026) -> ()  [unwired: 12 in, 3 out]
            }
            frame Error {
              n484 = call "CoreLib.set data type mismatch.vi"("error in (no error)"=w1058, "error source"=w1059) -> ("error out"=w1060:errorcluster)  [unwired: 17 in]
            }
          }
          n485 = call "BaseProcess.set event status.vi"("i ref in"=w1019, "EventStatus"=w1016, "error in (no error)"=w1018) -> ("i ref out"=w1015:refnum<vi>, "error out"=w1017:errorcluster)  [unwired: 14 in, 1 out]
          n486 = case shown="Error" w1017 {
            selector: w1017 -> [_ w1025]
            tunnel: [_ w1024] -> w1020
            frame No Error {
            }
            frame Error {
              n487 = Unbundle By Name(w1025) -> ("source"=w1023:string)
              n488 = call-poly "CoreLib.data 2 byte array.vi"("string"=w1023) -> ("byteArray out"=w1024:T1)  [unwired: 18 in]
            }
          }
          n489 = Unbundle By Name(w1017) -> ("code"=w1022:i32)
          n490 = Bundle By Name(cluster=w1013, "Data"=w1020, "Error #"=w1022, "Data Descriptor"="C:N") -> (w1021:T2)
        }
        frame "SetChannelRampDownSpeed" {
          # "This is just an example. On how to use this VI. The names of the selector should be identical to the name of the corresponding event. Inside the false case, place the method you want to call."
          n491 = Unbundle By Name(w1073) -> ("Data"=w1068:T1)
          n492 = call-poly "CoreLib.byte array 2 data.vi"("byteArray"=w1068, "error in (no error)"=w1069) -> ("byteArray out"=w1066:T1, "i32"=w1062:i32, "error out"=w1070:errorcluster)  [unwired: 15 in]
          n493 = call "PSChannelBase.get channel names.vi"("i ref in"=w1065, "channelIndex"=w1062, "error in (no error)"=w1070) -> ("i ref out"=w1064:refnum<vi>, "physcialName"=w1063:string, "error out"=w1067:errorcluster)  [unwired: 13 in, 1 out]
          n494 = call-poly "CoreLib.byte array 2 data.vi"("byteArray"=w1066, "error in (no error)"=w1067) -> ("d64"=w1072:dbl, "error out"=w1071:errorcluster)  [unwired: 15 in, 1 out]
          n495 = case shown="No Error" w1071 {
            selector: w1071 -> [w1087 w1118]
            tunnel: [w1098 w1121] -> w1079
            tunnel: w1064 -> [w1089 w1121]
            tunnel: [w1099 w1120] -> w1078
            tunnel: w1076 -> [_ w1119]
            tunnel: w1072 -> [w1092 _]
            tunnel: w1063 -> [w1088 _]
            tunnel: w1062 -> [w1086 _]
            frame No Error {
              n496 = call "CAEN_HVChannel.get i attribute.vi"("i ref in"=w1089, "error in (no error)"=w1087) -> ("i ref out"=w1090:refnum<vi>, "i attribute"=w1096:T9, "error out"=w1097:errorcluster)  [unwired: 15 in]
              n497 = Unbundle By Name(w1096) -> ("Channel Array"=w1095:T10)
              n498 = Index Array(array=w1095, index=w1086) -> (element=w1094:T11)
              n499 = Unbundle By Name(w1094) -> ("RDWn.RDWn#Multiplier"=w1093:dbl)
              n500 = Divide(x=w1092, y=w1093) -> (x/y=w1091:dbl)
              n501 = call "BaseProcess.get i attribute.vi"("i ref in"=w1090, "error in (no error)"=w1097) -> ("i ref out"=w1110:refnum<vi>, "i attribute"=w1113:T12, "error out"=w1114:errorcluster)  [unwired: 15 in]
              n502 = Unbundle By Name(w1113) -> ("Special"=w1112:string[])
              n503 = Concatenate Strings(w1088, "_nomRDWn" ("string")) -> (w1101:string)
              n504 = call-poly "CoreLib.data 2 byte array.vi"("string"=w1101) -> ("byteArray out"=w1106:T1)  [unwired: 18 in]
              n505 = Index Array(array=w1112, index=0) -> (element=w1109:string)
              n506 = call-poly "CoreLib.data 2 byte array.vi"("byteArray"=w1106, "f64"=w1091) -> ("byteArray out"=w1105:T1)  [unwired: 17 in]
              n507 = Boolean To (0,1)(Boolean=FALSE) -> (0, 1=w1103:i16)
              n508 = call-poly "CoreLib.data 2 byte array.vi"("byteArray"=w1105, "i16"=w1103) -> ("byteArray out"=w1102:T1)  [unwired: 17 in]
              n509 = call "BaseProcess.call process 2.vi"("i ref in"=w1110, "Object"=w1109, "Selector"="SetValue", "Data Descriptor"="C:N;D:1;S:1", "Data"=w1102, "error in (no error)"=w1114) -> ("i ref out"=w1098:refnum<vi>, "error out"=w1099:errorcluster)  [unwired: 12 in]
              n510 = Type Cast(x=w1092) -> (*(type *) &x=w1117:string)  [unwired: 1 in]
              n511 = call "PSChannelBase.update services and attribute data.vi"("i ref in"=w1098, "direction"=PSChannelBase.directionType."update nominal value", "service"=PSChannelBase.serviceType."rampDownSpeed", "value"=w1117, "channelNumber"=w1086) -> ()  [unwired: 12 in, 3 out]
            }
            frame Error {
              n512 = call "CoreLib.set data type mismatch.vi"("error in (no error)"=w1118, "error source"=w1119) -> ("error out"=w1120:errorcluster)  [unwired: 17 in]
            }
          }
          n513 = call "BaseProcess.set event status.vi"("i ref in"=w1079, "EventStatus"=w1076, "error in (no error)"=w1078) -> ("i ref out"=w1075:refnum<vi>, "error out"=w1077:errorcluster)  [unwired: 14 in, 1 out]
          n514 = case shown="Error" w1077 {
            selector: w1077 -> [_ w1085]
            tunnel: [_ w1084] -> w1080
            frame No Error {
            }
            frame Error {
              n515 = Unbundle By Name(w1085) -> ("source"=w1083:string)
              n516 = call-poly "CoreLib.data 2 byte array.vi"("string"=w1083) -> ("byteArray out"=w1084:T1)  [unwired: 18 in]
            }
          }
          n517 = Unbundle By Name(w1077) -> ("code"=w1082:i32)
          n518 = Bundle By Name(cluster=w1073, "Data"=w1080, "Error #"=w1082, "Data Descriptor"="C:N") -> (w1081:T2)
        }
        frame "Configure" {
          # "This is just an example. On how to use this VI. The names of the selector should be identical to the name of the corresponding event. Inside the false case, place the method you want to call."
          n519 = Unbundle By Name(w1135) -> ("Data"=w1125:T1)
          n520 = call-poly "CoreLib.byte array 2 data.vi"("byteArray"=w1125) -> ("string"=w1126:string, "error out"=w1124:errorcluster)  [unwired: 16 in, 1 out]
          n521 = call "CoreLib.stringToStringArray.vi"("String"=w1126) -> ("Array"=w1123:string[])
          n522 = case shown="No Error" w1124 {
            tunnel: [w1140 w1147] -> w1132
            tunnel: w1138 -> [w1142 w1147]
            tunnel: w1137 -> [w1143 w1146]
            tunnel: [w1141 w1145] -> w1131
            tunnel: w1123 -> [w1139 _]
            tunnel: w1129 -> [_ w1144]
            frame No Error {
              n523 = call "DeviceBase.configure.vi"("i ref in"=w1142, "configureData"=w1139, "error in (no error)"=w1143) -> ("i ref out"=w1140:refnum<vi>, "error out"=w1141:errorcluster)  [unwired: 14 in, 1 out]
            }
            frame Error {
              n524 = call "CoreLib.set data type mismatch.vi"("error in (no error)"=w1146, "error source"=w1144) -> ("error out"=w1145:errorcluster)  [unwired: 17 in]
            }
          }
          n525 = call "BaseProcess.set event status.vi"("i ref in"=w1132, "EventStatus"=w1129, "error in (no error)"=w1131) -> ("i ref out"=w1128:refnum<vi>, "error out"=w1130:errorcluster)  [unwired: 14 in, 1 out]
          n526 = Unbundle By Name(w1130) -> ("source"=w1122:string)
          n527 = Unbundle By Name(w1130) -> ("code"=w1136:i32)
          n528 = call-poly "CoreLib.data 2 byte array.vi"("string"=w1122) -> ("byteArray out"=w1133:T1)  [unwired: 18 in]
          n529 = Bundle By Name(cluster=w1135, "Data"=w1133, "Error #"=w1136, "Data Descriptor"="C:N") -> (w1134:T2)
        }
        frame "DIMUpdate" {
          n530 = call "CAEObj.unfold trend data.vi"("i ref in"=w1149, "raw trend data"=w1158, "error in (no error)"=w1151) -> ("quality"=w1153:i32, "timeStamp"=w1155:dbl, "no link"=w1154:bool, "data"=w1148:i8[], "serviceName"=w1150:string, "error out"=w1152:errorcluster)  [unwired: 8 in, 3 out]
          n531 = case shown="No Error" w1152 {
            selector: w1152 -> [w1184 w2792]
            tunnel: [w1188 w2794] -> w1164
            tunnel: w1149 -> [w1182 w2794]
            tunnel: [w1189 w2793] -> w1163
            tunnel: w1156 -> [w1190 _]
            tunnel: w1155 -> [w1172 _]
            tunnel: w1154 -> [w1187 _]
            tunnel: w1153 -> [w1186 _]
            tunnel: w1148 -> [w1185 _]
            tunnel: w1150 -> [w1178 _]
            frame No Error {
              n532 = call "PSChannelBase.get i attribute.vi"("i ref in"=w1182, "error in (no error)"=w1184) -> ("i ref out"=w1181:refnum<vi>, "i attribute"=w1180:T14, "error out"=w1183:errorcluster)  [unwired: 15 in]
              n533 = Reverse String(1:w1178) -> (0:w1177:string)
              n534 = To Time Stamp(1:w1172) -> (0:w1171:timestamp)
              n535 = Unbundle By Name(w1180) -> ("physicalName"=w1179:string[])
              n536 = Match Pattern(string=w1177, regular expression="_") -> (before substring=w1174:string, after substring=w1175:string)  [unwired: 1 in, 2 out]
              n537 = Reverse String(1:w1175) -> (0:w1173:string)
              n538 = Reverse String(1:w1174) -> (0:w1169:string)
              n539 = Search 1D Array(1D array=w1179, element=w1173) -> (index of element=w1170:i32)  [unwired: 1 in]
              n540 = case "-1: Channel not found" shown="Default" w1170 {
                selector: w1170 -> [_ w1220]
                tunnel: w1181 -> [w1198 w1230]
                tunnel: w1190 -> [_ w1229]
                tunnel: [w1196 w1205] -> w1189
                tunnel: [w1198 w1206] -> w1188
                tunnel: w1187 -> [_ w1226]
                tunnel: w1186 -> [_ w1225]
                tunnel: w1185 -> [_ w1224]
                tunnel: w1183 -> [w1197 w1222]
                tunnel: w1171 -> [_ w1221]
                tunnel: w1169 -> [_ w1218]
                frame -1 {
                  n541 = call "CoreLib.my to LV error.vi"("ErrorTypes"=CoreDefs.error_type."element not found", "severityLevel"=CoreDefs.error_severity."warning") -> ("myErrorCluster"=w1193:errorcluster)  [unwired: 16 in, 1 out]
                  n542 = Bundle By Name(cluster=w1193, "source"="DIMUpdate") -> (w1192:errorcluster)
                  n543 = Select(t=w1197, s=w1197, f=w1192) -> (s? t:f=w1196:errorcluster)
                }
                frame Default {
                  n544 = call "CAEN_HVChannel.get data to modify.vi"("i ref in"=w1230, "ms timeout (10000)"=w1229, "error in (no error)"=w1222) -> ("i ref out"=w1228:refnum<vi>, "i attribute"=w1223:T9, "timed out"=w1219:bool, "error out"=w1227:errorcluster)  [unwired: 13 in]
                  n545 = case "timed out?" shown="False" w1219 {
                    tunnel: w1228 -> [w1252 w2791]
                    tunnel: w1227 -> [w1257 w2790]
                    tunnel: [w1276 w2790] -> w1216
                    tunnel: [w1275 w2791] -> w1217
                    tunnel: w1226 -> [w1274 _]
                    tunnel: w1225 -> [w1273 _]
                    tunnel: w1224 -> [w1272 _]
                    tunnel: w1223 -> [w1268 _]
                    tunnel: w1221 -> [w1265 _]
                    tunnel: w1220 -> [w1255 w2788]
                    tunnel: w1218 -> [w1264 _]
                    tunnel: [w1263 PSChannelBase.directionType."unknown" ("direction")] -> w1210
                    tunnel: [w1262 _] -> w1213
                    tunnel: [w1261 _] -> w1212
                    tunnel: [w1260 _] -> w1211
                    tunnel: [w1255 w2788] -> w1204
                    tunnel: [w1259 _] -> w1201
                    frame False {
                      n546 = Unbundle By Name(w1268) -> ("VoltageInRangeBand"=w1258:dbl, "Channel Array"=w1270:T10)
                      n547 = Index Array(array=w1270, index=w1255) -> (element=w1271:T11)
                      n548 = call "PSChannelBase.get channel status.vi"("i ref in"=w1252, "channelIndex"=w1255, "error in (no error)"=w1257) -> ("i ref out"=w1253:refnum<vi>, "status"=w1254:i32, "error out"=w1256:errorcluster)  [unwired: 14 in]
                      n549 = case "Attribute" shown="\"PDwn\"" w1264 {
                        tunnel: w1274 -> [w1286 w1315 w1346 w1367 w1388 w1409 w1440 w1461 w1490 w1523 w1562 w1583 w1604 w1622 w1642 w1660 w1678 w1698 w1716 w1734 w1754 w1772 w1794 w1827 w1866 w1887 w1912 w1945 w1984 w2005 w2026 w2047 w2078 w2099 w2128 w2181 w2202 w2233 w2254 w2275 w2296 w2327 w2348 w2369 w2390 w2421 w2442 w2463 w2484 w2515 w2536 w2557 w2578 w2609 w2630 w2660 w2710 w2749 w2770 _]
                        tunnel: w1273 -> [w1285 w1314 w1345 w1366 w1387 w1408 w1439 w1460 w1489 w1522 w1561 w1582 w1603 w1621 w1641 w1659 w1677 w1697 w1715 w1733 w1753 w1771 w1793 w1826 w1865 w1886 w1911 w1944 w1983 w2004 w2025 w2046 w2077 w2098 w2127 w2180 w2201 w2232 w2253 w2274 w2295 w2326 w2347 w2368 w2389 w2420 w2441 w2462 w2483 w2514 w2535 w2556 w2577 w2608 w2629 w2659 w2709 w2748 w2769 _]
                        tunnel: w1272 -> [w1284 w1313 w1344 w1365 w1386 w1407 w1438 w1459 w1488 w1521 w1560 w1581 w1602 w1620 w1640 w1658 w1676 w1696 w1714 w1732 w1752 w1770 w1792 w1825 w1864 w1885 w1910 w1943 w1982 w2003 w2024 w2045 w2076 w2097 w2126 w2179 w2200 w2231 w2252 w2273 w2294 w2325 w2346 w2367 w2388 w2419 w2440 w2461 w2482 w2513 w2534 w2555 w2576 w2607 w2628 w2658 w2708 w2747 w2768 _]
                        tunnel: w1271 -> [w1283 w1312 w1343 w1364 w1385 w1406 w1437 w1458 w1487 w1520 w1559 w1580 w1601 w1619 w1639 w1657 w1675 w1695 w1713 w1731 w1751 w1769 w1791 w1824 w1863 w1884 w1909 w1942 w1981 w2002 w2023 w2044 w2075 w2096 w2125 w2178 w2199 w2230 w2251 w2272 w2293 w2324 w2345 w2366 w2387 w2418 w2439 w2460 w2481 w2512 w2533 w2554 w2575 w2606 w2627 w2657 w2707 w2746 w2767 w2787]
                        tunnel: [w1282 w1311 w1342 w1363 w1384 w1405 w1436 w1457 w1486 w1519 w1558 w1579 w1600 w1618 w1638 w1656 w1674 w1694 w1712 w1730 w1750 w1768 w1790 w1823 w1862 w1883 w1908 w1941 w1980 w2001 w2022 w2043 w2074 w2095 w2124 w2177 w2198 w2229 w2250 w2271 w2292 w2323 w2344 w2365 w2386 w2417 w2438 w2459 w2480 w2511 w2532 w2553 w2574 w2605 w2626 w2656 w2706 w2745 w2766 w2787] -> w1269
                        tunnel: w1265 -> [w1281 w1310 w1341 w1362 w1383 w1404 w1435 w1456 w1485 w1518 w1557 w1578 w1599 w1617 w1637 w1655 w1673 w1693 w1711 w1729 w1749 w1767 w1789 w1822 w1861 w1882 w1907 w1940 w1979 w2000 w2021 w2042 w2073 w2094 w2123 w2176 w2197 w2228 w2249 w2270 w2291 w2322 w2343 w2364 w2385 w2416 w2437 w2458 w2479 w2510 w2531 w2552 w2573 w2604 w2625 w2655 w2705 w2744 w2765 _]
                        tunnel: [w1280 _ _ _ _ _ _ _ w1484 w1517 _ _ _ _ _ _ _ _ _ _ _ _ w1788 w1821 _ _ w1906 w1939 _ _ _ _ _ _ w2122 _ _ _ _ _ _ _ _ _ _ _ _ _ _ _ _ _ _ _ _ w2654 w2704 _ _ PSChannelBase.directionType."unknown" ("direction")] -> w1263
                        tunnel: [w1278 _ _ _ _ _ _ _ w1483 w1515 _ _ _ _ _ _ _ _ _ _ _ _ w1786 w1819 _ _ w1904 w1937 _ _ _ _ _ _ w2121 _ _ _ _ _ _ _ _ _ _ _ _ _ _ _ _ _ _ _ _ w2653 w2702 _ _ _] -> w1262
                        tunnel: [w1279 _ _ _ _ _ _ _ w1482 w1516 _ _ _ _ _ _ _ _ _ _ _ _ w1787 w1820 _ _ w1905 w1938 _ _ _ _ _ _ w2120 _ _ _ _ _ _ _ _ _ _ _ _ _ _ _ _ _ _ _ _ w2652 w2703 _ _ _] -> w1261
                        tunnel: [w1277 _ _ _ _ _ _ _ w1481 w1514 _ _ _ _ _ _ _ _ _ _ _ _ w1785 w1818 _ _ w1903 w1936 _ _ _ _ _ _ w2119 _ _ _ _ _ _ _ _ _ _ _ _ _ _ _ _ _ _ _ _ w2651 w2701 _ _ _] -> w1260
                        tunnel: [_ _ _ _ _ _ _ _ _ _ _ _ _ _ _ _ _ _ _ _ _ _ _ _ _ _ _ _ _ _ _ _ _ _ _ _ _ _ _ _ _ _ _ _ _ _ _ _ _ _ _ _ _ _ _ w2646 _ _ _ _] -> w1259
                        tunnel: w1253 -> [_ _ _ _ _ _ _ _ w1480 _ _ _ _ _ _ _ _ _ _ _ _ _ _ _ _ _ _ _ _ _ _ _ _ _ w2118 _ _ _ _ _ _ _ _ _ _ _ _ _ _ _ _ _ _ _ _ w2650 _ _ _ _]
                        tunnel: w1255 -> [_ _ _ _ _ _ _ _ w1479 _ _ _ _ _ _ _ _ _ _ _ _ _ _ _ _ _ _ _ _ _ _ _ _ _ w2117 _ _ _ _ _ _ _ _ _ _ _ _ _ _ _ _ _ _ _ _ w2649 _ _ _ _]
                        tunnel: w1258 -> [_ _ _ _ _ _ _ _ w1478 _ _ _ _ _ _ _ _ _ _ _ _ _ _ _ _ _ _ _ _ _ _ _ _ _ w2116 _ _ _ _ _ _ _ _ _ _ _ _ _ _ _ _ _ _ _ _ w2648 _ _ _ _]
                        tunnel: w1254 -> [_ _ _ _ _ _ _ _ w1477 _ _ _ _ _ _ _ _ _ _ _ _ _ _ _ _ _ _ _ _ _ _ _ _ _ w2115 _ _ _ _ _ _ _ _ _ _ _ _ _ _ _ _ _ _ _ _ w2647 _ _ _ _]
                        frame "I0Set" {
                          n550 = case "no link?" shown="False" w1286 {
                            selector: w1286 -> [w1294 w1305]
                            tunnel: [w1296 w1309] -> w1282
                            tunnel: w1284 -> [_ w1308]
                            tunnel: w1283 -> [w1288 w1304]
                            tunnel: w1285 -> [w1293 w1301]
                            tunnel: w1281 -> [w1295 w1306]
                            tunnel: [PSChannelBase.directionType."update actual value" ("direction") PSChannelBase.directionType."update actual value" ("direction")] -> w1280
                            tunnel: [PSChannelBase.serviceType."tripCurrent" ("service") PSChannelBase.serviceType."tripCurrent" ("service")] -> w1279
                            tunnel: [w1290 w1298] -> w1278
                            tunnel: [UtilityLib.valueStatus."no info available" ("quality") _] -> w1277
                            frame True {
                              n551 = Unbundle By Name(w1288) -> ("I0Set.I0Set.I0Set"=w1287:dbl)
                              n552 = Bundle By Name(cluster=w1288, "I0Set.I0Set.DIM Status.quality"=w1293, "I0Set.I0Set.DIM Status.Time Stamp"=w1295, "I0Set.I0Set.DIM Status.no link"=w1294) -> (w1296:T11)
                              n553 = Type Cast(x=w1287) -> (*(type *) &x=w1290:string)  [unwired: 1 in]
                            }
                            frame False {
                              n554 = Type Cast(type=0.0, x=w1308) -> (*(type *) &x=w1307:dbl)
                              n555 = Unbundle By Name(w1304) -> ("I0Set.I0Set#Multiplier"=w1302:dbl)
                              n556 = Multiply(x=w1302, y=w1307) -> (x*y=w1297:dbl)
                              n557 = Bundle By Name(cluster=w1304, "I0Set.I0Set.DIM Status.quality"=w1301, "I0Set.I0Set.DIM Status.Time Stamp"=w1306, "I0Set.I0Set.I0Set"=w1297, "I0Set.I0Set.DIM Status.no link"=w1305) -> (w1309:T11)
                              n558 = Type Cast(x=w1297) -> (*(type *) &x=w1298:string)  [unwired: 1 in]
                            }
                          }
                        }
                        frame "I0Set#EU" {
                          n559 = case "no link?" shown="False" w1315 {
                            selector: w1315 -> [w1316 w1336]
                            tunnel: [w1320 w1340] -> w1311
                            tunnel: w1313 -> [_ w1339]
                            tunnel: w1312 -> [w1319 w1335]
                            tunnel: w1314 -> [w1318 w1338]
                            tunnel: w1310 -> [w1317 w1337]
                            frame True {
                              n560 = Bundle By Name(cluster=w1319, "I0Set.I0Set#EU.DIM Status.quality"=w1318, "I0Set.I0Set#EU.DIM Status.Time Stamp"=w1317, "I0Set.I0Set#EU.DIM Status.no link"=w1316) -> (w1320:T11)
                            }
                            frame False {
                              n561 = Type Cast(x=w1339) -> (*(type *) &x=w1334:string)  [unwired: 1 in]
                              n562 = Unbundle By Name(w1335) -> ("I0Set.I0Set.I0Set"=w1328:dbl, "I0Set.I0Set#HighEU.I0Set#HighEU"=w1327:dbl, "I0Set.I0Set#LowEU.I0Set#LowEU"=w1326:dbl, "I0Set.I0Set#Multiplier"=w1325:dbl)
                              n563 = call "CAEN_HVSystem.EUString2UnitMultilier.vi"("EU String"=w1334) -> ("Multiplier"=w1324:dbl, "Unit"=w1333:string)  [unwired: 2 in, 1 out]
                              n564 = Build Array(w1328, w1327, w1326) -> (w1330:dbl[])
                              n565 = Divide(x=w1330, y=w1325) -> (x/y=w1329:dbl[])
                              n566 = Multiply(x=w1329, y=w1324) -> (x*y=w1331:dbl[])
                              n567 = Index Array(array=w1331, index #1=0 ("index")) -> (element #1=w1323:dbl, element #2=w1322:dbl, element #3=w1321:dbl)  [unwired: 2 in]
                              n568 = Bundle By Name(cluster=w1335, "I0Set.I0Set.I0Set"=w1323, "I0Set.I0Set#HighEU.I0Set#HighEU"=w1322, "I0Set.I0Set#LowEU.I0Set#LowEU"=w1321, "I0Set.I0Set#Multiplier"=w1324, "I0Set.I0Set#EU.DIM Status.quality"=w1338, "I0Set.I0Set#EU.DIM Status.Time Stamp"=w1337, "I0Set.I0Set#EU.I0Set#EU"=w1333, "I0Set.I0Set#EU.DIM Status.no link"=w1336) -> (w1340:T11)
                            }
                          }
                        }
                        frame "I0Set#HighEU" {
                          n569 = case "no link?" shown="False" w1346 {
                            selector: w1346 -> [w1347 w1356]
                            tunnel: [w1351 w1361] -> w1342
                            tunnel: w1344 -> [_ w1360]
                            tunnel: w1343 -> [w1350 w1355]
                            tunnel: w1345 -> [w1349 w1358]
                            tunnel: w1341 -> [w1348 w1357]
                            frame True {
                              n570 = Bundle By Name(cluster=w1350, "I0Set.I0Set#HighEU.DIM Status.quality"=w1349, "I0Set.I0Set#HighEU.DIM Status.Time Stamp"=w1348, "I0Set.I0Set#HighEU.DIM Status.no link"=w1347) -> (w1351:T11)
                            }
                            frame False {
                              n571 = Type Cast(type=0.0, x=w1360) -> (*(type *) &x=w1359:dbl)
                              n572 = Unbundle By Name(w1355) -> ("I0Set.I0Set#Multiplier"=w1352:dbl)
                              n573 = Multiply(x=w1352, y=w1359) -> (x*y=w1353:dbl)
                              n574 = Bundle By Name(cluster=w1355, "I0Set.I0Set#HighEU.DIM Status.quality"=w1358, "I0Set.I0Set#HighEU.DIM Status.Time Stamp"=w1357, "I0Set.I0Set#HighEU.I0Set#HighEU"=w1353, "I0Set.I0Set#HighEU.DIM Status.no link"=w1356) -> (w1361:T11)
                            }
                          }
                        }
                        frame "I0Set#LowEU" {
                          n575 = case "no link?" shown="False" w1367 {
                            selector: w1367 -> [w1368 w1377]
                            tunnel: [w1372 w1382] -> w1363
                            tunnel: w1365 -> [_ w1381]
                            tunnel: w1364 -> [w1371 w1376]
                            tunnel: w1366 -> [w1370 w1379]
                            tunnel: w1362 -> [w1369 w1378]
                            frame True {
                              n576 = Bundle By Name(cluster=w1371, "I0Set.I0Set#LowEU.DIM Status.quality"=w1370, "I0Set.I0Set#LowEU.DIM Status.Time Stamp"=w1369, "I0Set.I0Set#LowEU.DIM Status.no link"=w1368) -> (w1372:T11)
                            }
                            frame False {
                              n577 = Type Cast(type=0.0, x=w1381) -> (*(type *) &x=w1380:dbl)
                              n578 = Unbundle By Name(w1376) -> ("I0Set.I0Set#Multiplier"=w1373:dbl)
                              n579 = Multiply(x=w1373, y=w1380) -> (x*y=w1374:dbl)
                              n580 = Bundle By Name(cluster=w1376, "I0Set.I0Set#LowEU.DIM Status.quality"=w1379, "I0Set.I0Set#LowEU.DIM Status.Time Stamp"=w1378, "I0Set.I0Set#LowEU.I0Set#LowEU"=w1374, "I0Set.I0Set#LowEU.DIM Status.no link"=w1377) -> (w1382:T11)
                            }
                          }
                        }
                        frame "I1Set" {
                          n581 = case "no link?" shown="False" w1388 {
                            selector: w1388 -> [w1391 w1399]
                            tunnel: [w1393 w1403] -> w1384
                            tunnel: w1386 -> [_ w1402]
                            tunnel: w1385 -> [w1390 w1398]
                            tunnel: w1387 -> [w1389 w1394]
                            tunnel: w1383 -> [w1392 w1400]
                            frame True {
                              n582 = Bundle By Name(cluster=w1390, "I1Set.I1Set.DIM Status.quality"=w1389, "I1Set.I1Set.DIM Status.Time Stamp"=w1392, "I1Set.I1Set.DIM Status.no link"=w1391) -> (w1393:T11)
                            }
                            frame False {
                              n583 = Type Cast(type=0.0, x=w1402) -> (*(type *) &x=w1401:dbl)
                              n584 = Unbundle By Name(w1398) -> ("I1Set.I1Set#Multiplier"=w1396:dbl)
                              n585 = Multiply(x=w1396, y=w1401) -> (x*y=w1395:dbl)
                              n586 = Bundle By Name(cluster=w1398, "I1Set.I1Set.DIM Status.quality"=w1394, "I1Set.I1Set.DIM Status.Time Stamp"=w1400, "I1Set.I1Set.I1Set"=w1395, "I1Set.I1Set.DIM Status.no link"=w1399) -> (w1403:T11)
                            }
                          }
                        }
                        frame "I1Set#EU" {
                          n587 = case "no link?" shown="False" w1409 {
                            selector: w1409 -> [w1410 w1430]
                            tunnel: [w1414 w1434] -> w1405
                            tunnel: w1407 -> [_ w1433]
                            tunnel: w1406 -> [w1413 w1429]
                            tunnel: w1408 -> [w1412 w1432]
                            tunnel: w1404 -> [w1411 w1431]
                            frame True {
                              n588 = Bundle By Name(cluster=w1413, "I1Set.I1Set#EU.DIM Status.quality"=w1412, "I1Set.I1Set#EU.DIM Status.Time Stamp"=w1411, "I1Set.I1Set#EU.DIM Status.no link"=w1410) -> (w1414:T11)
                            }
                            frame False {
                              n589 = Type Cast(x=w1433) -> (*(type *) &x=w1428:string)  [unwired: 1 in]
                              n590 = Unbundle By Name(w1429) -> ("I1Set.I1Set.I1Set"=w1422:dbl, "I1Set.I1Set#HighEU.I1Set#HighEU"=w1421:dbl, "I1Set.I1Set#LowEU.I1Set#LowEU"=w1420:dbl, "I1Set.I1Set#Multiplier"=w1419:dbl)
                              n591 = call "CAEN_HVSystem.EUString2UnitMultilier.vi"("EU String"=w1428) -> ("Multiplier"=w1418:dbl, "Unit"=w1427:string)  [unwired: 2 in, 1 out]
                              n592 = Build Array(w1422, w1421, w1420) -> (w1424:dbl[])
                              n593 = Divide(x=w1424, y=w1419) -> (x/y=w1423:dbl[])
                              n594 = Multiply(x=w1423, y=w1418) -> (x*y=w1425:dbl[])
                              n595 = Index Array(array=w1425, index #1=0 ("index")) -> (element #1=w1417:dbl, element #2=w1416:dbl, element #3=w1415:dbl)  [unwired: 2 in]
                              n596 = Bundle By Name(cluster=w1429, "I1Set.I1Set.I1Set"=w1417, "I1Set.I1Set#HighEU.I1Set#HighEU"=w1416, "I1Set.I1Set#LowEU.I1Set#LowEU"=w1415, "I1Set.I1Set#Multiplier"=w1418, "I1Set.I1Set#EU.DIM Status.quality"=w1432, "I1Set.I1Set#EU.DIM Status.Time Stamp"=w1431, "I1Set.I1Set#EU.I1Set#EU"=w1427, "I1Set.I1Set#EU.DIM Status.no link"=w1430) -> (w1434:T11)
                            }
                          }
                        }
                        frame "I1Set#HighEU" {
                          n597 = case "no link?" shown="False" w1440 {
                            selector: w1440 -> [w1441 w1450]
                            tunnel: [w1445 w1455] -> w1436
                            tunnel: w1438 -> [_ w1454]
                            tunnel: w1437 -> [w1444 w1449]
                            tunnel: w1439 -> [w1443 w1452]
                            tunnel: w1435 -> [w1442 w1451]
                            frame True {
                              n598 = Bundle By Name(cluster=w1444, "I1Set.I1Set#HighEU.DIM Status.quality"=w1443, "I1Set.I1Set#HighEU.DIM Status.Time Stamp"=w1442, "I1Set.I1Set#HighEU.DIM Status.no link"=w1441) -> (w1445:T11)
                            }
                            frame False {
                              n599 = Type Cast(type=0.0, x=w1454) -> (*(type *) &x=w1453:dbl)
                              n600 = Unbundle By Name(w1449) -> ("I1Set.I1Set#Multiplier"=w1446:dbl)
                              n601 = Multiply(x=w1446, y=w1453) -> (x*y=w1447:dbl)
                              n602 = Bundle By Name(cluster=w1449, "I1Set.I1Set#HighEU.DIM Status.quality"=w1452, "I1Set.I1Set#HighEU.DIM Status.Time Stamp"=w1451, "I1Set.I1Set#HighEU.I1Set#HighEU"=w1447, "I1Set.I1Set#HighEU.DIM Status.no link"=w1450) -> (w1455:T11)
                            }
                          }
                        }
                        frame "I1Set#LowEU" {
                          n603 = case "no link?" shown="False" w1461 {
                            selector: w1461 -> [w1462 w1471]
                            tunnel: [w1466 w1476] -> w1457
                            tunnel: w1459 -> [_ w1475]
                            tunnel: w1458 -> [w1465 w1470]
                            tunnel: w1460 -> [w1464 w1473]
                            tunnel: w1456 -> [w1463 w1472]
                            frame True {
                              n604 = Bundle By Name(cluster=w1465, "I1Set.I1Set#LowEU.DIM Status.quality"=w1464, "I1Set.I1Set#LowEU.DIM Status.Time Stamp"=w1463, "I1Set.I1Set#LowEU.DIM Status.no link"=w1462) -> (w1466:T11)
                            }
                            frame False {
                              n605 = Type Cast(type=0.0, x=w1475) -> (*(type *) &x=w1474:dbl)
                              n606 = Unbundle By Name(w1470) -> ("I1Set.I1Set#Multiplier"=w1467:dbl)
                              n607 = Multiply(x=w1467, y=w1474) -> (x*y=w1468:dbl)
                              n608 = Bundle By Name(cluster=w1470, "I1Set.I1Set#LowEU.DIM Status.quality"=w1473, "I1Set.I1Set#LowEU.DIM Status.Time Stamp"=w1472, "I1Set.I1Set#LowEU.I1Set#LowEU"=w1468, "I1Set.I1Set#LowEU.DIM Status.no link"=w1471) -> (w1476:T11)
                            }
                          }
                        }
                        frame "IMon" {
                          n609 = case "no link?" shown="False" w1490 {
                            selector: w1490 -> [w1498 w1509]
                            tunnel: [w1500 w1513] -> w1486
                            tunnel: w1488 -> [_ w1512]
                            tunnel: w1487 -> [w1497 w1508]
                            tunnel: w1489 -> [w1494 w1502]
                            tunnel: w1485 -> [w1499 w1510]
                            tunnel: [PSChannelBase.directionType."update actual value" ("direction") PSChannelBase.directionType."update actual value" ("direction")] -> w1484
                            tunnel: [w1496 w1504] -> w1483
                            tunnel: [PSChannelBase.serviceType."current" ("service") PSChannelBase.serviceType."current" ("service")] -> w1482
                            tunnel: [UtilityLib.valueStatus."no info available" ("quality") w1502] -> w1481
                            tunnel: w1480 -> [_ _]
                            tunnel: w1479 -> [_ _]
                            tunnel: w1478 -> [_ _]
                            tunnel: w1477 -> [_ _]
                            frame True {
                              n610 = Unbundle By Name(w1497) -> ("IMon.IMon.IMon"=w1495:dbl)
                              n611 = Bundle By Name(cluster=w1497, "IMon.IMon.DIM Status.quality"=w1494, "IMon.IMon.DIM Status.Time Stamp"=w1499, "IMon.IMon.DIM Status.no link"=w1498) -> (w1500:T11)
                              n612 = Type Cast(x=w1495) -> (*(type *) &x=w1496:string)  [unwired: 1 in]
                            }
                            frame False {
                              n613 = Type Cast(type=0.0, x=w1512) -> (*(type *) &x=w1511:dbl)
                              n614 = Unbundle By Name(w1508) -> ("IMon.IMon#Multiplier"=w1506:dbl)
                              n615 = Multiply(x=w1506, y=w1511) -> (x*y=w1501:dbl)
                              n616 = Bundle By Name(cluster=w1508, "IMon.IMon.DIM Status.quality"=w1502, "IMon.IMon.DIM Status.Time Stamp"=w1510, "IMon.IMon.IMon"=w1501, "IMon.IMon.DIM Status.no link"=w1509) -> (w1513:T11)
                              n617 = Type Cast(x=w1501) -> (*(type *) &x=w1504:string)  [unwired: 1 in]
                            }
                          }
                        }
                        frame "IMon#EU" {
                          n618 = case "no link?" shown="False" w1523 {
                            selector: w1523 -> [w1530 w1553]
                            tunnel: [w1533 w1556] -> w1519
                            tunnel: w1521 -> [_ w1555]
                            tunnel: w1520 -> [w1526 w1552]
                            tunnel: w1522 -> [w1532 w1534]
                            tunnel: w1518 -> [w1531 w1554]
                            tunnel: [PSChannelBase.directionType."update actual value" ("direction") PSChannelBase.directionType."update actual value" ("direction")] -> w1517
                            tunnel: [PSChannelBase.serviceType."current" ("service") PSChannelBase.serviceType."current" ("service")] -> w1516
                            tunnel: [w1524 w1535] -> w1515
                            tunnel: [UtilityLib.valueStatus."warning" ("quality") w1534] -> w1514
                            frame True {
                              n619 = Unbundle By Name(w1526) -> ("VMon.VMon.VMon"=w1525:dbl)
                              n620 = Type Cast(x=w1525) -> (*(type *) &x=w1524:string)  [unwired: 1 in]
                              n621 = Bundle By Name(cluster=w1526, "IMon.IMon#EU.DIM Status.quality"=w1532, "IMon.IMon#EU.DIM Status.Time Stamp"=w1531, "IMon.IMon#EU.DIM Status.no link"=w1530) -> (w1533:T11)
                            }
                            frame False {
                              n622 = Type Cast(x=w1555) -> (*(type *) &x=w1551:string)  [unwired: 1 in]
                              n623 = Unbundle By Name(w1552) -> ("IMon.IMon.IMon"=w1545:dbl, "IMon.IMon#HighEU.IMon#HighEU"=w1544:dbl, "IMon.IMon#LowEU.IMon#LowEU"=w1543:dbl, "IMon.IMon#Multiplier"=w1542:dbl)
                              n624 = call "CAEN_HVSystem.EUString2UnitMultilier.vi"("EU String"=w1551) -> ("Multiplier"=w1541:dbl, "Unit"=w1550:string)  [unwired: 2 in, 1 out]
                              n625 = Build Array(w1545, w1544, w1543) -> (w1547:dbl[])
                              n626 = Divide(x=w1547, y=w1542) -> (x/y=w1546:dbl[])
                              n627 = Multiply(x=w1546, y=w1541) -> (x*y=w1548:dbl[])
                              n628 = Index Array(array=w1548, index #1=0 ("index")) -> (element #1=w1536:dbl, element #2=w1540:dbl, element #3=w1539:dbl)  [unwired: 2 in]
                              n629 = Bundle By Name(cluster=w1552, "IMon.IMon.IMon"=w1536, "IMon.IMon#HighEU.IMon#HighEU"=w1540, "IMon.IMon#LowEU.IMon#LowEU"=w1539, "IMon.IMon#Multiplier"=w1541, "IMon.IMon#EU.DIM Status.quality"=w1534, "IMon.IMon#EU.DIM Status.Time Stamp"=w1554, "IMon.IMon#EU.IMon#EU"=w1550, "IMon.IMon#EU.DIM Status.no link"=w1553) -> (w1556:T11)
                              n630 = Type Cast(x=w1536) -> (*(type *) &x=w1535:string)  [unwired: 1 in]
                            }
                          }
                        }
                        frame "IMon#HighEU" {
                          n631 = case "no link?" shown="False" w1562 {
                            selector: w1562 -> [w1563 w1572]
                            tunnel: [w1567 w1577] -> w1558
                            tunnel: w1560 -> [_ w1576]
                            tunnel: w1559 -> [w1566 w1571]
                            tunnel: w1561 -> [w1565 w1574]
                            tunnel: w1557 -> [w1564 w1573]
                            frame True {
                              n632 = Bundle By Name(cluster=w1566, "IMon.IMon#HighEU.DIM Status.quality"=w1565, "IMon.IMon#HighEU.DIM Status.Time Stamp"=w1564, "IMon.IMon#HighEU.DIM Status.no link"=w1563) -> (w1567:T11)
                            }
                            frame False {
                              n633 = Type Cast(type=0.0, x=w1576) -> (*(type *) &x=w1575:dbl)
                              n634 = Unbundle By Name(w1571) -> ("IMon.IMon#Multiplier"=w1568:dbl)
                              n635 = Multiply(x=w1568, y=w1575) -> (x*y=w1569:dbl)
                              n636 = Bundle By Name(cluster=w1571, "IMon.IMon#HighEU.DIM Status.quality"=w1574, "IMon.IMon#HighEU.DIM Status.Time Stamp"=w1573, "IMon.IMon#HighEU.IMon#HighEU"=w1569, "IMon.IMon#HighEU.DIM Status.no link"=w1572) -> (w1577:T11)
                            }
                          }
                        }
                        frame "IMon#LowEU" {
                          n637 = case "no link?" shown="False" w1583 {
                            selector: w1583 -> [w1584 w1593]
                            tunnel: [w1588 w1598] -> w1579
                            tunnel: w1581 -> [_ w1597]
                            tunnel: w1580 -> [w1587 w1592]
                            tunnel: w1582 -> [w1586 w1595]
                            tunnel: w1578 -> [w1585 w1594]
                            frame True {
                              n638 = Bundle By Name(cluster=w1587, "IMon.IMon#LowEU.DIM Status.quality"=w1586, "IMon.IMon#LowEU.DIM Status.Time Stamp"=w1585, "IMon.IMon#LowEU.DIM Status.no link"=w1584) -> (w1588:T11)
                            }
                            frame False {
                              n639 = Type Cast(type=0.0, x=w1597) -> (*(type *) &x=w1596:dbl)
                              n640 = Unbundle By Name(w1592) -> ("IMon.IMon#Multiplier"=w1589:dbl)
                              n641 = Multiply(x=w1589, y=w1596) -> (x*y=w1590:dbl)
                              n642 = Bundle By Name(cluster=w1592, "IMon.IMon#LowEU.DIM Status.quality"=w1595, "IMon.IMon#LowEU.DIM Status.Time Stamp"=w1594, "IMon.IMon#LowEU.IMon#LowEU"=w1590, "IMon.IMon#LowEU.DIM Status.no link"=w1593) -> (w1598:T11)
                            }
                          }
                        }
                        frame "Name" {
                          n643 = case "no link?" shown="True" w1604 {
                            selector: w1604 -> [w1605 w1610]
                            tunnel: [w1609 w1616] -> w1600
                            tunnel: w1602 -> [_ w1615]
                            tunnel: w1601 -> [w1608 w1614]
                            tunnel: w1603 -> [w1607 w1612]
                            tunnel: w1599 -> [w1606 w1611]
                            frame True {
                              n644 = Bundle By Name(cluster=w1608, "Name.DIM Status.quality"=w1607, "Name.DIM Status.Time Stamp"=w1606, "Name.DIM Status.no link"=w1605) -> (w1609:T11)
                            }
                            frame False {
                              n645 = Type Cast(x=w1615) -> (*(type *) &x=w1613:string)  [unwired: 1 in]
                              n646 = Bundle By Name(cluster=w1614, "Name.DIM Status.quality"=w1612, "Name.DIM Status.Time Stamp"=w1611, "Name.Name"=w1613, "Name.DIM Status.no link"=w1610) -> (w1616:T11)
                            }
                          }
                        }
                        frame "PDwn" {
                          n647 = case "no link?" shown="False" w1622 {
                            selector: w1622 -> [w1625 w1632]
                            tunnel: [w1631 w1636] -> w1618
                            tunnel: w1620 -> [w1630 _]
                            tunnel: w1619 -> [w1629 w1635]
                            tunnel: w1621 -> [w1627 w1634]
                            tunnel: w1617 -> [w1626 w1633]
                            frame False {
                              n648 = Type Cast(type=i16 0, x=w1630) -> (*(type *) &x=w1628:i16)
                              n649 = Not Equal To 0?(x=w1628) -> (x != 0?=w1624:bool)
                              n650 = Bundle By Name(cluster=w1629, "PDwn.PDwn.DIM Status.quality"=w1627, "PDwn.PDwn.DIM Status.Time Stamp"=w1626, "PDwn.PDwn.PDwn"=w1624, "PDwn.PDwn.DIM Status.no link"=w1625) -> (w1631:T11)
                            }
                            frame True {
                              n651 = Bundle By Name(cluster=w1635, "PDwn.PDwn.DIM Status.quality"=w1634, "PDwn.PDwn.DIM Status.Time Stamp"=w1633, "PDwn.PDwn.DIM Status.no link"=w1632) -> (w1636:T11)
                            }
                          }
                        }
                        frame "PDwn#CoClose" {
                          n652 = case "no link?" shown="True" w1642 {
                            selector: w1642 -> [w1643 w1650]
                            tunnel: [w1649 w1654] -> w1638
                            tunnel: w1640 -> [w1648 _]
                            tunnel: w1639 -> [w1647 w1653]
                            tunnel: w1641 -> [w1645 w1652]
                            tunnel: w1637 -> [w1644 w1651]
                            frame False {
                              n653 = Type Cast(x=w1648) -> (*(type *) &x=w1646:string)  [unwired: 1 in]
                              n654 = Bundle By Name(cluster=w1647, "PDwn.PDwn#CoClose.DIM Status.quality"=w1645, "PDwn.PDwn#CoClose.DIM Status.Time Stamp"=w1644, "PDwn.PDwn#CoClose.PDwn#CoClose"=w1646, "PDwn.PDwn#CoClose.DIM Status.no link"=w1643) -> (w1649:T11)
                            }
                            frame True {
                              n655 = Bundle By Name(cluster=w1653, "PDwn.PDwn#CoClose.DIM Status.quality"=w1652, "PDwn.PDwn#CoClose.DIM Status.Time Stamp"=w1651, "PDwn.PDwn#CoClose.DIM Status.no link"=w1650) -> (w1654:T11)
                            }
                          }
                        }
                        frame "PDwn#CoOpen" {
                          n656 = case "no link?" shown="False" w1660 {
                            selector: w1660 -> [w1661 w1668]
                            tunnel: [w1667 w1672] -> w1656
                            tunnel: w1658 -> [w1666 _]
                            tunnel: w1657 -> [w1665 w1671]
                            tunnel: w1659 -> [w1663 w1670]
                            tunnel: w1655 -> [w1662 w1669]
                            frame False {
                              n657 = Type Cast(x=w1666) -> (*(type *) &x=w1664:string)  [unwired: 1 in]
                              n658 = Bundle By Name(cluster=w1665, "PDwn.PDwn#CoOpen.DIM Status.quality"=w1663, "PDwn.PDwn#CoOpen.DIM Status.Time Stamp"=w1662, "PDwn.PDwn#CoOpen.PDwn#CoOpen"=w1664, "PDwn.PDwn#CoOpen.DIM Status.no link"=w1661) -> (w1667:T11)
                            }
                            frame True {
                              n659 = Bundle By Name(cluster=w1671, "PDwn.PDwn#CoOpen.DIM Status.quality"=w1670, "PDwn.PDwn#CoOpen.DIM Status.Time Stamp"=w1669, "PDwn.PDwn#CoOpen.DIM Status.no link"=w1668) -> (w1672:T11)
                            }
                          }
                        }
                        frame "POn" {
                          n660 = case "no link?" shown="False" w1678 {
                            selector: w1678 -> [w1681 w1688]
                            tunnel: [w1687 w1692] -> w1674
                            tunnel: w1676 -> [w1686 _]
                            tunnel: w1675 -> [w1685 w1691]
                            tunnel: w1677 -> [w1683 w1690]
                            tunnel: w1673 -> [w1682 w1689]
                            frame False {
                              n661 = Type Cast(type=i16 0, x=w1686) -> (*(type *) &x=w1684:i16)
                              n662 = Not Equal To 0?(x=w1684) -> (x != 0?=w1680:bool)
                              n663 = Bundle By Name(cluster=w1685, "POn.POn.DIM Status.quality"=w1683, "POn.POn.DIM Status.Time Stamp"=w1682, "POn.POn.POn"=w1680, "POn.POn.DIM Status.no link"=w1681) -> (w1687:T11)
                            }
                            frame True {
                              n664 = Bundle By Name(cluster=w1691, "POn.POn.DIM Status.quality"=w1690, "POn.POn.DIM Status.Time Stamp"=w1689, "POn.POn.DIM Status.no link"=w1688) -> (w1692:T11)
                            }
                          }
                        }
                        frame "POn#CoClose" {
                          n665 = case "no link?" shown="False" w1698 {
                            selector: w1698 -> [w1699 w1706]
                            tunnel: [w1705 w1710] -> w1694
                            tunnel: w1696 -> [w1704 _]
                            tunnel: w1695 -> [w1703 w1709]
                            tunnel: w1697 -> [w1701 w1708]
                            tunnel: w1693 -> [w1700 w1707]
                            frame False {
                              n666 = Type Cast(x=w1704) -> (*(type *) &x=w1702:string)  [unwired: 1 in]
                              n667 = Bundle By Name(cluster=w1703, "POn.POn#CoClose.DIM Status.quality"=w1701, "POn.POn#CoClose.DIM Status.Time Stamp"=w1700, "POn.POn#CoClose.POn#CoClose"=w1702, "POn.POn#CoClose.DIM Status.no link"=w1699) -> (w1705:T11)
                            }
                            frame True {
                              n668 = Bundle By Name(cluster=w1709, "POn.POn#CoClose.DIM Status.quality"=w1708, "POn.POn#CoClose.DIM Status.Time Stamp"=w1707, "POn.POn#CoClose.DIM Status.no link"=w1706) -> (w1710:T11)
                            }
                          }
                        }
                        frame "POn#CoOpen" {
                          n669 = case "no link?" shown="False" w1716 {
                            selector: w1716 -> [w1717 w1724]
                            tunnel: [w1723 w1728] -> w1712
                            tunnel: w1714 -> [w1722 _]
                            tunnel: w1713 -> [w1721 w1727]
                            tunnel: w1715 -> [w1719 w1726]
                            tunnel: w1711 -> [w1718 w1725]
                            frame False {
                              n670 = Type Cast(x=w1722) -> (*(type *) &x=w1720:string)  [unwired: 1 in]
                              n671 = Bundle By Name(cluster=w1721, "POn.POn#CoOpen.DIM Status.quality"=w1719, "POn.POn#CoOpen.DIM Status.Time Stamp"=w1718, "POn.POn#CoOpen.POn#CoOpen"=w1720, "POn.POn#CoOpen.DIM Status.no link"=w1717) -> (w1723:T11)
                            }
                            frame True {
                              n672 = Bundle By Name(cluster=w1727, "POn.POn#CoOpen.DIM Status.quality"=w1726, "POn.POn#CoOpen.DIM Status.Time Stamp"=w1725, "POn.POn#CoOpen.DIM Status.no link"=w1724) -> (w1728:T11)
                            }
                          }
                        }
                        frame "Pw" {
                          n673 = case "no link?" shown="False" w1734 {
                            selector: w1734 -> [w1737 w1744]
                            tunnel: [w1743 w1748] -> w1730
                            tunnel: w1732 -> [w1742 _]
                            tunnel: w1731 -> [w1741 w1747]
                            tunnel: w1733 -> [w1739 w1746]
                            tunnel: w1729 -> [w1738 w1745]
                            frame False {
                              n674 = Type Cast(type=i16 0, x=w1742) -> (*(type *) &x=w1740:i16)
                              n675 = Not Equal To 0?(x=w1740) -> (x != 0?=w1736:bool)
                              n676 = Bundle By Name(cluster=w1741, "Pw.Pw.DIM Status.quality"=w1739, "Pw.Pw.DIM Status.Time Stamp"=w1738, "Pw.Pw.Pw"=w1736, "Pw.Pw.DIM Status.no link"=w1737) -> (w1743:T11)
                            }
                            frame True {
                              n677 = Bundle By Name(cluster=w1747, "Pw.Pw.DIM Status.quality"=w1746, "Pw.Pw.DIM Status.Time Stamp"=w1745, "Pw.Pw.DIM Status.no link"=w1744) -> (w1748:T11)
                            }
                          }
                        }
                        frame "Pw#CoClose" {
                          n678 = case "no link?" shown="False" w1754 {
                            selector: w1754 -> [w1755 w1762]
                            tunnel: [w1761 w1766] -> w1750
                            tunnel: w1752 -> [w1760 _]
                            tunnel: w1751 -> [w1759 w1765]
                            tunnel: w1753 -> [w1757 w1764]
                            tunnel: w1749 -> [w1756 w1763]
                            frame False {
                              n679 = Type Cast(x=w1760) -> (*(type *) &x=w1758:string)  [unwired: 1 in]
                              n680 = Bundle By Name(cluster=w1759, "Pw.Pw#CoClose.DIM Status.quality"=w1757, "Pw.Pw#CoClose.DIM Status.Time Stamp"=w1756, "Pw.Pw#CoClose.Pw#CoClose"=w1758, "Pw.Pw#CoClose.DIM Status.no link"=w1755) -> (w1761:T11)
                            }
                            frame True {
                              n681 = Bundle By Name(cluster=w1765, "Pw.Pw#CoClose.DIM Status.quality"=w1764, "Pw.Pw#CoClose.DIM Status.Time Stamp"=w1763, "Pw.Pw#CoClose.DIM Status.no link"=w1762) -> (w1766:T11)
                            }
                          }
                        }
                        frame "Pw#CoOpen" {
                          n682 = case "no link?" shown="False" w1772 {
                            selector: w1772 -> [w1773 w1780]
                            tunnel: [w1779 w1784] -> w1768
                            tunnel: w1770 -> [w1778 _]
                            tunnel: w1769 -> [w1777 w1783]
                            tunnel: w1771 -> [w1775 w1782]
                            tunnel: w1767 -> [w1774 w1781]
                            frame False {
                              n683 = Type Cast(x=w1778) -> (*(type *) &x=w1776:string)  [unwired: 1 in]
                              n684 = Bundle By Name(cluster=w1777, "Pw.Pw#CoOpen.DIM Status.quality"=w1775, "Pw.Pw#CoOpen.DIM Status.Time Stamp"=w1774, "Pw.Pw#CoOpen.Pw#CoOpen"=w1776, "Pw.Pw#CoOpen.DIM Status.no link"=w1773) -> (w1779:T11)
                            }
                            frame True {
                              n685 = Bundle By Name(cluster=w1783, "Pw.Pw#CoOpen.DIM Status.quality"=w1782, "Pw.Pw#CoOpen.DIM Status.Time Stamp"=w1781, "Pw.Pw#CoOpen.DIM Status.no link"=w1780) -> (w1784:T11)
                            }
                          }
                        }
                        frame "RDWn" {
                          n686 = case "no link?" shown="False" w1794 {
                            selector: w1794 -> [w1802 w1813]
                            tunnel: [w1804 w1817] -> w1790
                            tunnel: w1792 -> [_ w1816]
                            tunnel: w1791 -> [w1796 w1812]
                            tunnel: w1793 -> [w1801 w1805]
                            tunnel: w1789 -> [w1803 w1814]
                            tunnel: [PSChannelBase.directionType."update actual value" ("direction") PSChannelBase.directionType."update actual value" ("direction")] -> w1788
                            tunnel: [PSChannelBase.serviceType."rampDownSpeed" ("service") PSChannelBase.serviceType."rampDownSpeed" ("service")] -> w1787
                            tunnel: [w1798 w1807] -> w1786
                            tunnel: [UtilityLib.valueStatus."no info available" ("quality") w1805] -> w1785
                            frame True {
                              n687 = Unbundle By Name(w1796) -> ("RDWn.RDWn.RDWn"=w1795:dbl)
                              n688 = Bundle By Name(cluster=w1796, "RDWn.RDWn.DIM Status.quality"=w1801, "RDWn.RDWn.DIM Status.Time Stamp"=w1803, "RDWn.RDWn.DIM Status.no link"=w1802) -> (w1804:T11)
                              n689 = Type Cast(x=w1795) -> (*(type *) &x=w1798:string)  [unwired: 1 in]
                            }
                            frame False {
                              n690 = Type Cast(type=0.0, x=w1816) -> (*(type *) &x=w1815:dbl)
                              n691 = Unbundle By Name(w1812) -> ("RDWn.RDWn#Multiplier"=w1810:dbl)
                              n692 = Multiply(x=w1810, y=w1815) -> (x*y=w1806:dbl)
                              n693 = Bundle By Name(cluster=w1812, "RDWn.RDWn.DIM Status.quality"=w1805, "RDWn.RDWn.DIM Status.Time Stamp"=w1814, "RDWn.RDWn.RDWn"=w1806, "RDWn.RDWn.DIM Status.no link"=w1813) -> (w1817:T11)
                              n694 = Type Cast(x=w1806) -> (*(type *) &x=w1807:string)  [unwired: 1 in]
                            }
                          }
                        }
                        frame "RDWn#EU" {
                          n695 = case "no link?" shown="False" w1827 {
                            selector: w1827 -> [w1834 w1857]
                            tunnel: [w1837 w1860] -> w1823
                            tunnel: w1825 -> [_ w1859]
                            tunnel: w1824 -> [w1830 w1856]
                            tunnel: w1826 -> [w1836 w1838]
                            tunnel: w1822 -> [w1835 w1858]
                            tunnel: [PSChannelBase.directionType."update actual value" ("direction") PSChannelBase.directionType."update actual value" ("direction")] -> w1821
                            tunnel: [PSChannelBase.serviceType."rampUpSpeed" ("service") PSChannelBase.serviceType."rampDownSpeed" ("service")] -> w1820
                            tunnel: [w1831 w1839] -> w1819
                            tunnel: [UtilityLib.valueStatus."no info available" ("quality") w1838] -> w1818
                            frame True {
                              n696 = Unbundle By Name(w1830) -> ("RDWn.RDWn.RDWn"=w1829:dbl)
                              n697 = Bundle By Name(cluster=w1830, "RDWn.RDWn#EU.DIM Status.quality"=w1836, "RDWn.RDWn#EU.DIM Status.Time Stamp"=w1835, "RDWn.RDWn#EU.DIM Status.no link"=w1834) -> (w1837:T11)
                              n698 = Type Cast(x=w1829) -> (*(type *) &x=w1831:string)  [unwired: 1 in]
                            }
                            frame False {
                              n699 = Type Cast(x=w1859) -> (*(type *) &x=w1855:string)  [unwired: 1 in]
                              n700 = Unbundle By Name(w1856) -> ("RDWn.RDWn.RDWn"=w1849:dbl, "RDWn.RDWn#HighEU.RDWn#HighEU"=w1848:dbl, "RDWn.RDWn#LowEU.RDWn#LowEU"=w1847:dbl, "RDWn.RDWn#Multiplier"=w1846:dbl)
                              n701 = call "CAEN_HVSystem.EUString2UnitMultilier.vi"("EU String"=w1855) -> ("Multiplier"=w1845:dbl, "Unit"=w1854:string)  [unwired: 2 in, 1 out]
                              n702 = Build Array(w1849, w1848, w1847) -> (w1851:dbl[])
                              n703 = Divide(x=w1851, y=w1846) -> (x/y=w1850:dbl[])
                              n704 = Multiply(x=w1850, y=w1845) -> (x*y=w1852:dbl[])
                              n705 = Index Array(array=w1852, index #1=0 ("index")) -> (element #1=w1840:dbl, element #2=w1844:dbl, element #3=w1843:dbl)  [unwired: 2 in]
                              n706 = Bundle By Name(cluster=w1856, "RDWn.RDWn.RDWn"=w1840, "RDWn.RDWn#HighEU.RDWn#HighEU"=w1844, "RDWn.RDWn#LowEU.RDWn#LowEU"=w1843, "RDWn.RDWn#Multiplier"=w1845, "RDWn.RDWn#EU.DIM Status.quality"=w1838, "RDWn.RDWn#EU.DIM Status.Time Stamp"=w1858, "RDWn.RDWn#EU.RDWn#EU"=w1854, "RDWn.RDWn#EU.DIM Status.no link"=w1857) -> (w1860:T11)
                              n707 = Type Cast(x=w1840) -> (*(type *) &x=w1839:string)  [unwired: 1 in]
                            }
                          }
                        }
                        frame "RDWn#HighEU" {
                          n708 = case "no link?" shown="False" w1866 {
                            selector: w1866 -> [w1867 w1876]
                            tunnel: [w1871 w1881] -> w1862
                            tunnel: w1864 -> [_ w1880]
                            tunnel: w1863 -> [w1870 w1875]
                            tunnel: w1865 -> [w1869 w1878]
                            tunnel: w1861 -> [w1868 w1877]
                            frame True {
                              n709 = Bundle By Name(cluster=w1870, "RDWn.RDWn#HighEU.DIM Status.quality"=w1869, "RDWn.RDWn#HighEU.DIM Status.Time Stamp"=w1868, "RDWn.RDWn#HighEU.DIM Status.no link"=w1867) -> (w1871:T11)
                            }
                            frame False {
                              n710 = Type Cast(type=0.0, x=w1880) -> (*(type *) &x=w1879:dbl)
                              n711 = Unbundle By Name(w1875) -> ("RDWn.RDWn#Multiplier"=w1872:dbl)
                              n712 = Multiply(x=w1872, y=w1879) -> (x*y=w1873:dbl)
                              n713 = Bundle By Name(cluster=w1875, "RDWn.RDWn#HighEU.DIM Status.quality"=w1878, "RDWn.RDWn#HighEU.DIM Status.Time Stamp"=w1877, "RDWn.RDWn#HighEU.RDWn#HighEU"=w1873, "RDWn.RDWn#HighEU.DIM Status.no link"=w1876) -> (w1881:T11)
                            }
                          }
                        }
                        frame "RDWn#LowEU" {
                          n714 = case "no link?" shown="False" w1887 {
                            selector: w1887 -> [w1888 w1897]
                            tunnel: [w1892 w1902] -> w1883
                            tunnel: w1885 -> [_ w1901]
                            tunnel: w1884 -> [w1891 w1896]
                            tunnel: w1886 -> [w1890 w1899]
                            tunnel: w1882 -> [w1889 w1898]
                            frame True {
                              n715 = Bundle By Name(cluster=w1891, "RDWn.RDWn#LowEU.DIM Status.quality"=w1890, "RDWn.RDWn#LowEU.DIM Status.Time Stamp"=w1889, "RDWn.RDWn#LowEU.DIM Status.no link"=w1888) -> (w1892:T11)
                            }
                            frame False {
                              n716 = Type Cast(type=0.0, x=w1901) -> (*(type *) &x=w1900:dbl)
                              n717 = Unbundle By Name(w1896) -> ("RDWn.RDWn#Multiplier"=w1893:dbl)
                              n718 = Multiply(x=w1893, y=w1900) -> (x*y=w1894:dbl)
                              n719 = Bundle By Name(cluster=w1896, "RDWn.RDWn#LowEU.DIM Status.quality"=w1899, "RDWn.RDWn#LowEU.DIM Status.Time Stamp"=w1898, "RDWn.RDWn#LowEU.RDWn#LowEU"=w1894, "RDWn.RDWn#LowEU.DIM Status.no link"=w1897) -> (w1902:T11)
                            }
                          }
                        }
                        frame "RUp" {
                          n720 = case "no link?" shown="False" w1912 {
                            selector: w1912 -> [w1920 w1931]
                            tunnel: [w1922 w1935] -> w1908
                            tunnel: w1910 -> [_ w1934]
                            tunnel: w1909 -> [w1914 w1930]
                            tunnel: w1911 -> [w1919 w1923]
                            tunnel: w1907 -> [w1921 w1932]
                            tunnel: [PSChannelBase.directionType."update actual value" ("direction") PSChannelBase.directionType."update actual value" ("direction")] -> w1906
                            tunnel: [PSChannelBase.serviceType."rampUpSpeed" ("service") PSChannelBase.serviceType."rampUpSpeed" ("service")] -> w1905
                            tunnel: [w1915 w1925] -> w1904
                            tunnel: [UtilityLib.valueStatus."no info available" ("quality") w1923] -> w1903
                            frame True {
                              n721 = Unbundle By Name(w1914) -> ("RUp.RUp.RUp"=w1913:dbl)
                              n722 = Bundle By Name(cluster=w1914, "RUp.RUp.DIM Status.quality"=w1919, "RUp.RUp.DIM Status.Time Stamp"=w1921, "RUp.RUp.DIM Status.no link"=w1920) -> (w1922:T11)
                              n723 = Type Cast(x=w1913) -> (*(type *) &x=w1915:string)  [unwired: 1 in]
                            }
                            frame False {
                              n724 = Type Cast(type=0.0, x=w1934) -> (*(type *) &x=w1933:dbl)
                              n725 = Unbundle By Name(w1930) -> ("RUp.RUp#Multiplier"=w1928:dbl)
                              n726 = Multiply(x=w1928, y=w1933) -> (x*y=w1924:dbl)
                              n727 = Bundle By Name(cluster=w1930, "RUp.RUp.DIM Status.quality"=w1923, "RUp.RUp.DIM Status.Time Stamp"=w1932, "RUp.RUp.RUp"=w1924, "RUp.RUp.DIM Status.no link"=w1931) -> (w1935:T11)
                              n728 = Type Cast(x=w1924) -> (*(type *) &x=w1925:string)  [unwired: 1 in]
                            }
                          }
                        }
                        frame "RUp#EU" {
                          n729 = case "no link?" shown="False" w1945 {
                            selector: w1945 -> [w1952 w1975]
                            tunnel: [w1955 w1978] -> w1941
                            tunnel: w1943 -> [_ w1977]
                            tunnel: w1942 -> [w1947 w1974]
                            tunnel: w1944 -> [w1954 w1956]
                            tunnel: w1940 -> [w1953 w1976]
                            tunnel: [PSChannelBase.directionType."update actual value" ("direction") PSChannelBase.directionType."update actual value" ("direction")] -> w1939
                            tunnel: [PSChannelBase.serviceType."rampUpSpeed" ("service") PSChannelBase.serviceType."rampUpSpeed" ("service")] -> w1938
                            tunnel: [w1948 w1957] -> w1937
                            tunnel: [UtilityLib.valueStatus."no info available" ("quality") w1956] -> w1936
                            frame True {
                              n730 = Unbundle By Name(w1947) -> ("RUp.RUp.RUp"=w1946:dbl)
                              n731 = Bundle By Name(cluster=w1947, "RUp.RUp#EU.DIM Status.quality"=w1954, "RUp.RUp#EU.DIM Status.Time Stamp"=w1953, "RUp.RUp#EU.DIM Status.no link"=w1952) -> (w1955:T11)
                              n732 = Type Cast(x=w1946) -> (*(type *) &x=w1948:string)  [unwired: 1 in]
                            }
                            frame False {
                              n733 = Type Cast(x=w1977) -> (*(type *) &x=w1973:string)  [unwired: 1 in]
                              n734 = Unbundle By Name(w1974) -> ("RUp.RUp.RUp"=w1967:dbl, "RUp.RUp#HighEU.RUp#HighEU"=w1966:dbl, "RUp.RUp#LowEU.RUp#LowEU"=w1965:dbl, "RUp.RUp#Multiplier"=w1964:dbl)
                              n735 = call "CAEN_HVSystem.EUString2UnitMultilier.vi"("EU String"=w1973) -> ("Multiplier"=w1963:dbl, "Unit"=w1972:string)  [unwired: 2 in, 1 out]
                              n736 = Build Array(w1967, w1966, w1965) -> (w1969:dbl[])
                              n737 = Divide(x=w1969, y=w1964) -> (x/y=w1968:dbl[])
                              n738 = Multiply(x=w1968, y=w1963) -> (x*y=w1970:dbl[])
                              n739 = Index Array(array=w1970, index #1=0 ("index")) -> (element #1=w1958:dbl, element #2=w1962:dbl, element #3=w1961:dbl)  [unwired: 2 in]
                              n740 = Bundle By Name(cluster=w1974, "RUp.RUp.RUp"=w1958, "RUp.RUp#HighEU.RUp#HighEU"=w1962, "RUp.RUp#LowEU.RUp#LowEU"=w1961, "RUp.RUp#Multiplier"=w1963, "RUp.RUp#EU.DIM Status.quality"=w1956, "RUp.RUp#EU.DIM Status.Time Stamp"=w1976, "RUp.RUp#EU.RUp#EU"=w1972, "RUp.RUp#EU.DIM Status.no link"=w1975) -> (w1978:T11)
                              n741 = Type Cast(x=w1958) -> (*(type *) &x=w1957:string)  [unwired: 1 in]
                            }
                          }
                        }
                        frame "RUp#HighEU" {
                          n742 = case "no link?" shown="False" w1984 {
                            selector: w1984 -> [w1985 w1994]
                            tunnel: [w1989 w1999] -> w1980
                            tunnel: w1982 -> [_ w1998]
                            tunnel: w1981 -> [w1988 w1993]
                            tunnel: w1983 -> [w1987 w1996]
                            tunnel: w1979 -> [w1986 w1995]
                            frame True {
                              n743 = Bundle By Name(cluster=w1988, "RUp.RUp#HighEU.DIM Status.quality"=w1987, "RUp.RUp#HighEU.DIM Status.Time Stamp"=w1986, "RUp.RUp#HighEU.DIM Status.no link"=w1985) -> (w1989:T11)
                            }
                            frame False {
                              n744 = Type Cast(type=0.0, x=w1998) -> (*(type *) &x=w1997:dbl)
                              n745 = Unbundle By Name(w1993) -> ("RUp.RUp#Multiplier"=w1990:dbl)
                              n746 = Multiply(x=w1990, y=w1997) -> (x*y=w1991:dbl)
                              n747 = Bundle By Name(cluster=w1993, "RUp.RUp#HighEU.DIM Status.quality"=w1996, "RUp.RUp#HighEU.DIM Status.Time Stamp"=w1995, "RUp.RUp#HighEU.RUp#HighEU"=w1991, "RUp.RUp#HighEU.DIM Status.no link"=w1994) -> (w1999:T11)
                            }
                          }
                        }
                        frame "RUp#LowEU" {
                          n748 = case "no link?" shown="False" w2005 {
                            selector: w2005 -> [w2006 w2015]
                            tunnel: [w2010 w2020] -> w2001
                            tunnel: w2003 -> [_ w2019]
                            tunnel: w2002 -> [w2009 w2014]
                            tunnel: w2004 -> [w2008 w2017]
                            tunnel: w2000 -> [w2007 w2016]
                            frame True {
                              n749 = Bundle By Name(cluster=w2009, "RUp.RUp#LowEU.DIM Status.quality"=w2008, "RUp.RUp#LowEU.DIM Status.Time Stamp"=w2007, "RUp.RUp#LowEU.DIM Status.no link"=w2006) -> (w2010:T11)
                            }
                            frame False {
                              n750 = Type Cast(type=0.0, x=w2019) -> (*(type *) &x=w2018:dbl)
                              n751 = Unbundle By Name(w2014) -> ("RUp.RUp#Multiplier"=w2011:dbl)
                              n752 = Multiply(x=w2011, y=w2018) -> (x*y=w2012:dbl)
                              n753 = Bundle By Name(cluster=w2014, "RUp.RUp#LowEU.DIM Status.quality"=w2017, "RUp.RUp#LowEU.DIM Status.Time Stamp"=w2016, "RUp.RUp#LowEU.RUp#LowEU"=w2012, "RUp.RUp#LowEU.DIM Status.no link"=w2015) -> (w2020:T11)
                            }
                          }
                        }
                        frame "SVMax" {
                          n754 = case "no link?" shown="False" w2026 {
                            selector: w2026 -> [w2029 w2037]
                            tunnel: [w2031 w2041] -> w2022
                            tunnel: w2024 -> [_ w2040]
                            tunnel: w2023 -> [w2028 w2036]
                            tunnel: w2025 -> [w2027 w2032]
                            tunnel: w2021 -> [w2030 w2038]
                            frame True {
                              n755 = Bundle By Name(cluster=w2028, "SVMax.SVMax.DIM Status.quality"=w2027, "SVMax.SVMax.DIM Status.Time Stamp"=w2030, "SVMax.SVMax.DIM Status.no link"=w2029) -> (w2031:T11)
                            }
                            frame False {
                              n756 = Type Cast(type=0.0, x=w2040) -> (*(type *) &x=w2039:dbl)
                              n757 = Unbundle By Name(w2036) -> ("SVMax.SVMax#Multiplier"=w2034:dbl)
                              n758 = Multiply(x=w2034, y=w2039) -> (x*y=w2033:dbl)
                              n759 = Bundle By Name(cluster=w2036, "SVMax.SVMax.DIM Status.quality"=w2032, "SVMax.SVMax.DIM Status.Time Stamp"=w2038, "SVMax.SVMax.SVMax"=w2033, "SVMax.SVMax.DIM Status.no link"=w2037) -> (w2041:T11)
                            }
                          }
                        }
                        frame "SVMax#EU" {
                          n760 = case "no link?" shown="False" w2047 {
                            selector: w2047 -> [w2048 w2068]
                            tunnel: [w2052 w2072] -> w2043
                            tunnel: w2045 -> [_ w2071]
                            tunnel: w2044 -> [w2051 w2067]
                            tunnel: w2046 -> [w2050 w2070]
                            tunnel: w2042 -> [w2049 w2069]
                            frame True {
                              n761 = Bundle By Name(cluster=w2051, "SVMax.SVMax#EU.DIM Status.quality"=w2050, "SVMax.SVMax#EU.DIM Status.Time Stamp"=w2049, "SVMax.SVMax#EU.DIM Status.no link"=w2048) -> (w2052:T11)
                            }
                            frame False {
                              n762 = Type Cast(x=w2071) -> (*(type *) &x=w2066:string)  [unwired: 1 in]
                              n763 = Unbundle By Name(w2067) -> ("SVMax.SVMax.SVMax"=w2060:dbl, "SVMax.SVMax#HighEU.SVMax#HighEU"=w2059:dbl, "SVMax.SVMax#LowEU.SVMax#LowEU"=w2058:dbl, "SVMax.SVMax#Multiplier"=w2057:dbl)
                              n764 = call "CAEN_HVSystem.EUString2UnitMultilier.vi"("EU String"=w2066) -> ("Multiplier"=w2056:dbl, "Unit"=w2065:string)  [unwired: 2 in, 1 out]
                              n765 = Build Array(w2060, w2059, w2058) -> (w2062:dbl[])
                              n766 = Divide(x=w2062, y=w2057) -> (x/y=w2061:dbl[])
                              n767 = Multiply(x=w2061, y=w2056) -> (x*y=w2063:dbl[])
                              n768 = Index Array(array=w2063, index #1=0 ("index")) -> (element #1=w2055:dbl, element #2=w2054:dbl, element #3=w2053:dbl)  [unwired: 2 in]
                              n769 = Bundle By Name(cluster=w2067, "SVMax.SVMax.SVMax"=w2055, "SVMax.SVMax#HighEU.SVMax#HighEU"=w2054, "SVMax.SVMax#LowEU.SVMax#LowEU"=w2053, "SVMax.SVMax#Multiplier"=w2056, "SVMax.SVMax#EU.DIM Status.quality"=w2070, "SVMax.SVMax#EU.DIM Status.Time Stamp"=w2069, "SVMax.SVMax#EU.SVMax#EU"=w2065, "SVMax.SVMax#EU.DIM Status.no link"=w2068) -> (w2072:T11)
                            }
                          }
                        }
                        frame "SVMax#HighEU" {
                          n770 = case "no link?" shown="False" w2078 {
                            selector: w2078 -> [w2079 w2088]
                            tunnel: [w2083 w2093] -> w2074
                            tunnel: w2076 -> [_ w2092]
                            tunnel: w2075 -> [w2082 w2087]
                            tunnel: w2077 -> [w2081 w2090]
                            tunnel: w2073 -> [w2080 w2089]
                            frame True {
                              n771 = Bundle By Name(cluster=w2082, "SVMax.SVMax#HighEU.DIM Status.quality"=w2081, "SVMax.SVMax#HighEU.DIM Status.Time Stamp"=w2080, "SVMax.SVMax#HighEU.DIM Status.no link"=w2079) -> (w2083:T11)
                            }
                            frame False {
                              n772 = Type Cast(type=0.0, x=w2092) -> (*(type *) &x=w2091:dbl)
                              n773 = Unbundle By Name(w2087) -> ("SVMax.SVMax#Multiplier"=w2084:dbl)
                              n774 = Multiply(x=w2084, y=w2091) -> (x*y=w2085:dbl)
                              n775 = Bundle By Name(cluster=w2087, "SVMax.SVMax#HighEU.DIM Status.quality"=w2090, "SVMax.SVMax#HighEU.DIM Status.Time Stamp"=w2089, "SVMax.SVMax#HighEU.SVMax#HighEU"=w2085, "SVMax.SVMax#HighEU.DIM Status.no link"=w2088) -> (w2093:T11)
                            }
                          }
                        }
                        frame "SVMax#LowEU" {
                          n776 = case "no link?" shown="False" w2099 {
                            selector: w2099 -> [w2100 w2109]
                            tunnel: [w2104 w2114] -> w2095
                            tunnel: w2097 -> [_ w2113]
                            tunnel: w2096 -> [w2103 w2108]
                            tunnel: w2098 -> [w2102 w2111]
                            tunnel: w2094 -> [w2101 w2110]
                            frame True {
                              n777 = Bundle By Name(cluster=w2103, "SVMax.SVMax#LowEU.DIM Status.quality"=w2102, "SVMax.SVMax#LowEU.DIM Status.Time Stamp"=w2101, "SVMax.SVMax#LowEU.DIM Status.no link"=w2100) -> (w2104:T11)
                            }
                            frame False {
                              n778 = Type Cast(type=0.0, x=w2113) -> (*(type *) &x=w2112:dbl)
                              n779 = Unbundle By Name(w2108) -> ("SVMax.SVMax#Multiplier"=w2105:dbl)
                              n780 = Multiply(x=w2105, y=w2112) -> (x*y=w2106:dbl)
                              n781 = Bundle By Name(cluster=w2108, "SVMax.SVMax#LowEU.DIM Status.quality"=w2111, "SVMax.SVMax#LowEU.DIM Status.Time Stamp"=w2110, "SVMax.SVMax#LowEU.SVMax#LowEU"=w2106, "SVMax.SVMax#LowEU.DIM Status.no link"=w2109) -> (w2114:T11)
                            }
                          }
                        }
                        frame "Status" {
                          n782 = case "no link?" shown="False" w2128 {
                            selector: w2128 -> [w2136 w2172]
                            tunnel: [w2138 w2175] -> w2124
                            tunnel: w2126 -> [_ w2174]
                            tunnel: w2125 -> [w2135 w2171]
                            tunnel: w2127 -> [w2133 w2145]
                            tunnel: w2123 -> [w2137 w2173]
                            tunnel: [PSChannelBase.directionType."update actual value" ("direction") PSChannelBase.directionType."update actual value" ("direction")] -> w2122
                            tunnel: [w2134 w2167] -> w2121
                            tunnel: [PSChannelBase.serviceType."status" ("service") PSChannelBase.serviceType."status" ("service")] -> w2120
                            tunnel: [UtilityLib.valueStatus."no info available" ("quality") w2145] -> w2119
                            tunnel: w2118 -> [_ _]
                            tunnel: w2117 -> [_ _]
                            tunnel: w2116 -> [_ _]
                            tunnel: w2115 -> [w2129 w2163]
                            frame True {
                              n783 = Bundle By Name(cluster=w2135, "Status.DIM Status.quality"=w2133, "Status.DIM Status.Time Stamp"=w2137, "Status.DIM Status.no link"=w2136) -> (w2138:T11)
                              n784 = Type Cast(x=w2129) -> (*(type *) &x=w2134:string)  [unwired: 1 in]
                            }
                            frame False {
                              w2144 = 1  # OnOff
                              w2148 = 54456  # Error
                              w2158 = 576  # Tripped
                              w2166 = 6  # Ramping Flags
                              w2164 = 2  # Flags to keep
                              n785 = Type Cast(type=0.0, x=w2174) -> (*(type *) &x=w2147:dbl)
                              n786 = To Long Integer(number=w2147) -> (32bit integer=w2139:i32)
                              n787 = And(x=w2163, y=w2164) -> (x .and. y?=w2162:i32)
                              n788 = And(x=w2139, y=w2148) -> (x .and. y?=w2149:i32)
                              n789 = And(x=w2139, y=w2158) -> (x .and. y?=w2157:i32)
                              n790 = Not Equal To 0?(x=w2149) -> (x != 0?=w2151:bool)
                              n791 = Not Equal To 0?(x=w2157) -> (x != 0?=w2155:bool)
                              n792 = And(x=w2166, y=w2139) -> (x .and. y?=w2159:i32)
                              n793 = Boolean To (0,1)(Boolean=w2151) -> (0, 1=w2152:i16)
                              n794 = Boolean To (0,1)(Boolean=w2155) -> (0, 1=w2154:i16)
                              n795 = To Long Integer(number=w2152) -> (32bit integer=w2140:i32)
                              n796 = To Long Integer(number=w2154) -> (32bit integer=w2141:i32)
                              n797 = Logical Shift(y=1, x=w2159) -> (x << y=w2160:i32)
                              n798 = Logical Shift(y=5, x=w2140) -> (x << y=w2146:i32)
                              n799 = Logical Shift(y=4, x=w2141) -> (x << y=w2153:i32)
                              n800 = And(x=w2144, y=w2139) -> (x .and. y?=w2143:i32)
                              n801 = Compound Arithmetic op=OR(w2162, w2160, w2153, w2143, w2146) -> (w2161:i32)
                              n802 = To Word Integer(number=w2139) -> (16bit integer=w2142:i16)
                              n803 = Bundle By Name(cluster=w2171, "Status.DIM Status.quality"=w2145, "Status.DIM Status.Time Stamp"=w2173, "Status.Status"=w2142, "Status.DIM Status.no link"=w2172) -> (w2175:T11)
                              n804 = Type Cast(x=w2161) -> (*(type *) &x=w2167:string)  [unwired: 1 in]
                            }
                          }
                        }
                        frame "Trip" {
                          n805 = case "no link?" shown="False" w2181 {
                            selector: w2181 -> [w2184 w2192]
                            tunnel: [w2186 w2196] -> w2177
                            tunnel: w2179 -> [_ w2195]
                            tunnel: w2178 -> [w2183 w2191]
                            tunnel: w2180 -> [w2182 w2187]
                            tunnel: w2176 -> [w2185 w2193]
                            frame True {
                              n806 = Bundle By Name(cluster=w2183, "Trip.Trip.DIM Status.quality"=w2182, "Trip.Trip.DIM Status.Time Stamp"=w2185, "Trip.Trip.DIM Status.no link"=w2184) -> (w2186:T11)
                            }
                            frame False {
                              n807 = Type Cast(type=0.0, x=w2195) -> (*(type *) &x=w2194:dbl)
                              n808 = Unbundle By Name(w2191) -> ("Trip.Trip#Multiplier"=w2189:dbl)
                              n809 = Multiply(x=w2189, y=w2194) -> (x*y=w2188:dbl)
                              n810 = Bundle By Name(cluster=w2191, "Trip.Trip.DIM Status.quality"=w2187, "Trip.Trip.DIM Status.Time Stamp"=w2193, "Trip.Trip.Trip"=w2188, "Trip.Trip.DIM Status.no link"=w2192) -> (w2196:T11)
                            }
                          }
                        }
                        frame "Trip#EU" {
                          n811 = case "no link?" shown="False" w2202 {
                            selector: w2202 -> [w2203 w2223]
                            tunnel: [w2207 w2227] -> w2198
                            tunnel: w2200 -> [_ w2226]
                            tunnel: w2199 -> [w2206 w2222]
                            tunnel: w2201 -> [w2205 w2225]
                            tunnel: w2197 -> [w2204 w2224]
                            frame True {
                              n812 = Bundle By Name(cluster=w2206, "Trip.Trip#EU.DIM Status.quality"=w2205, "Trip.Trip#EU.DIM Status.Time Stamp"=w2204, "Trip.Trip#EU.DIM Status.no link"=w2203) -> (w2207:T11)
                            }
                            frame False {
                              n813 = Type Cast(x=w2226) -> (*(type *) &x=w2221:string)  [unwired: 1 in]
                              n814 = Unbundle By Name(w2222) -> ("Trip.Trip.Trip"=w2215:dbl, "Trip.Trip#HighEU.Trip#HighEU"=w2214:dbl, "Trip.Trip#LowEU.Trip#LowEU"=w2213:dbl, "Trip.Trip#Multiplier"=w2212:dbl)
                              n815 = call "CAEN_HVSystem.EUString2UnitMultilier.vi"("EU String"=w2221) -> ("Multiplier"=w2211:dbl, "Unit"=w2220:string)  [unwired: 2 in, 1 out]
                              n816 = Build Array(w2215, w2214, w2213) -> (w2217:dbl[])
                              n817 = Divide(x=w2217, y=w2212) -> (x/y=w2216:dbl[])
                              n818 = Multiply(x=w2216, y=w2211) -> (x*y=w2218:dbl[])
                              n819 = Index Array(array=w2218, index #1=0 ("index")) -> (element #1=w2210:dbl, element #2=w2209:dbl, element #3=w2208:dbl)  [unwired: 2 in]
                              n820 = Bundle By Name(cluster=w2222, "Trip.Trip.Trip"=w2210, "Trip.Trip#HighEU.Trip#HighEU"=w2209, "Trip.Trip#LowEU.Trip#LowEU"=w2208, "Trip.Trip#Multiplier"=w2211, "Trip.Trip#EU.DIM Status.quality"=w2225, "Trip.Trip#EU.DIM Status.Time Stamp"=w2224, "Trip.Trip#EU.Trip#EU"=w2220, "Trip.Trip#EU.DIM Status.no link"=w2223) -> (w2227:T11)
                            }
                          }
                        }
                        frame "Trip#HighEU" {
                          n821 = case "no link?" shown="False" w2233 {
                            selector: w2233 -> [w2234 w2243]
                            tunnel: [w2238 w2248] -> w2229
                            tunnel: w2231 -> [_ w2247]
                            tunnel: w2230 -> [w2237 w2242]
                            tunnel: w2232 -> [w2236 w2245]
                            tunnel: w2228 -> [w2235 w2244]
                            frame True {
                              n822 = Bundle By Name(cluster=w2237, "Trip.Trip#HighEU.DIM Status.quality"=w2236, "Trip.Trip#HighEU.DIM Status.Time Stamp"=w2235, "Trip.Trip#HighEU.DIM Status.no link"=w2234) -> (w2238:T11)
                            }
                            frame False {
                              n823 = Type Cast(type=0.0, x=w2247) -> (*(type *) &x=w2246:dbl)
                              n824 = Unbundle By Name(w2242) -> ("Trip.Trip#Multiplier"=w2239:dbl)
                              n825 = Multiply(x=w2239, y=w2246) -> (x*y=w2240:dbl)
                              n826 = Bundle By Name(cluster=w2242, "Trip.Trip#HighEU.DIM Status.quality"=w2245, "Trip.Trip#HighEU.DIM Status.Time Stamp"=w2244, "Trip.Trip#HighEU.Trip#HighEU"=w2240, "Trip.Trip#HighEU.DIM Status.no link"=w2243) -> (w2248:T11)
                            }
                          }
                        }
                        frame "Trip#LowEU" {
                          n827 = case "no link?" shown="False" w2254 {
                            selector: w2254 -> [w2255 w2264]
                            tunnel: [w2259 w2269] -> w2250
                            tunnel: w2252 -> [_ w2268]
                            tunnel: w2251 -> [w2258 w2263]
                            tunnel: w2253 -> [w2257 w2266]
                            tunnel: w2249 -> [w2256 w2265]
                            frame True {
                              n828 = Bundle By Name(cluster=w2258, "Trip.Trip#LowEU.DIM Status.quality"=w2257, "Trip.Trip#LowEU.DIM Status.Time Stamp"=w2256, "Trip.Trip#LowEU.DIM Status.no link"=w2255) -> (w2259:T11)
                            }
                            frame False {
                              n829 = Type Cast(type=0.0, x=w2268) -> (*(type *) &x=w2267:dbl)
                              n830 = Unbundle By Name(w2263) -> ("Trip.Trip#Multiplier"=w2260:dbl)
                              n831 = Multiply(x=w2260, y=w2267) -> (x*y=w2261:dbl)
                              n832 = Bundle By Name(cluster=w2263, "Trip.Trip#LowEU.DIM Status.quality"=w2266, "Trip.Trip#LowEU.DIM Status.Time Stamp"=w2265, "Trip.Trip#LowEU.Trip#LowEU"=w2261, "Trip.Trip#LowEU.DIM Status.no link"=w2264) -> (w2269:T11)
                            }
                          }
                        }
                        frame "TripExt" {
                          n833 = case "no link?" shown="False" w2275 {
                            selector: w2275 -> [w2278 w2286]
                            tunnel: [w2280 w2290] -> w2271
                            tunnel: w2273 -> [_ w2289]
                            tunnel: w2272 -> [w2277 w2285]
                            tunnel: w2274 -> [w2276 w2281]
                            tunnel: w2270 -> [w2279 w2287]
                            frame True {
                              n834 = Bundle By Name(cluster=w2277, "TripExt.TripExt.DIM Status.quality"=w2276, "TripExt.TripExt.DIM Status.Time Stamp"=w2279, "TripExt.TripExt.DIM Status.no link"=w2278) -> (w2280:T11)
                            }
                            frame False {
                              n835 = Type Cast(type=0.0, x=w2289) -> (*(type *) &x=w2288:dbl)
                              n836 = Unbundle By Name(w2285) -> ("TripExt.TripExt#Multiplier"=w2283:dbl)
                              n837 = Multiply(x=w2283, y=w2288) -> (x*y=w2282:dbl)
                              n838 = Bundle By Name(cluster=w2285, "TripExt.TripExt.DIM Status.quality"=w2281, "TripExt.TripExt.DIM Status.Time Stamp"=w2287, "TripExt.TripExt.TripExt"=w2282, "TripExt.TripExt.DIM Status.no link"=w2286) -> (w2290:T11)
                            }
                          }
                        }
                        frame "TripExt#EU" {
                          n839 = case "no link?" shown="False" w2296 {
                            selector: w2296 -> [w2297 w2317]
                            tunnel: [w2301 w2321] -> w2292
                            tunnel: w2294 -> [_ w2320]
                            tunnel: w2293 -> [w2300 w2316]
                            tunnel: w2295 -> [w2299 w2319]
                            tunnel: w2291 -> [w2298 w2318]
                            frame True {
                              n840 = Bundle By Name(cluster=w2300, "TripExt.TripExt#EU.DIM Status.quality"=w2299, "TripExt.TripExt#EU.DIM Status.Time Stamp"=w2298, "TripExt.TripExt#EU.DIM Status.no link"=w2297) -> (w2301:T11)
                            }
                            frame False {
                              n841 = Type Cast(x=w2320) -> (*(type *) &x=w2315:string)  [unwired: 1 in]
                              n842 = Unbundle By Name(w2316) -> ("TripExt.TripExt.TripExt"=w2309:dbl, "TripExt.TripExt#HighEU.TripExt#HighEU"=w2308:dbl, "TripExt.TripExt#LowEU.TripExt#LowEU"=w2307:dbl, "TripExt.TripExt#Multiplier"=w2306:dbl)
                              n843 = call "CAEN_HVSystem.EUString2UnitMultilier.vi"("EU String"=w2315) -> ("Multiplier"=w2305:dbl, "Unit"=w2314:string)  [unwired: 2 in, 1 out]
                              n844 = Build Array(w2309, w2308, w2307) -> (w2311:dbl[])
                              n845 = Divide(x=w2311, y=w2306) -> (x/y=w2310:dbl[])
                              n846 = Multiply(x=w2310, y=w2305) -> (x*y=w2312:dbl[])
                              n847 = Index Array(array=w2312, index #1=0 ("index")) -> (element #1=w2304:dbl, element #2=w2303:dbl, element #3=w2302:dbl)  [unwired: 2 in]
                              n848 = Bundle By Name(cluster=w2316, "TripExt.TripExt.TripExt"=w2304, "TripExt.TripExt#HighEU.TripExt#HighEU"=w2303, "TripExt.TripExt#LowEU.TripExt#LowEU"=w2302, "TripExt.TripExt#Multiplier"=w2305, "TripExt.TripExt#EU.DIM Status.quality"=w2319, "TripExt.TripExt#EU.DIM Status.Time Stamp"=w2318, "TripExt.TripExt#EU.TripExt#EU"=w2314, "TripExt.TripExt#EU.DIM Status.no link"=w2317) -> (w2321:T11)
                            }
                          }
                        }
                        frame "TripExt#HighEU" {
                          n849 = case "no link?" shown="True" w2327 {
                            selector: w2327 -> [w2328 w2337]
                            tunnel: [w2332 w2342] -> w2323
                            tunnel: w2325 -> [_ w2341]
                            tunnel: w2324 -> [w2331 w2336]
                            tunnel: w2326 -> [w2330 w2339]
                            tunnel: w2322 -> [w2329 w2338]
                            frame True {
                              n850 = Bundle By Name(cluster=w2331, "TripExt.TripExt#HighEU.DIM Status.quality"=w2330, "TripExt.TripExt#HighEU.DIM Status.Time Stamp"=w2329, "TripExt.TripExt#HighEU.DIM Status.no link"=w2328) -> (w2332:T11)
                            }
                            frame False {
                              n851 = Type Cast(type=0.0, x=w2341) -> (*(type *) &x=w2340:dbl)
                              n852 = Unbundle By Name(w2336) -> ("TripExt.TripExt#Multiplier"=w2333:dbl)
                              n853 = Multiply(x=w2333, y=w2340) -> (x*y=w2334:dbl)
                              n854 = Bundle By Name(cluster=w2336, "TripExt.TripExt#HighEU.DIM Status.quality"=w2339, "TripExt.TripExt#HighEU.DIM Status.Time Stamp"=w2338, "TripExt.TripExt#HighEU.TripExt#HighEU"=w2334, "TripExt.TripExt#HighEU.DIM Status.no link"=w2337) -> (w2342:T11)
                            }
                          }
                        }
                        frame "TripExt#LowEU" {
                          n855 = case "no link?" shown="False" w2348 {
                            selector: w2348 -> [w2349 w2358]
                            tunnel: [w2353 w2363] -> w2344
                            tunnel: w2346 -> [_ w2362]
                            tunnel: w2345 -> [w2352 w2357]
                            tunnel: w2347 -> [w2351 w2360]
                            tunnel: w2343 -> [w2350 w2359]
                            frame True {
                              n856 = Bundle By Name(cluster=w2352, "TripExt.TripExt#LowEU.DIM Status.quality"=w2351, "TripExt.TripExt#LowEU.DIM Status.Time Stamp"=w2350, "TripExt.TripExt#LowEU.DIM Status.no link"=w2349) -> (w2353:T11)
                            }
                            frame False {
                              n857 = Type Cast(type=0.0, x=w2362) -> (*(type *) &x=w2361:dbl)
                              n858 = Unbundle By Name(w2357) -> ("TripExt.TripExt#Multiplier"=w2354:dbl)
                              n859 = Multiply(x=w2354, y=w2361) -> (x*y=w2355:dbl)
                              n860 = Bundle By Name(cluster=w2357, "TripExt.TripExt#LowEU.DIM Status.quality"=w2360, "TripExt.TripExt#LowEU.DIM Status.Time Stamp"=w2359, "TripExt.TripExt#LowEU.TripExt#LowEU"=w2355, "TripExt.TripExt#LowEU.DIM Status.no link"=w2358) -> (w2363:T11)
                            }
                          }
                        }
                        frame "TripInt" {
                          n861 = case "no link?" shown="False" w2369 {
                            selector: w2369 -> [w2372 w2380]
                            tunnel: [w2374 w2384] -> w2365
                            tunnel: w2367 -> [_ w2383]
                            tunnel: w2366 -> [w2371 w2379]
                            tunnel: w2368 -> [w2370 w2375]
                            tunnel: w2364 -> [w2373 w2381]
                            frame True {
                              n862 = Bundle By Name(cluster=w2371, "TripInt.TripInt.DIM Status.quality"=w2370, "TripInt.TripInt.DIM Status.Time Stamp"=w2373, "TripInt.TripInt.DIM Status.no link"=w2372) -> (w2374:T11)
                            }
                            frame False {
                              n863 = Type Cast(type=0.0, x=w2383) -> (*(type *) &x=w2382:dbl)
                              n864 = Unbundle By Name(w2379) -> ("TripInt.TripInt#Multiplier"=w2377:dbl)
                              n865 = Multiply(x=w2377, y=w2382) -> (x*y=w2376:dbl)
                              n866 = Bundle By Name(cluster=w2379, "TripInt.TripInt.DIM Status.quality"=w2375, "TripInt.TripInt.DIM Status.Time Stamp"=w2381, "TripInt.TripInt.TripInt"=w2376, "TripInt.TripInt.DIM Status.no link"=w2380) -> (w2384:T11)
                            }
                          }
                        }
                        frame "TripInt#EU" {
                          n867 = case "no link?" shown="False" w2390 {
                            selector: w2390 -> [w2391 w2411]
                            tunnel: [w2395 w2415] -> w2386
                            tunnel: w2388 -> [_ w2414]
                            tunnel: w2387 -> [w2394 w2410]
                            tunnel: w2389 -> [w2393 w2413]
                            tunnel: w2385 -> [w2392 w2412]
                            frame True {
                              n868 = Bundle By Name(cluster=w2394, "TripInt.TripInt#EU.DIM Status.quality"=w2393, "TripInt.TripInt#EU.DIM Status.Time Stamp"=w2392, "TripInt.TripInt#EU.DIM Status.no link"=w2391) -> (w2395:T11)
                            }
                            frame False {
                              n869 = Type Cast(x=w2414) -> (*(type *) &x=w2409:string)  [unwired: 1 in]
                              n870 = Unbundle By Name(w2410) -> ("TripInt.TripInt.TripInt"=w2403:dbl, "TripInt.TripInt#HighEU.TripInt#HighEU"=w2402:dbl, "TripInt.TripInt#LowEU.TripInt#LowEU"=w2401:dbl, "TripInt.TripInt#Multiplier"=w2400:dbl)
                              n871 = call "CAEN_HVSystem.EUString2UnitMultilier.vi"("EU String"=w2409) -> ("Multiplier"=w2399:dbl, "Unit"=w2408:string)  [unwired: 2 in, 1 out]
                              n872 = Build Array(w2403, w2402, w2401) -> (w2405:dbl[])
                              n873 = Divide(x=w2405, y=w2400) -> (x/y=w2404:dbl[])
                              n874 = Multiply(x=w2404, y=w2399) -> (x*y=w2406:dbl[])
                              n875 = Index Array(array=w2406, index #1=0 ("index")) -> (element #1=w2398:dbl, element #2=w2397:dbl, element #3=w2396:dbl)  [unwired: 2 in]
                              n876 = Bundle By Name(cluster=w2410, "TripInt.TripInt.TripInt"=w2398, "TripInt.TripInt#HighEU.TripInt#HighEU"=w2397, "TripInt.TripInt#LowEU.TripInt#LowEU"=w2396, "TripInt.TripInt#Multiplier"=w2399, "TripInt.TripInt#EU.DIM Status.quality"=w2413, "TripInt.TripInt#EU.DIM Status.Time Stamp"=w2412, "TripInt.TripInt#EU.TripInt#EU"=w2408, "TripInt.TripInt#EU.DIM Status.no link"=w2411) -> (w2415:T11)
                            }
                          }
                        }
                        frame "TripInt#HighEU" {
                          n877 = case "no link?" shown="False" w2421 {
                            selector: w2421 -> [w2422 w2431]
                            tunnel: [w2426 w2436] -> w2417
                            tunnel: w2419 -> [_ w2435]
                            tunnel: w2418 -> [w2425 w2430]
                            tunnel: w2420 -> [w2424 w2433]
                            tunnel: w2416 -> [w2423 w2432]
                            frame True {
                              n878 = Bundle By Name(cluster=w2425, "TripInt.TripInt#HighEU.DIM Status.quality"=w2424, "TripInt.TripInt#HighEU.DIM Status.Time Stamp"=w2423, "TripInt.TripInt#HighEU.DIM Status.no link"=w2422) -> (w2426:T11)
                            }
                            frame False {
                              n879 = Type Cast(type=0.0, x=w2435) -> (*(type *) &x=w2434:dbl)
                              n880 = Unbundle By Name(w2430) -> ("TripInt.TripInt#Multiplier"=w2427:dbl)
                              n881 = Multiply(x=w2427, y=w2434) -> (x*y=w2428:dbl)
                              n882 = Bundle By Name(cluster=w2430, "TripInt.TripInt#HighEU.DIM Status.quality"=w2433, "TripInt.TripInt#HighEU.DIM Status.Time Stamp"=w2432, "TripInt.TripInt#HighEU.TripInt#HighEU"=w2428, "TripInt.TripInt#HighEU.DIM Status.no link"=w2431) -> (w2436:T11)
                            }
                          }
                        }
                        frame "TripInt#LowEU" {
                          n883 = case "no link?" shown="False" w2442 {
                            selector: w2442 -> [w2443 w2452]
                            tunnel: [w2447 w2457] -> w2438
                            tunnel: w2440 -> [_ w2456]
                            tunnel: w2439 -> [w2446 w2451]
                            tunnel: w2441 -> [w2445 w2454]
                            tunnel: w2437 -> [w2444 w2453]
                            frame True {
                              n884 = Bundle By Name(cluster=w2446, "TripInt.TripInt#LowEU.DIM Status.quality"=w2445, "TripInt.TripInt#LowEU.DIM Status.Time Stamp"=w2444, "TripInt.TripInt#LowEU.DIM Status.no link"=w2443) -> (w2447:T11)
                            }
                            frame False {
                              n885 = Type Cast(type=0.0, x=w2456) -> (*(type *) &x=w2455:dbl)
                              n886 = Unbundle By Name(w2451) -> ("TripInt.TripInt#Multiplier"=w2448:dbl)
                              n887 = Multiply(x=w2448, y=w2455) -> (x*y=w2449:dbl)
                              n888 = Bundle By Name(cluster=w2451, "TripInt.TripInt#LowEU.DIM Status.quality"=w2454, "TripInt.TripInt#LowEU.DIM Status.Time Stamp"=w2453, "TripInt.TripInt#LowEU.TripInt#LowEU"=w2449, "TripInt.TripInt#LowEU.DIM Status.no link"=w2452) -> (w2457:T11)
                            }
                          }
                        }
                        frame "V0Set" {
                          n889 = case "no link?" shown="True" w2463 {
                            selector: w2463 -> [w2466 w2474]
                            tunnel: [w2468 w2478] -> w2459
                            tunnel: w2461 -> [_ w2477]
                            tunnel: w2460 -> [w2465 w2473]
                            tunnel: w2462 -> [w2464 w2469]
                            tunnel: w2458 -> [w2467 w2475]
                            frame True {
                              n890 = Bundle By Name(cluster=w2465, "V0Set.V0Set.DIM Status.quality"=w2464, "V0Set.V0Set.DIM Status.Time Stamp"=w2467, "V0Set.V0Set.DIM Status.no link"=w2466) -> (w2468:T11)
                            }
                            frame False {
                              n891 = Type Cast(type=0.0, x=w2477) -> (*(type *) &x=w2476:dbl)
                              n892 = Unbundle By Name(w2473) -> ("V0Set.V0Set#Multiplier"=w2471:dbl)
                              n893 = Multiply(x=w2471, y=w2476) -> (x*y=w2470:dbl)
                              n894 = Bundle By Name(cluster=w2473, "V0Set.V0Set.DIM Status.quality"=w2469, "V0Set.V0Set.DIM Status.Time Stamp"=w2475, "V0Set.V0Set.V0Set"=w2470, "V0Set.V0Set.DIM Status.no link"=w2474) -> (w2478:T11)
                            }
                          }
                        }
                        frame "V0Set#EU" {
                          n895 = case "no link?" shown="False" w2484 {
                            selector: w2484 -> [w2485 w2505]
                            tunnel: [w2489 w2509] -> w2480
                            tunnel: w2482 -> [_ w2508]
                            tunnel: w2481 -> [w2488 w2504]
                            tunnel: w2483 -> [w2487 w2507]
                            tunnel: w2479 -> [w2486 w2506]
                            frame True {
                              n896 = Bundle By Name(cluster=w2488, "V0Set.V0Set#EU.DIM Status.quality"=w2487, "V0Set.V0Set#EU.DIM Status.Time Stamp"=w2486, "V0Set.V0Set#EU.DIM Status.no link"=w2485) -> (w2489:T11)
                            }
                            frame False {
                              n897 = Type Cast(x=w2508) -> (*(type *) &x=w2503:string)  [unwired: 1 in]
                              n898 = Unbundle By Name(w2504) -> ("V0Set.V0Set.V0Set"=w2497:dbl, "V0Set.V0Set#HighEU.V0Set#HighEU"=w2496:dbl, "V0Set.V0Set#LowEU.V0Set#LowEU"=w2495:dbl, "V0Set.V0Set#Multiplier"=w2494:dbl)
                              n899 = call "CAEN_HVSystem.EUString2UnitMultilier.vi"("EU String"=w2503) -> ("Multiplier"=w2493:dbl, "Unit"=w2502:string)  [unwired: 2 in, 1 out]
                              n900 = Build Array(w2497, w2496, w2495) -> (w2499:dbl[])
                              n901 = Divide(x=w2499, y=w2494) -> (x/y=w2498:dbl[])
                              n902 = Multiply(x=w2498, y=w2493) -> (x*y=w2500:dbl[])
                              n903 = Index Array(array=w2500, index #1=0 ("index")) -> (element #1=w2492:dbl, element #2=w2491:dbl, element #3=w2490:dbl)  [unwired: 2 in]
                              n904 = Bundle By Name(cluster=w2504, "V0Set.V0Set.V0Set"=w2492, "V0Set.V0Set#HighEU.V0Set#HighEU"=w2491, "V0Set.V0Set#LowEU.V0Set#LowEU"=w2490, "V0Set.V0Set#Multiplier"=w2493, "V0Set.V0Set#EU.DIM Status.quality"=w2507, "V0Set.V0Set#EU.DIM Status.Time Stamp"=w2506, "V0Set.V0Set#EU.V0Set#EU"=w2502, "V0Set.V0Set#EU.DIM Status.no link"=w2505) -> (w2509:T11)
                            }
                          }
                        }
                        frame "V0Set#HighEU" {
                          n905 = case "no link?" shown="True" w2515 {
                            selector: w2515 -> [w2516 w2525]
                            tunnel: [w2520 w2530] -> w2511
                            tunnel: w2513 -> [_ w2529]
                            tunnel: w2512 -> [w2519 w2524]
                            tunnel: w2514 -> [w2518 w2527]
                            tunnel: w2510 -> [w2517 w2526]
                            frame True {
                              n906 = Bundle By Name(cluster=w2519, "V0Set.V0Set#HighEU.DIM Status.quality"=w2518, "V0Set.V0Set#HighEU.DIM Status.Time Stamp"=w2517, "V0Set.V0Set#HighEU.DIM Status.no link"=w2516) -> (w2520:T11)
                            }
                            frame False {
                              n907 = Type Cast(type=0.0, x=w2529) -> (*(type *) &x=w2528:dbl)
                              n908 = Unbundle By Name(w2524) -> ("V0Set.V0Set#Multiplier"=w2521:dbl)
                              n909 = Multiply(x=w2521, y=w2528) -> (x*y=w2522:dbl)
                              n910 = Bundle By Name(cluster=w2524, "V0Set.V0Set#HighEU.DIM Status.quality"=w2527, "V0Set.V0Set#HighEU.DIM Status.Time Stamp"=w2526, "V0Set.V0Set#HighEU.V0Set#HighEU"=w2522, "V0Set.V0Set#HighEU.DIM Status.no link"=w2525) -> (w2530:T11)
                            }
                          }
                        }
                        frame "V0Set#LowEU" {
                          n911 = case "no link?" shown="False" w2536 {
                            selector: w2536 -> [w2537 w2546]
                            tunnel: [w2541 w2551] -> w2532
                            tunnel: w2534 -> [_ w2550]
                            tunnel: w2533 -> [w2540 w2545]
                            tunnel: w2535 -> [w2539 w2548]
                            tunnel: w2531 -> [w2538 w2547]
                            frame True {
                              n912 = Bundle By Name(cluster=w2540, "V0Set.V0Set#LowEU.DIM Status.quality"=w2539, "V0Set.V0Set#LowEU.DIM Status.Time Stamp"=w2538, "V0Set.V0Set#LowEU.DIM Status.no link"=w2537) -> (w2541:T11)
                            }
                            frame False {
                              n913 = Type Cast(type=0.0, x=w2550) -> (*(type *) &x=w2549:dbl)
                              n914 = Unbundle By Name(w2545) -> ("V0Set.V0Set#Multiplier"=w2542:dbl)
                              n915 = Multiply(x=w2542, y=w2549) -> (x*y=w2543:dbl)
                              n916 = Bundle By Name(cluster=w2545, "V0Set.V0Set#LowEU.DIM Status.quality"=w2548, "V0Set.V0Set#LowEU.DIM Status.Time Stamp"=w2547, "V0Set.V0Set#LowEU.V0Set#LowEU"=w2543, "V0Set.V0Set#LowEU.DIM Status.no link"=w2546) -> (w2551:T11)
                            }
                          }
                        }
                        frame "V1Set" {
                          n917 = case "no link?" shown="False" w2557 {
                            selector: w2557 -> [w2560 w2568]
                            tunnel: [w2562 w2572] -> w2553
                            tunnel: w2555 -> [_ w2571]
                            tunnel: w2554 -> [w2559 w2567]
                            tunnel: w2556 -> [w2558 w2563]
                            tunnel: w2552 -> [w2561 w2569]
                            frame True {
                              n918 = Bundle By Name(cluster=w2559, "V1Set.V1Set.DIM Status.quality"=w2558, "V1Set.V1Set.DIM Status.Time Stamp"=w2561, "V1Set.V1Set.DIM Status.no link"=w2560) -> (w2562:T11)
                            }
                            frame False {
                              n919 = Type Cast(type=0.0, x=w2571) -> (*(type *) &x=w2570:dbl)
                              n920 = Unbundle By Name(w2567) -> ("V1Set.V1Set#Multiplier"=w2565:dbl)
                              n921 = Multiply(x=w2565, y=w2570) -> (x*y=w2564:dbl)
                              n922 = Bundle By Name(cluster=w2567, "V1Set.V1Set.DIM Status.quality"=w2563, "V1Set.V1Set.DIM Status.Time Stamp"=w2569, "V1Set.V1Set.V1Set"=w2564, "V1Set.V1Set.DIM Status.no link"=w2568) -> (w2572:T11)
                            }
                          }
                        }
                        frame "V1Set#EU" {
                          n923 = case "no link?" shown="False" w2578 {
                            selector: w2578 -> [w2579 w2599]
                            tunnel: [w2583 w2603] -> w2574
                            tunnel: w2576 -> [_ w2602]
                            tunnel: w2575 -> [w2582 w2598]
                            tunnel: w2577 -> [w2581 w2601]
                            tunnel: w2573 -> [w2580 w2600]
                            frame True {
                              n924 = Bundle By Name(cluster=w2582, "V1Set.V1Set#EU.DIM Status.quality"=w2581, "V1Set.V1Set#EU.DIM Status.Time Stamp"=w2580, "V1Set.V1Set#EU.DIM Status.no link"=w2579) -> (w2583:T11)
                            }
                            frame False {
                              n925 = Type Cast(x=w2602) -> (*(type *) &x=w2597:string)  [unwired: 1 in]
                              n926 = Unbundle By Name(w2598) -> ("V1Set.V1Set.V1Set"=w2591:dbl, "V1Set.V1Set#HighEU.V1Set#HighEU"=w2590:dbl, "V1Set.V1Set#LowEU.V1Set#LowEU"=w2589:dbl, "V1Set.V1Set#Multiplier"=w2588:dbl)
                              n927 = call "CAEN_HVSystem.EUString2UnitMultilier.vi"("EU String"=w2597) -> ("Multiplier"=w2587:dbl, "Unit"=w2596:string)  [unwired: 2 in, 1 out]
                              n928 = Build Array(w2591, w2590, w2589) -> (w2593:dbl[])
                              n929 = Divide(x=w2593, y=w2588) -> (x/y=w2592:dbl[])
                              n930 = Multiply(x=w2592, y=w2587) -> (x*y=w2594:dbl[])
                              n931 = Index Array(array=w2594, index #1=0 ("index")) -> (element #1=w2586:dbl, element #2=w2585:dbl, element #3=w2584:dbl)  [unwired: 2 in]
                              n932 = Bundle By Name(cluster=w2598, "V1Set.V1Set.V1Set"=w2586, "V1Set.V1Set#HighEU.V1Set#HighEU"=w2585, "V1Set.V1Set#LowEU.V1Set#LowEU"=w2584, "V1Set.V1Set#Multiplier"=w2587, "V1Set.V1Set#EU.DIM Status.quality"=w2601, "V1Set.V1Set#EU.DIM Status.Time Stamp"=w2600, "V1Set.V1Set#EU.V1Set#EU"=w2596, "V1Set.V1Set#EU.DIM Status.no link"=w2599) -> (w2603:T11)
                            }
                          }
                        }
                        frame "V1Set#HighEU" {
                          n933 = case "no link?" shown="True" w2609 {
                            selector: w2609 -> [w2610 w2619]
                            tunnel: [w2614 w2624] -> w2605
                            tunnel: w2607 -> [_ w2623]
                            tunnel: w2606 -> [w2613 w2618]
                            tunnel: w2608 -> [w2612 w2621]
                            tunnel: w2604 -> [w2611 w2620]
                            frame True {
                              n934 = Bundle By Name(cluster=w2613, "V1Set.V1Set#HighEU.DIM Status.quality"=w2612, "V1Set.V1Set#HighEU.DIM Status.Time Stamp"=w2611, "V1Set.V1Set#HighEU.DIM Status.no link"=w2610) -> (w2614:T11)
                            }
                            frame False {
                              n935 = Type Cast(type=0.0, x=w2623) -> (*(type *) &x=w2622:dbl)
                              n936 = Unbundle By Name(w2618) -> ("V1Set.V1Set#Multiplier"=w2615:dbl)
                              n937 = Multiply(x=w2615, y=w2622) -> (x*y=w2616:dbl)
                              n938 = Bundle By Name(cluster=w2618, "V1Set.V1Set#HighEU.DIM Status.quality"=w2621, "V1Set.V1Set#HighEU.DIM Status.Time Stamp"=w2620, "V1Set.V1Set#HighEU.V1Set#HighEU"=w2616, "V1Set.V1Set#HighEU.DIM Status.no link"=w2619) -> (w2624:T11)
                            }
                          }
                        }
                        frame "V1Set#LowEU" {
                          n939 = case "no link?" shown="False" w2630 {
                            selector: w2630 -> [w2631 w2640]
                            tunnel: [w2635 w2645] -> w2626
                            tunnel: w2628 -> [_ w2644]
                            tunnel: w2627 -> [w2634 w2639]
                            tunnel: w2629 -> [w2633 w2642]
                            tunnel: w2625 -> [w2632 w2641]
                            frame True {
                              n940 = Bundle By Name(cluster=w2634, "V1Set.V1Set#LowEU.DIM Status.quality"=w2633, "V1Set.V1Set#LowEU.DIM Status.Time Stamp"=w2632, "V1Set.V1Set#LowEU.DIM Status.no link"=w2631) -> (w2635:T11)
                            }
                            frame False {
                              n941 = Type Cast(type=0.0, x=w2644) -> (*(type *) &x=w2643:dbl)
                              n942 = Unbundle By Name(w2639) -> ("V1Set.V1Set#Multiplier"=w2636:dbl)
                              n943 = Multiply(x=w2636, y=w2643) -> (x*y=w2637:dbl)
                              n944 = Bundle By Name(cluster=w2639, "V1Set.V1Set#LowEU.DIM Status.quality"=w2642, "V1Set.V1Set#LowEU.DIM Status.Time Stamp"=w2641, "V1Set.V1Set#LowEU.V1Set#LowEU"=w2637, "V1Set.V1Set#LowEU.DIM Status.no link"=w2640) -> (w2645:T11)
                            }
                          }
                        }
                        frame "VMon" {
                          n945 = case "no link?" shown="False" w2660 {
                            selector: w2660 -> [w2668 w2696]
                            tunnel: [w2670 w2700] -> w2656
                            tunnel: w2658 -> [_ w2699]
                            tunnel: w2657 -> [w2667 w2695]
                            tunnel: w2659 -> [w2664 w2689]
                            tunnel: w2655 -> [w2669 w2697]
                            tunnel: [PSChannelBase.directionType."update actual value" ("direction") PSChannelBase.directionType."update actual value" ("direction")] -> w2654
                            tunnel: [w2666 w2691] -> w2653
                            tunnel: [PSChannelBase.serviceType."voltage" ("service") PSChannelBase.serviceType."voltage" ("service")] -> w2652
                            tunnel: [UtilityLib.valueStatus."no info available" ("quality") w2689] -> w2651
                            tunnel: w2650 -> [_ w2674]
                            tunnel: w2649 -> [_ w2673]
                            tunnel: w2648 -> [_ w2688]
                            tunnel: w2647 -> [_ w2679]
                            tunnel: [_ w2677] -> w2646
                            frame True {
                              n946 = Unbundle By Name(w2667) -> ("VMon.VMon.VMon"=w2665:dbl)
                              n947 = Bundle By Name(cluster=w2667, "VMon.VMon.DIM Status.quality"=w2664, "VMon.VMon.DIM Status.Time Stamp"=w2669, "VMon.VMon.DIM Status.no link"=w2668) -> (w2670:T11)
                              n948 = Type Cast(x=w2665) -> (*(type *) &x=w2666:string)  [unwired: 1 in]
                            }
                            frame False {
                              w2681 = -3  # Flags to keep
                              w2683 = i16 1  # InRange
                              n949 = Type Cast(type=0.0, x=w2699) -> (*(type *) &x=w2698:dbl)
                              n950 = Unbundle By Name(w2695) -> ("VMon.VMon#Multiplier"=w2693:dbl)
                              n951 = Multiply(x=w2693, y=w2698) -> (x*y=w2685:dbl)
                              n952 = call "PSChannelBase.get i attribute.vi"("i ref in"=w2674) -> ("i attribute"=w2675:T14)  [unwired: 16 in, 2 out]
                              n953 = Unbundle By Name(w2675) -> ("nomValues.voltage"=w2672:dbl[])
                              n954 = Index Array(array=w2672, index=w2673) -> (element=w2671:dbl)
                              n955 = Add(x=w2688, y=w2671) -> (x+y=w2687:dbl)
                              n956 = Subtract(x=w2671, y=w2688) -> (x-y=w2686:dbl)
                              n957 = In Range and Coerce(upper limit=w2687, x=w2685, lower limit=w2686) -> (In Range?=w2680:bool)  [unwired: 1 out]
                              n958 = And(x=w2681, y=w2679) -> (x .and. y?=w2678:i32)
                              n959 = Boolean To (0,1)(Boolean=w2680) -> (0, 1=w2684:i16)
                              n960 = Bundle By Name(cluster=w2695, "VMon.VMon.DIM Status.quality"=w2689, "VMon.VMon.DIM Status.Time Stamp"=w2697, "VMon.VMon.VMon"=w2685, "VMon.VMon.DIM Status.no link"=w2696) -> (w2700:T11)
                              n961 = Logical Shift(y=w2683, x=w2684) -> (x << y=w2682:i16)
                              n962 = To Long Integer(number=w2682) -> (32bit integer=w2676:i32)
                              n963 = Compound Arithmetic op=OR(w2676, w2678) -> (w2677:i32)
                              n964 = Type Cast(x=w2685) -> (*(type *) &x=w2691:string)  [unwired: 1 in]
                            }
                          }
                        }
                        frame "VMon#EU" {
                          n965 = case "no link?" shown="False" w2710 {
                            selector: w2710 -> [w2717 w2740]
                            tunnel: [w2720 w2743] -> w2706
                            tunnel: w2708 -> [_ w2742]
                            tunnel: w2707 -> [w2713 w2739]
                            tunnel: w2709 -> [w2719 w2721]
                            tunnel: w2705 -> [w2718 w2741]
                            tunnel: [PSChannelBase.directionType."update actual value" ("direction") PSChannelBase.directionType."update actual value" ("direction")] -> w2704
                            tunnel: [PSChannelBase.serviceType."voltage" ("service") PSChannelBase.serviceType."voltage" ("service")] -> w2703
                            tunnel: [w2711 w2722] -> w2702
                            tunnel: [UtilityLib.valueStatus."warning" ("quality") w2721] -> w2701
                            frame True {
                              n966 = Unbundle By Name(w2713) -> ("VMon.VMon.VMon"=w2712:dbl)
                              n967 = Type Cast(x=w2712) -> (*(type *) &x=w2711:string)  [unwired: 1 in]
                              n968 = Bundle By Name(cluster=w2713, "VMon.VMon#EU.DIM Status.quality"=w2719, "VMon.VMon#EU.DIM Status.Time Stamp"=w2718, "VMon.VMon#EU.DIM Status.no link"=w2717) -> (w2720:T11)
                            }
                            frame False {
                              n969 = Type Cast(x=w2742) -> (*(type *) &x=w2738:string)  [unwired: 1 in]
                              n970 = Unbundle By Name(w2739) -> ("VMon.VMon.VMon"=w2732:dbl, "VMon.VMon#HighEU.VMon#HighEU"=w2731:dbl, "VMon.VMon#LowEU.VMon#LowEU"=w2730:dbl, "VMon.VMon#Multiplier"=w2729:dbl)
                              n971 = call "CAEN_HVSystem.EUString2UnitMultilier.vi"("EU String"=w2738) -> ("Multiplier"=w2728:dbl, "Unit"=w2737:string)  [unwired: 2 in, 1 out]
                              n972 = Build Array(w2732, w2731, w2730) -> (w2734:dbl[])
                              n973 = Divide(x=w2734, y=w2729) -> (x/y=w2733:dbl[])
                              n974 = Multiply(x=w2733, y=w2728) -> (x*y=w2735:dbl[])
                              n975 = Index Array(array=w2735, index #1=0 ("index")) -> (element #1=w2723:dbl, element #2=w2727:dbl, element #3=w2726:dbl)  [unwired: 2 in]
                              n976 = Bundle By Name(cluster=w2739, "VMon.VMon.VMon"=w2723, "VMon.VMon#HighEU.VMon#HighEU"=w2727, "VMon.VMon#LowEU.VMon#LowEU"=w2726, "VMon.VMon#Multiplier"=w2728, "VMon.VMon#EU.DIM Status.quality"=w2721, "VMon.VMon#EU.DIM Status.Time Stamp"=w2741, "VMon.VMon#EU.VMon#EU"=w2737, "VMon.VMon.DIM Status.no link"=w2740) -> (w2743:T11)
                              n977 = Type Cast(x=w2723) -> (*(type *) &x=w2722:string)  [unwired: 1 in]
                            }
                          }
                        }
                        frame "VMon#HighEU" {
                          n978 = case "no link?" shown="False" w2749 {
                            selector: w2749 -> [w2750 w2759]
                            tunnel: [w2754 w2764] -> w2745
                            tunnel: w2747 -> [_ w2763]
                            tunnel: w2746 -> [w2753 w2758]
                            tunnel: w2748 -> [w2752 w2761]
                            tunnel: w2744 -> [w2751 w2760]
                            frame True {
                              n979 = Bundle By Name(cluster=w2753, "VMon.VMon#HighEU.DIM Status.quality"=w2752, "VMon.VMon#HighEU.DIM Status.Time Stamp"=w2751, "VMon.VMon#HighEU.DIM Status.no link"=w2750) -> (w2754:T11)
                            }
                            frame False {
                              n980 = Type Cast(type=0.0, x=w2763) -> (*(type *) &x=w2762:dbl)
                              n981 = Unbundle By Name(w2758) -> ("VMon.VMon#Multiplier"=w2755:dbl)
                              n982 = Multiply(x=w2755, y=w2762) -> (x*y=w2756:dbl)
                              n983 = Bundle By Name(cluster=w2758, "VMon.VMon#HighEU.DIM Status.quality"=w2761, "VMon.VMon#HighEU.DIM Status.Time Stamp"=w2760, "VMon.VMon#HighEU.VMon#HighEU"=w2756, "VMon.VMon#HighEU.DIM Status.no link"=w2759) -> (w2764:T11)
                            }
                          }
                        }
                        frame "VMon#LowEU" {
                          n984 = case "no link?" shown="False" w2770 {
                            selector: w2770 -> [w2771 w2780]
                            tunnel: [w2775 w2785] -> w2766
                            tunnel: w2768 -> [_ w2784]
                            tunnel: w2767 -> [w2774 w2779]
                            tunnel: w2769 -> [w2773 w2782]
                            tunnel: w2765 -> [w2772 w2781]
                            frame True {
                              n985 = Bundle By Name(cluster=w2774, "VMon.VMon#LowEU.DIM Status.quality"=w2773, "VMon.VMon#LowEU.DIM Status.Time Stamp"=w2772, "VMon.VMon#LowEU.DIM Status.no link"=w2771) -> (w2775:T11)
                            }
                            frame False {
                              n986 = Type Cast(type=0.0, x=w2784) -> (*(type *) &x=w2783:dbl)
                              n987 = Unbundle By Name(w2779) -> ("VMon.VMon#Multiplier"=w2776:dbl)
                              n988 = Multiply(x=w2776, y=w2783) -> (x*y=w2777:dbl)
                              n989 = Bundle By Name(cluster=w2779, "VMon.VMon#LowEU.DIM Status.quality"=w2782, "VMon.VMon#LowEU.DIM Status.Time Stamp"=w2781, "VMon.VMon#LowEU.VMon#LowEU"=w2777, "VMon.VMon#LowEU.DIM Status.no link"=w2780) -> (w2785:T11)
                            }
                          }
                        }
                        frame Default {
                        }
                      }
                      n990 = Replace Array Subset(array=w1270, new element=w1269, index=w1255) -> (w1267:T10)
                      n991 = Bundle By Name(cluster=w1268, "Channel Array"=w1267) -> (w1266:T9)
                      n992 = call "CAEN_HVChannel.set modified data.vi"("i ref in"=w1253, "i attribute"=w1266, "error in (no error)"=w1256) -> ("i ref out"=w1275:refnum<vi>, "error out"=w1276:errorcluster)  [unwired: 15 in]
                    }
                    frame True {
                    }
                  }
                  n993 = Not Equal?(x=PSChannelBase.directionType."unknown" ("direction"), y=w1210) -> (x != y?=w1215:bool)
                  n994 = case shown="True" w1215 {
                    tunnel: [w1242 w1251] -> w1207
                    tunnel: w1217 -> [w1242 w1250]
                    tunnel: [w1241 w1249] -> w1208
                    tunnel: w1216 -> [w1241 w1248]
                    tunnel: w1213 -> [_ w1247]
                    tunnel: w1212 -> [_ w1246]
                    tunnel: w1211 -> [_ w1245]
                    tunnel: w1204 -> [_ w1244]
                    tunnel: w1210 -> [_ w1243]
                    frame False {
                    }
                    frame True {
                      n995 = call "PSChannelBase.update services and attribute data.vi"("i ref in"=w1250, "direction"=w1243, "service"=w1246, "value"=w1247, "error in (no error)"=w1248, "quality"=w1245, "channelNumber"=w1244) -> ("i ref out"=w1251:refnum<vi>, "error out"=w1249:errorcluster)  [unwired: 10 in, 1 out]
                    }
                  }
                  n996 = To Long Integer(number=w1201) -> (32bit integer=w1199:i32)
                  n997 = Not Equal To 0?(x=w1199) -> (x != 0?=w1209:bool)
                  n998 = Type Cast(x=w1199) -> (*(type *) &x=w1202:string)  [unwired: 1 in]
                  n999 = case shown="True" w1209 {
                    tunnel: [w1232 w1240] -> w1206
                    tunnel: w1207 -> [w1232 w1239]
                    tunnel: [w1231 w1238] -> w1205
                    tunnel: w1208 -> [w1231 w1237]
                    tunnel: w1202 -> [_ w1236]
                    tunnel: w1204 -> [_ w1235]
                    tunnel: PSChannelBase.directionType."update actual value" ("direction") -> [_ w1234]
                    tunnel: PSChannelBase.serviceType."status" ("service") -> [_ w1233]
                    frame False {
                    }
                    frame True {
                      n1000 = call "PSChannelBase.update services and attribute data.vi"("i ref in"=w1239, "direction"=w1234, "service"=w1233, "value"=w1236, "error in (no error)"=w1237, "channelNumber"=w1235) -> ("i ref out"=w1240:refnum<vi>, "error out"=w1238:errorcluster)  [unwired: 11 in, 1 out]
                    }
                  }
                }
              }
            }
            frame Error {
              n1001 = call "CoreLib.set data type mismatch.vi"("error in (no error)"=w2792) -> ("error out"=w2793:errorcluster)  [unwired: 18 in]
            }
          }
          n1002 = call "BaseProcess.set event status.vi"("i ref in"=w1164, "EventStatus"=w1161, "error in (no error)"=w1163) -> ("i ref out"=w1160:refnum<vi>, "error out"=w1162:errorcluster)  [unwired: 14 in, 1 out]
          n1003 = Unbundle By Name(w1162) -> ("source"=w1157:string, "code"=w1168:i32)
          n1004 = call-poly "CoreLib.data 2 byte array.vi"("string"=w1157) -> ("byteArray out"=w1165:T1)  [unwired: 18 in]
          n1005 = Bundle By Name(cluster=w1167, "Data"=w1165, "Error #"=w1168, "Data Descriptor"="C:N") -> (w1166:T2)
        }
      }
      n1006 = case "Default?" shown="False" w13 {
        tunnel: w12 -> [w21 _]
        tunnel: w11 -> [w20 _]
        frame False {
          n1007 = call "DeviceBase.set device state.vi"("i ref in"=w20, "implicit"=TRUE, "device error"=w21) -> ()  [unwired: 14 in, 3 out]
        }
        frame True {
        }
      }
    }
    frame Error {
    }
  }
  "answer cluster" <- w8
  "i ref out" <- w4
  "error out" <- w3
